vi "Main HMI.vi"() -> ()   [LabVIEW 2023]
uses:
  <instrlib>/HPS-17000/Client Facing Datatypes/Limits.ctl
  Types/Function.ctl
  Types/Mode.ctl
  Types/Range.ctl
  Types/Setpoints.ctl
  <instrlib>/HPS-17000/Client Facing Datatypes/DeviceProperties.ctl
  Types/EIS Mode.ctl
  <vilib>/HPS-17000/nibatterycycler_grpc_Setpoint.ctl
  Classes/Grapher_class/Grapher.lvclass
  Streamer_class/Streamer.lvclass
  Logger_class/Logger.lvclass
  Script_class/Script.lvclass
  <instrlib>/HPS-17000/HPS-17000.lvclass
  <instrlib>/HPS-17000/Client Facing Datatypes/Multi-Cycler Events.ctl
  <instrlib>/HPS-17000/Client Facing Datatypes/Heartbeat Event Data.ctl
  <instrlib>/HPS-17000/Client Facing Datatypes/Faults Event Data.ctl
  <instrlib>/HPS-17000/Client Facing Datatypes/Network Sync Event Data.ctl
  <instrlib>/HPS-17000/Client Facing Datatypes/Setpoint Stream Status Data.ctl
  <vilib>/HPS-17000/MStream_grpc_CyclerMeasurement.ctl
  Types/ERROR_GLOBAL.ctl
  <instrlib>/HPS-17000/Client Facing Datatypes/Range.ctl
  <vilib>/HPS-17000/Setpoint Stream Basic Config.ctl
  <vilib>/Utility/miscctls.llb/LVStringsAndValuesArrayTypeDef_I16.ctl
  <vilib>/addons/_JKI Toolkits/State Machine/_JKI_lib_State_Machine.llb/Select State(s)_err__jki_lib_state_machine.vi
  <vilib>/Utility/error.llb/Trim Whitespace One-Sided.vi
  <instrlib>/HPS-17000/Internal/Acknowledge Faults Multi.vi
  <instrlib>/HPS-17000/Internal/Identify Multi.vi
  <vilib>/Utility/TDMS File Viewer/TDMS - File Viewer (NXG Style).vi
  <instrlib>/HPS-17000/Internal/Get Status Multi.vi
  <instrlib>/HPS-17000/Internal/Get Faults Multi.vi
  <instrlib>/HPS-17000/Internal/Get Mode Multi.vi
  <instrlib>/HPS-17000/Internal/Get Limits Multi.vi
  <instrlib>/HPS-17000/Internal/Get Enabled Output Multi.vi
  <vilib>/Waveform/WDTOps.llb/WDT Append Waveforms DBL.vi
  <vilib>/Utility/file.llb/Write Delimited Spreadsheet (DBL).vi
  <instrlib>/HPS-17000/Internal/Find GM ID Single.vi
  <instrlib>/HPS-17000/Internal/Initialize Single.vi
  <instrlib>/HPS-17000/Internal/Initialize Multi.vi
  <instrlib>/HPS-17000/Internal/Close Multi.vi
  <instrlib>/HPS-17000/Internal/Reserve Multi.vi
  <instrlib>/HPS-17000/Internal/Unreserve Multi.vi
  <instrlib>/HPS-17000/Internal/Clear Reservation Multi.vi
  <instrlib>/HPS-17000/Internal/Clear Reservation Confirmation Multi.vi
  <instrlib>/HPS-17000/Internal/Write Setpoint Multi.vi
  <instrlib>/HPS-17000/Internal/Set Mode Multi.vi
  <instrlib>/HPS-17000/Internal/Set Limits Multi.vi
  <instrlib>/HPS-17000/Internal/Set Energized Multi.vi
  <instrlib>/HPS-17000/Internal/Set Enabled Output Multi.vi
  <instrlib>/HPS-17000/Internal/Start Measurement Stream Multi.vi
  <instrlib>/HPS-17000/Internal/Stop Measurement Stream Multi.vi
  <instrlib>/HPS-17000/Internal/Start Setpoint Stream Multi.vi
  <instrlib>/HPS-17000/Internal/Stream Setpoints Multi.vi
  <instrlib>/HPS-17000/Internal/Stop Setpoint Stream Multi.vi
  <vilib>/Utility/file.llb/Read Delimited Spreadsheet (DBL).vi
  <userlib>/_OpenG.lib/appcontrol/appcontrol.llb/openg_application_control.lvlib
  <vilib>/HPS-17000/NI_BC_client.lvlib
  <vilib>/HPS-17000/Cycler.lvclass
  <vilib>/measure/NI_MABase.lvlib
  <vilib>/Utility/TDMS File Viewer/NI_TDMS File Viewer.lvlib
panel:
  out "Charging 2":bool caption="CHARGE"
  out "Discharging":bool caption="DISCHARGE"
  in  "Cycler Selection":i16(ring) caption="CYCLER(S)" items=["ALL"=-1]
  out "EMO Indicator":u16(ring)
  in  "Start Logging":bool
  out "Function":T1=enum."STANDBY" caption="FUNCTION"
  out "MODE":u16(ring)=193 items=["UNKNOWN"=0, "CONSTANT VOLTAGE"=1, "CONSTANT CURRENT"=2, "INTERNAL RECIRCULATION"=193]
  in  "HPS Clear":bool
  out "Status Message":string
  in  "HPS Reserve":bool
  in  "HPS Connect":bool
  out "Fault Message":string
  in  "Acknowledge Faults":bool
  out "Current Range":string(combo) caption="RANGE"
  out "Voltage Range":string(combo) caption="RANGE"
  out "Power Maximum":sgl caption="MAX"
  out "Power Minimum":sgl caption="MIN"
  out "Current Maximum":sgl caption="MAX"
  out "Current Minimum":sgl caption="MIN"
  out "Voltage Maximum":sgl caption="MAX"
  out "Voltage Minimum":sgl caption="MIN"
  in  "Main Tab Control":T2(tab)=enum."CONTROL"
  out "XY Graph":T3(graph)
  in  "Use Local Time":bool caption="LOCAL TIME"
  in  "High Speed":bool caption="HIGH SPEED"
  in  "Pause Chart":bool
  in  "Save Chart":bool
  in  "Erase Chart":bool
  in  "TSN NIC IP Address":string caption="TSN NIC IP ADDRESS"
  in  "HPS Topology":enum16{"SINGLE", "MULTI"}(ring) caption="HPS17K TOPOLOGY"
  in  "Profile Step dT (ns)":i64=10000 caption="PROFILE STEP TIME (ns)"
  in  "Graph Samples":u32=10000 caption="CHART SAMPLES"
  in  "Graph Data Decimation":i32=100 caption="CHART DECIMATION"
  in  "Log File Directory":path caption="LOG FILE DIRECTORY"
  in  "Controller TSN IP":string caption="CONTROLLER TSN IP"
  in  "HPS17K Search":bool
  in  "Device Search":string(tree) caption="HPS17K SEARCH"
  in  "HPS17K IP Addresses":string[](tree) caption="HPS17K NETWORK"
  in  "Add HPS17K":bool
  in  "Remove HPS17K":bool
  in  "Apply Slew Rates":bool
  in  "Slew Rates":T4={"Voltage Inc. [V/sec]"=inf, "Voltage Dec. [V/sec]"=inf, "Current Inc. [A/sec]"=inf, "Current Dec. [A/sec]"=inf, "Resistance Inc. [Ohms/sec]"=inf, "Resistance Dec. [Ohms/sec]"=inf} caption="SLEW RATES"
  in  "Output":bool caption="OUTPUT"
  in  "Apply Setpoints":bool
  in  "Setpoints":T5 caption="SETPOINTS"
  in  "Apply Mode & Range":bool
  in  "Mode & Range":cluster{"Mode":T6, "Range":T7}={"Mode"=193, "Range"=1} caption="MODE | RANGE" {"Range" items=["Low Voltage"=1, "High Voltage"=2]; "Mode" items=["Constant Voltage"=1, "Constant Current"=2, "Internal Recirculation"=193]}
  in  "Apply Limits":bool
  in  "Limits":T8 caption="LIMITS"
  in  "Energize":bool caption="ENERGIZE"
  in  "TDMS Viewer":bool
  in  "Get Device Properties":bool
  in  "Get XC Report":bool
  out "Event Log":i32(listbox) caption="EVENT LOG"
  in  "Clear Event Log":bool
  in  "Volta Monitor":bool
  out "device properties":T9
  out "GM ID":string
  out "Measurement Stream":bool caption="MEASUREMENT STREAM"
  out "Setpoint Stream":bool caption="SETPOINT STREAM"
  out "OK":bool
  out "Heartbeat Valid":bool caption="HEARTBEAT VALID"
  in  "FC Sys Inspect":bool
  out "Fault Description":string caption="FAULT DESCRIPTION"
  in  "Start & Stop EIS Profile":bool
  in  "EIS AC Step Delay":dbl=1.0 caption="AC Step Delay (Seconds)"
  in  "EIS Samples":dbl=1000.0 caption="Samples at Frequency"
  in  "AC Signal (mV/mA RMS)":dbl=20.0
  in  "EIS DC Current":dbl caption="DC Current (A)"
  in  "EIS Delta Frequency":dbl=100.0 caption="AC Step Frequency (Hz)"
  in  "EIS Stop Frequency":dbl=500.0 caption="AC Stop Frequency (Hz)"
  in  "EIS Start Frequency":dbl=1000.0 caption="AC Start Frequency (Hz)"
  in  "EIS DC Potential":dbl=650.0 caption="DC Potential (V)"
  in  "EIS Mode":T10=2 items=["Voltage (PEIS)"=1, "Current (GEIS)"=2]
  in  "Generate EIS Profile":bool
  in  "EIS Save & Load Profile":bool
  in  "Generate EIS Report":bool
  in  "CSV Profile":path caption="CSV PROFILE"
  in  "Start Profile":bool
  out "CSV Profile":waveform(sgl)[](graph)
  out "Self Test Log":i32(listbox) caption="SELF TEST LOG"
  in  "Run Self Test":bool
  out "Test Server Log":i32(listbox) caption="TEST SERVER LOG"
  in  "Launch Test Server":bool
  in  "Voltage Reformation":bool caption="REFORMATION"
  in  "Update Temperatures":bool
  out "Temperatures":i32(listbox) caption="TEMPERATURES"
  out "Thermal Limits":i32(listbox) caption="THERMAL LIMITS"
  out "Hardware Limits":i32(listbox) caption="HARDWARE LIMITS"
  out "Fault":bool caption="FAULT"
  out "Output Enabled":bool caption="OUTPUT ENABLED"
  out "Output Disabled":bool caption="OUTPUT DISABLED"
  out "System Power":bool caption="SYSTEM POWER"
  out "POWER":dbl(knob) caption="Gauge" scale=150.0..-150.0
  out "CURRENT":dbl(knob) caption="Gauge" scale=480.0..-480.0
  out "VOLTAGE":dbl(knob) caption="Gauge"
  # "what if the graphs on the right were instead a subpanel of the new EIS active object class\n\nthat way it could show us the actual EIS profile, where it's at in the test, and other features.\n\nikt would need to communicate with teh main HMI to lock out the GUI but that is fine, the main HMI\n\nwould act as the object controller launching/destroying it for different EIS profiles.  This will run an automated test that will guarnatee full resolution for each EIS frequency sweep.  It will need to automate the logging functionality as well because this log file will be necessary to run the VI afterwards to generate the profile\n\nexpand the tabs to show more details, maybe show the FFT graph so we can pinpoint hte frequency peaks and see more intermediate FFT data that might help analysis (or at the very least help development)"
  # "generate eis profile will create a new object and embed it into the subpanel.  if one already exists, it willr emove it\n\nstart eis profile will start/stop the EIS profile active object active test sequence until it finishes or is stopped.  It will not\nenable this button until an EIS profile has been generated.\n\nthe user can also load a previous EIS data which will load the data into the EIS object for analysis\n\nthen, generate report wil take the newly generated (or loaded data previously generated) and then generate the nyquist, bode, and FFT plots for viewing.\n\nwe should also add a way to export this graph once it's generated\n\nneed to add teh subpanel"
  # "OFF               ON"
  # "OFF               ON"
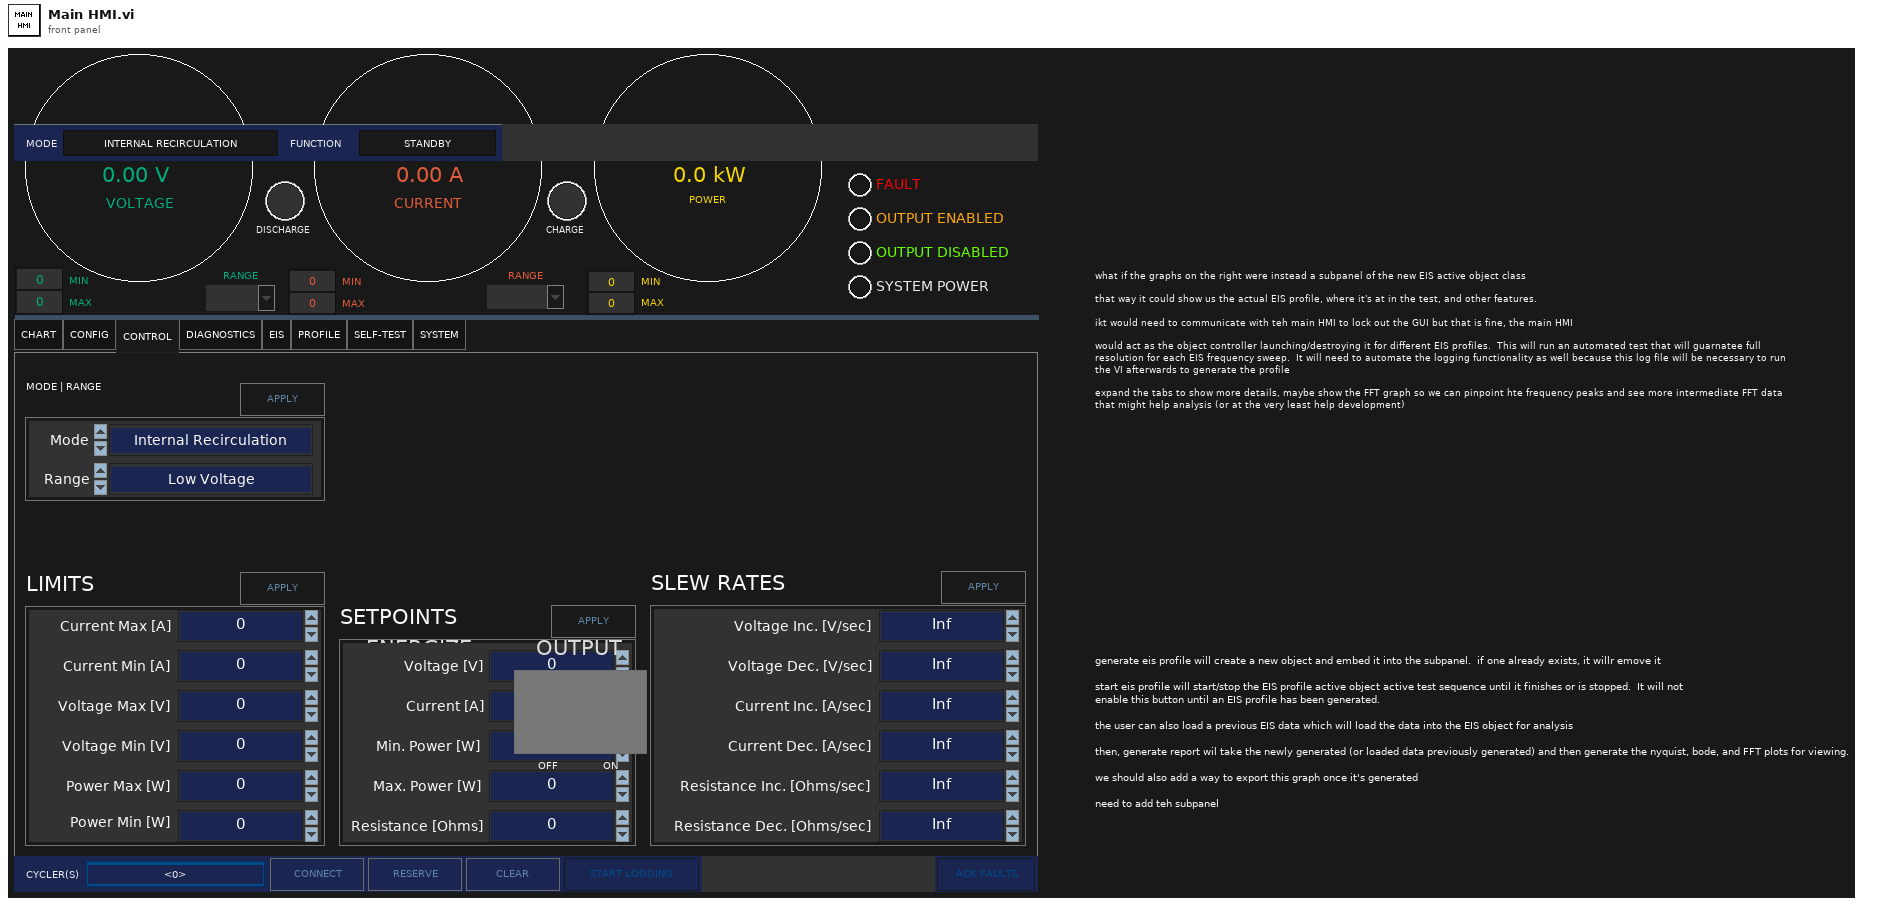
[diagram p1: front panel]
types:
  T1 = typedef "Function.ctl" = enum16{"REGEN", "STANDBY", "SUPPLY"}
  T2 = enum32{"CHART", "CONFIG", "CONTROL", "DIAGNOSTICS", "EIS", "PROFILE", "SELF-TEST", "SYSTEM"}
  T3 = cluster{"timestamp":dbl[], "setpoint current":dbl[]}[]
  T4 = cluster{"Voltage Inc. [V/sec]":sgl, "Voltage Dec. [V/sec]":sgl, "Current Inc. [A/sec]":sgl, "Current Dec. [A/sec]":sgl, "Resistance Inc. [Ohms/sec]":sgl, "Resistance Dec. [Ohms/sec]":sgl}
  T5 = typedef "Setpoints.ctl" = cluster{"Voltage":sgl, "Current":sgl, "Minimum Power":sgl, "Maximum Power":sgl, "Resistance":sgl}
  T6 = typedef "Mode.ctl" = u16
  T7 = typedef "Range.ctl" = u16
  T8 = typedef "HPS-17000.lvclass/Limits.ctl" = cluster{"Current Max Limit":sgl, "Current Min Limit":sgl, "Voltage Max Limit":sgl, "Voltage Min Limit":sgl, "Power Max Limit":sgl, "Power Min Limit":sgl}
  T9 = typedef "HPS-17000.lvclass/DeviceProperties.ctl" = cluster{"name":string, "model":string, "vendor":string, "serial_number":string}
  T10 = typedef "EIS Mode.ctl" = u16
  T11 = typedef "NI_BC_client.lvlib/nibatterycycler_grpc_Setpoint.ctl" = cluster{"voltage":sgl, "current":sgl, "min_power":sgl, "max_power":sgl, "resistance":sgl}
  T12 = typedef "HPS-17000.lvclass/Multi-Cycler Events.ctl" = cluster{"heartbeats events":refnum<user-event>[], "faults events":refnum<user-event>[], "network sync event":refnum<user-event>[], "setpoint status event":refnum<user-event>[]}
  T13 = cluster{"Core":cluster{"Current VI Reference":refnum<vi>, "Close Panel on Exit?":bool}, "Connected":bool, "Reserved":bool, "Measurement Stream":bool, "Setpoint Stream":bool, "Last Periodic Update":u32, "Profile Setpoints":T11[], "Grapher Ref":refnum<class "Grapher.lvclass">, "Streamer Ref":refnum<class "Streamer.lvclass">, "Logger Ref":refnum<class "Logger.lvclass">, "Test Server Ref":refnum<class "Script.lvclass">, "Self Test Ref":refnum<class "Script.lvclass">, "HPS17K Refs":refnum<class "HPS-17000.lvclass">[], "HPS17K Events":T12, "Self Test Completed":refnum<user-event>, "Graph Queue":refnum<queue>, "Logger Queue":refnum<queue>, "Drag Data":cluster{"data name":string, "drag data":variant}[]}
  T14 = enum8{"Enabled", "Disabled", "Disabled and Grayed Out"}
  T15 = cluster{"data name":string, "drag data":variant}[]
  T16 = enum32{"Invalid", "Standard", "Closed", "Hidden", "Minimized", "Maximized"}
  T17 = enum32{"invalid app kind", "Development System", "Run Time System", "Student Edition", "Embedded LabVIEW", "Evaluation", "Custom"}
  T18 = enum16{"open", "replace", "create", "open or create", "replace or create", "replace or create with confirmation"}
  T19 = typedef "Cycler.lvclass/Setpoint Stream Basic Config.ctl" = cluster{"local address":string, "receiver port":u16}
  T20 = cluster{"XY Graph":refnum<vi>, "Voltage":refnum<vi>, "Current":refnum<vi>, "Power":refnum<vi>, "Function":refnum<vi>}
  T21 = typedef "LVStringsAndValuesArrayTypeDef_I16.ctl" = cluster{"String":string, "Value":i16}[]
  T22 = typedef "ERROR_GLOBAL.ctl" = u32
  T23 = typedef "NI_BC_client.lvlib/MStream_grpc_CyclerMeasurement.ctl" = cluster{"measured_voltage":sgl, "measured_current":sgl, "setpoint_voltage":sgl, "setpoint_current":sgl, "timestamp":i64}
  T24 = cluster{"Current VI Reference":refnum<vi>, "Close Panel on Exit?":bool}
  T25 = typedef "HPS-17000.lvclass/Range.ctl" = u8
  T26 = typedef "HPS-17000.lvclass/Mode.ctl" = u8
  T27 = typedef "HPS-17000.lvclass/Events.ctl" = cluster{"heartbeat failure event":refnum<user-event>, "faults event":refnum<user-event>, "network sync event":refnum<user-event>, "setpoint status event":refnum<user-event>}
  T28 = cluster{"[0]":dbl, "[1]":dbl, "[2]":dbl, "[3]":dbl, "[4]":dbl, "[5]":dbl}
  T29 = cluster{"[0]":dbl, "[1]":dbl, "[2]":dbl, "[3]":dbl, "[4]":dbl}
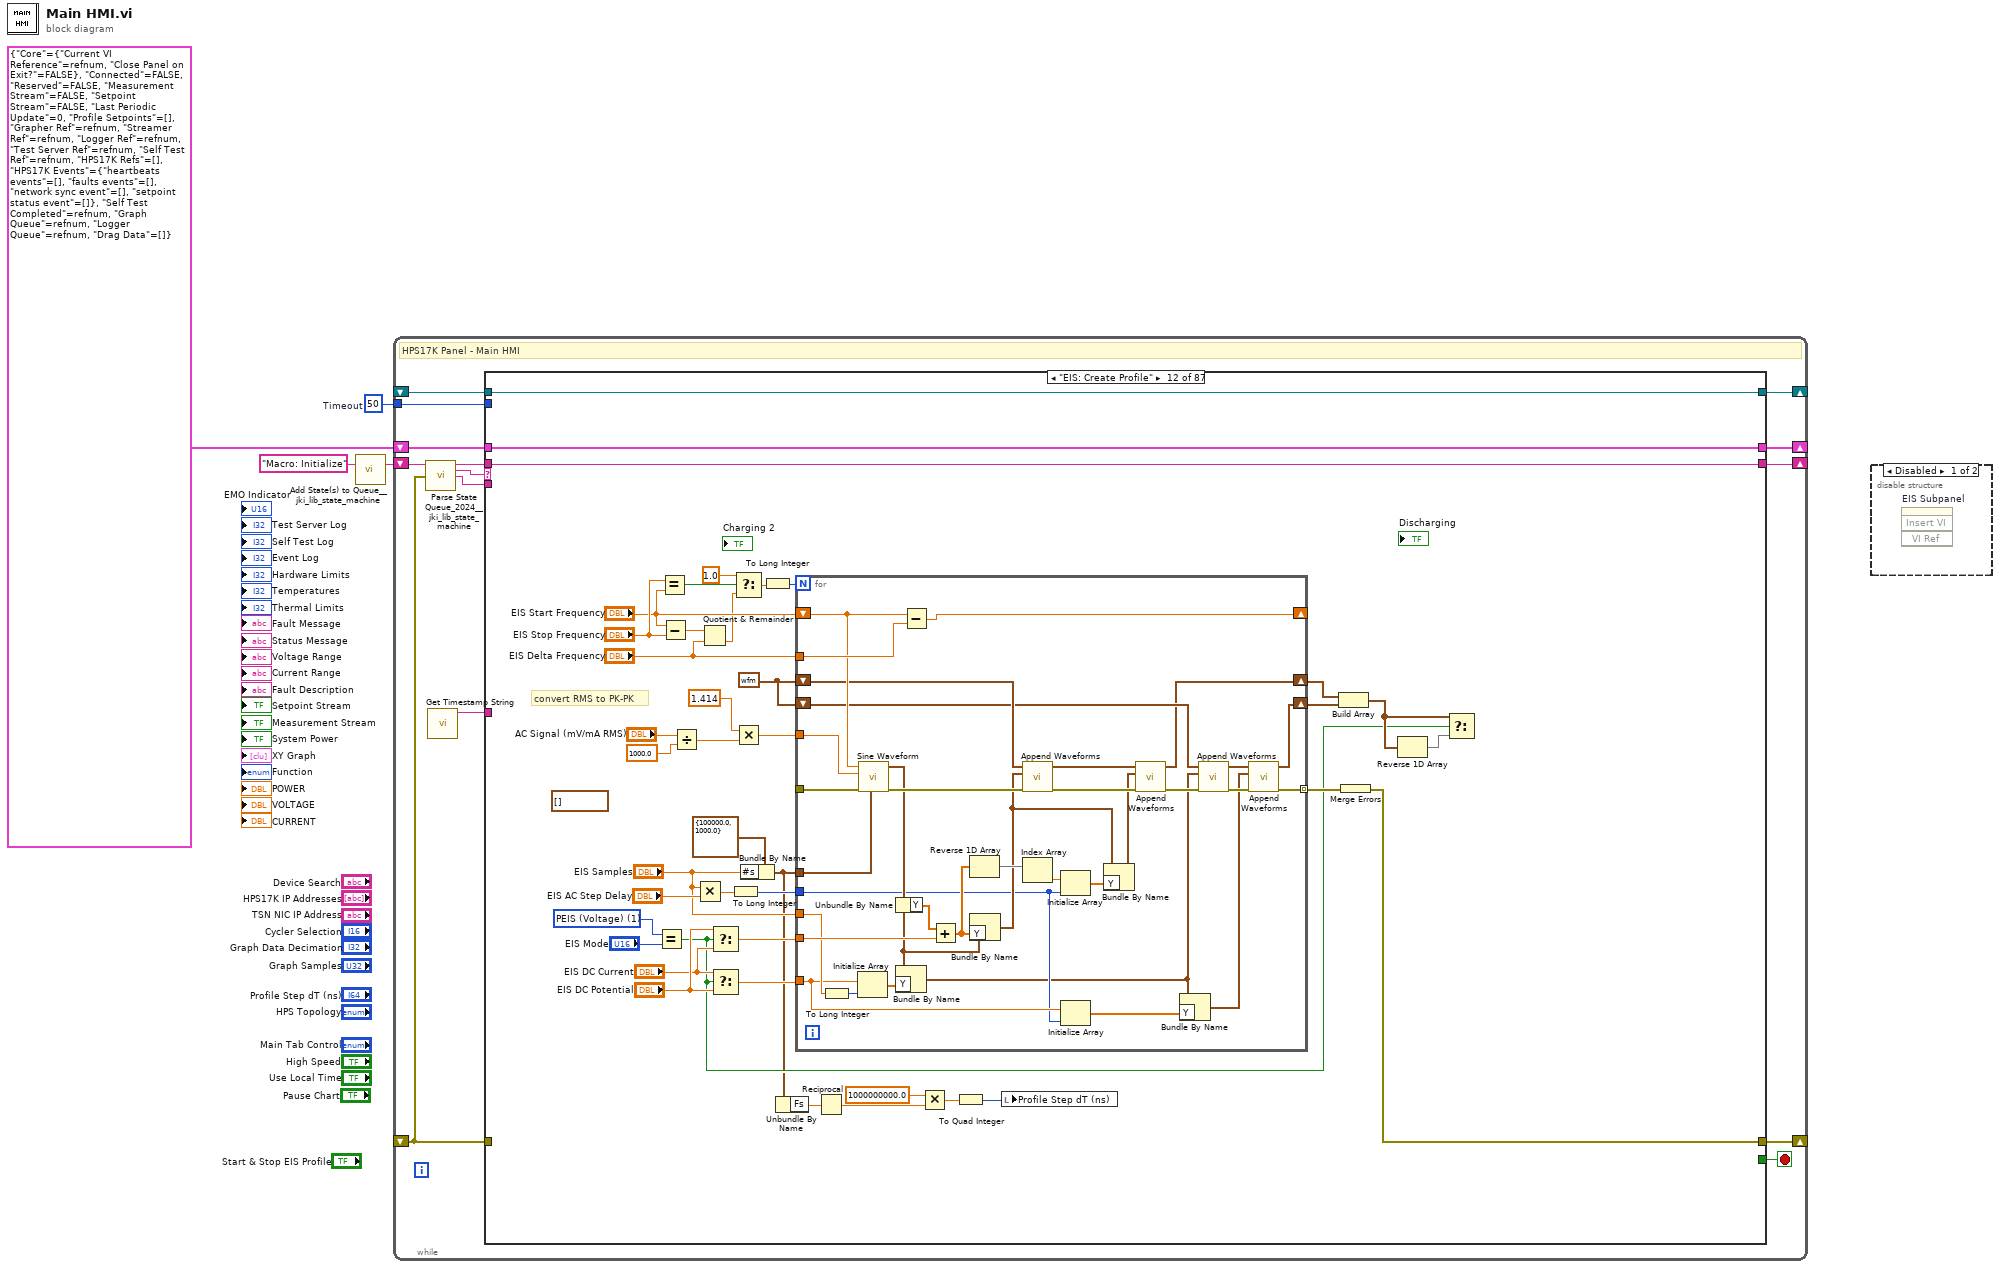
[diagram p0: block diagram]
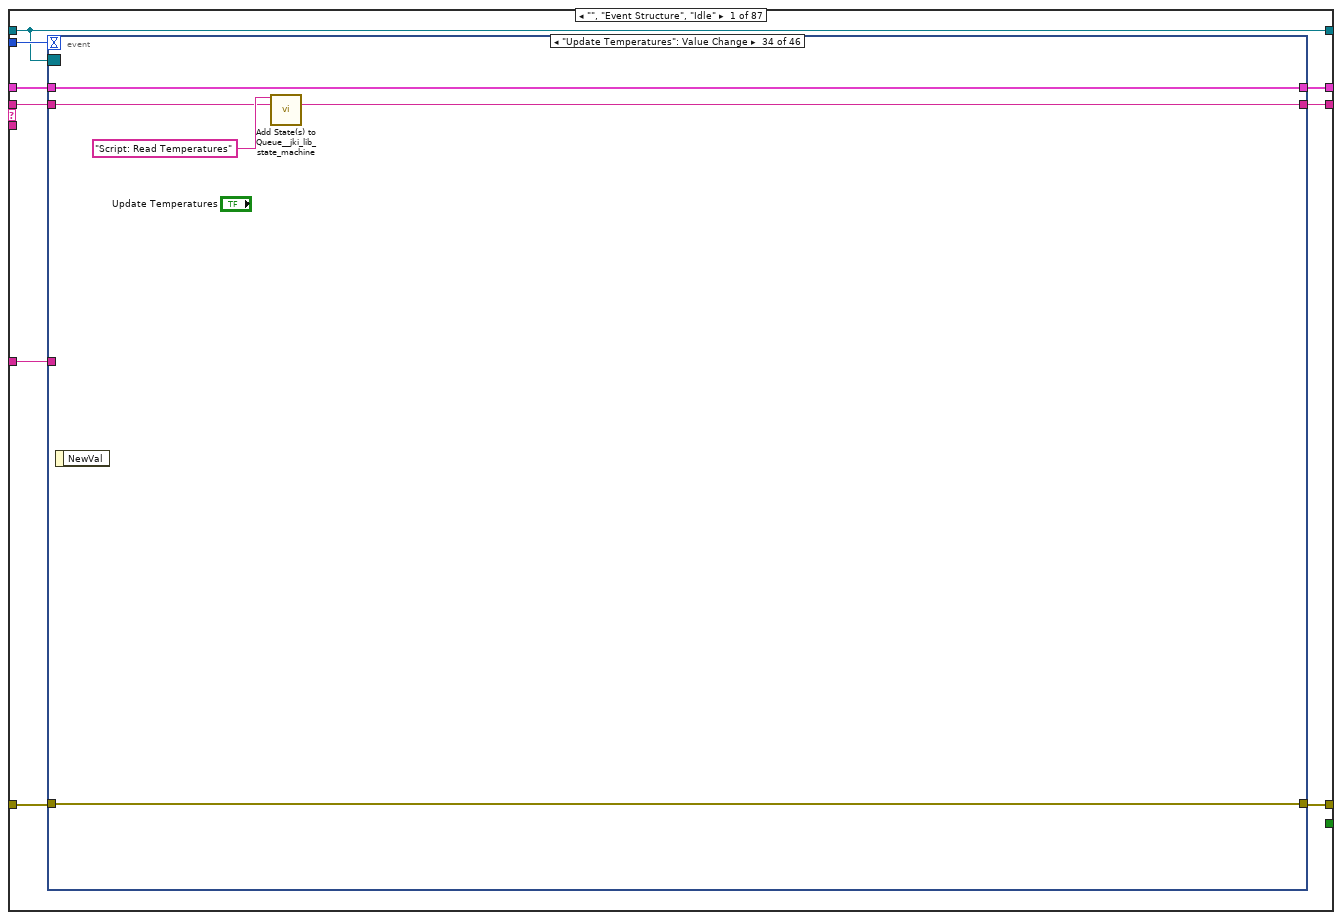
[diagram p3: hidden frame]
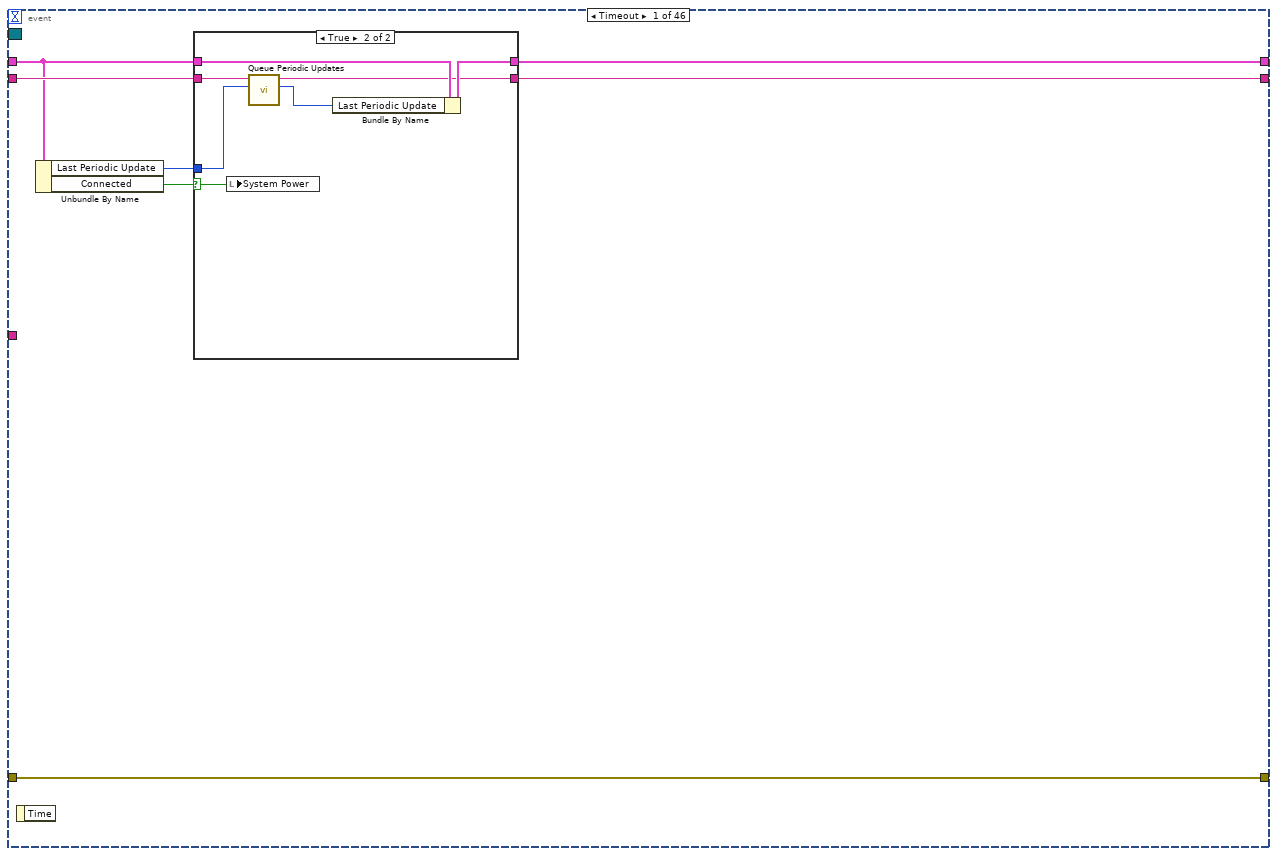
[diagram p4: hidden frame]
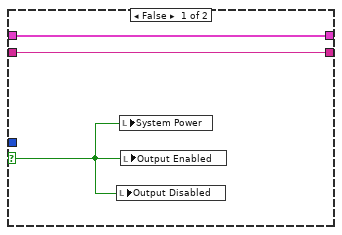
[diagram p5: hidden frame]
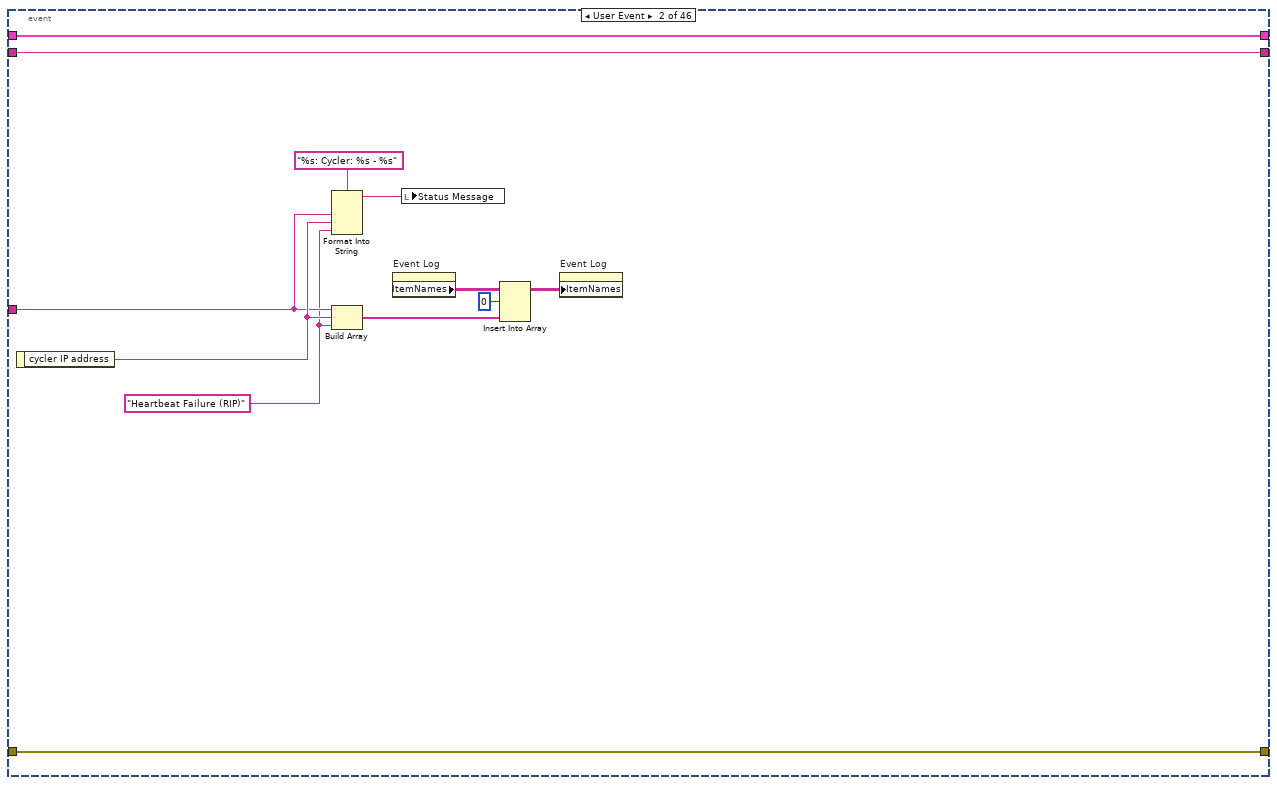
[diagram p6: hidden frame]
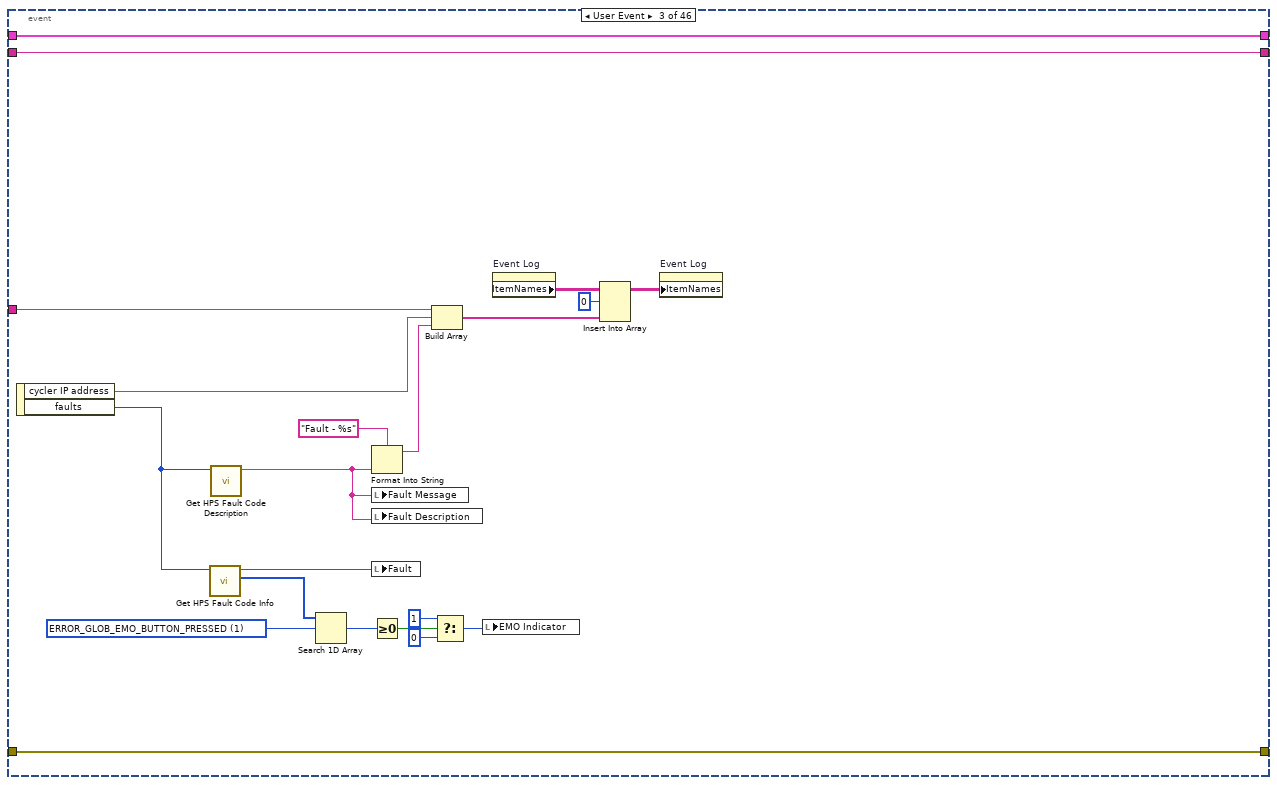
[diagram p7: hidden frame]
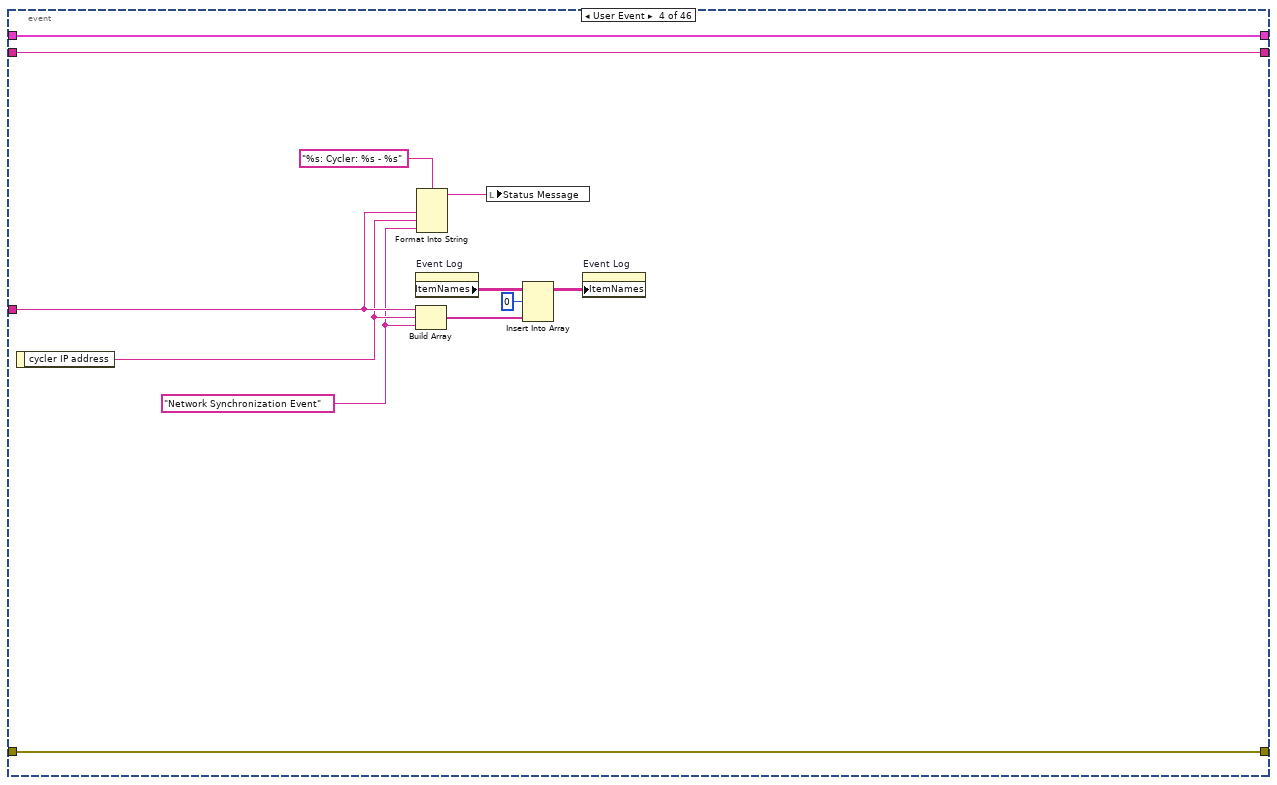
[diagram p8: hidden frame]
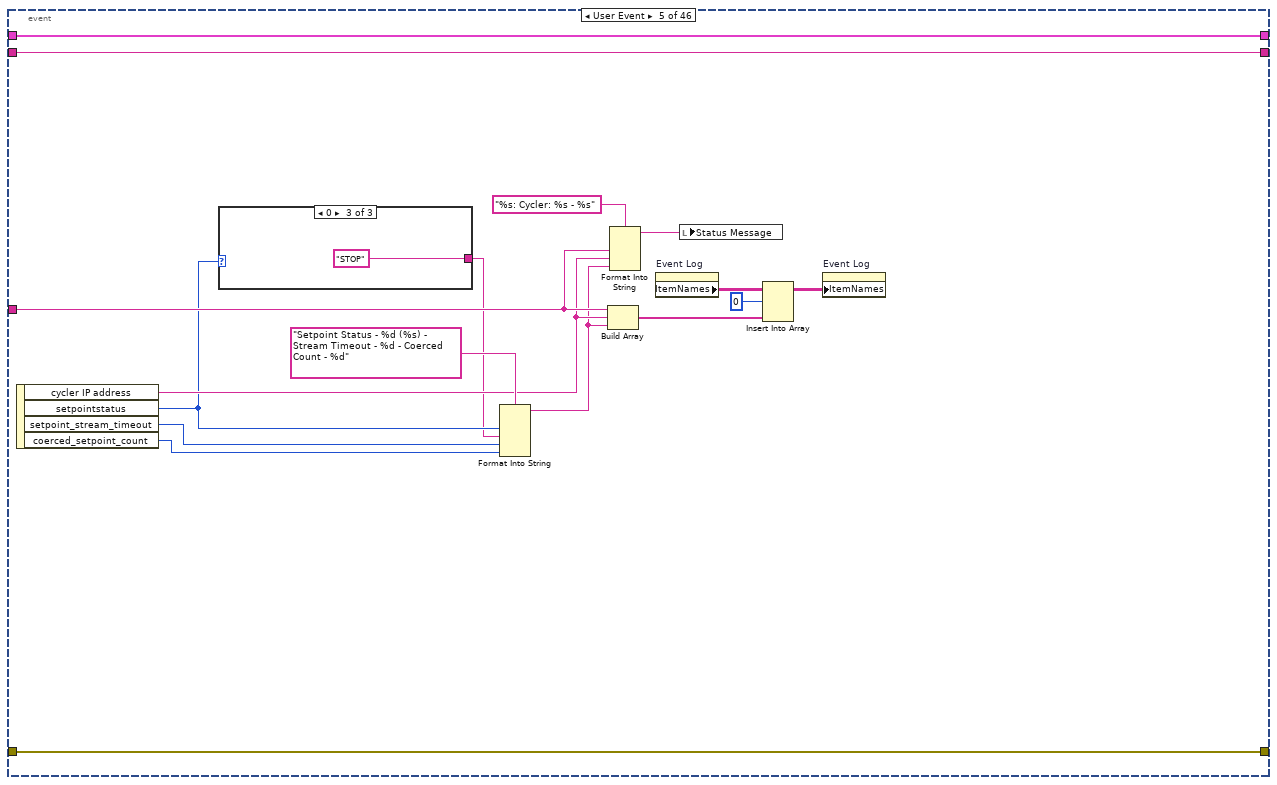
[diagram p9: hidden frame]
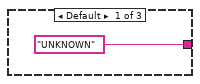
[diagram p10: hidden frame]
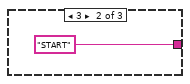
[diagram p11: hidden frame]
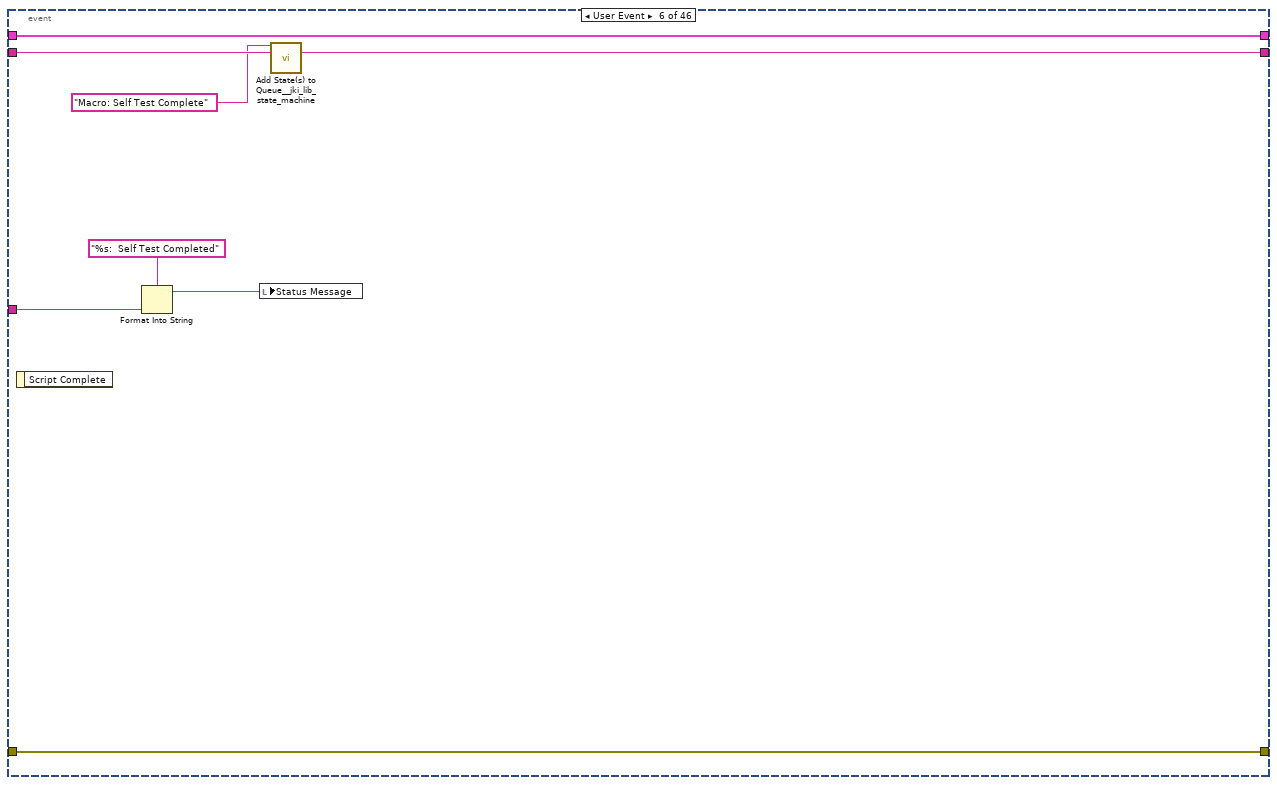
[diagram p12: hidden frame]
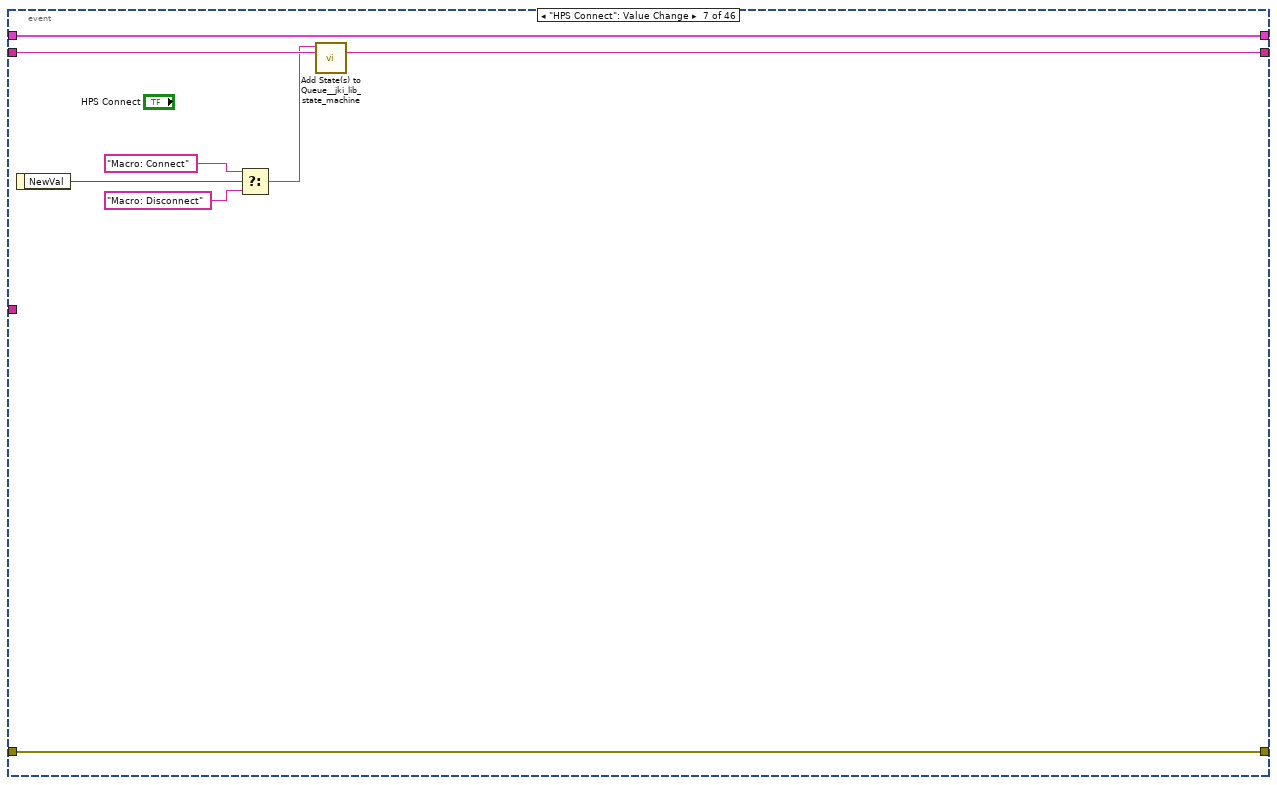
[diagram p13: hidden frame]
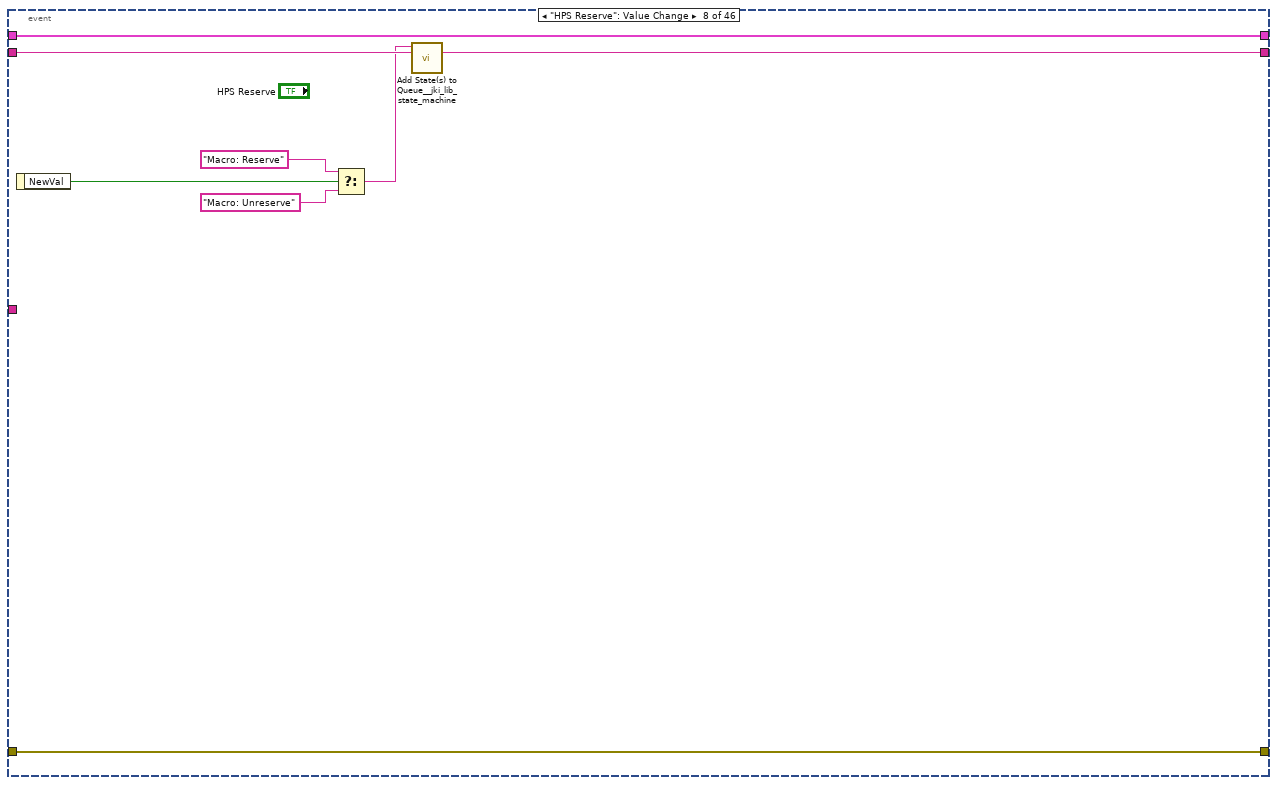
[diagram p14: hidden frame]
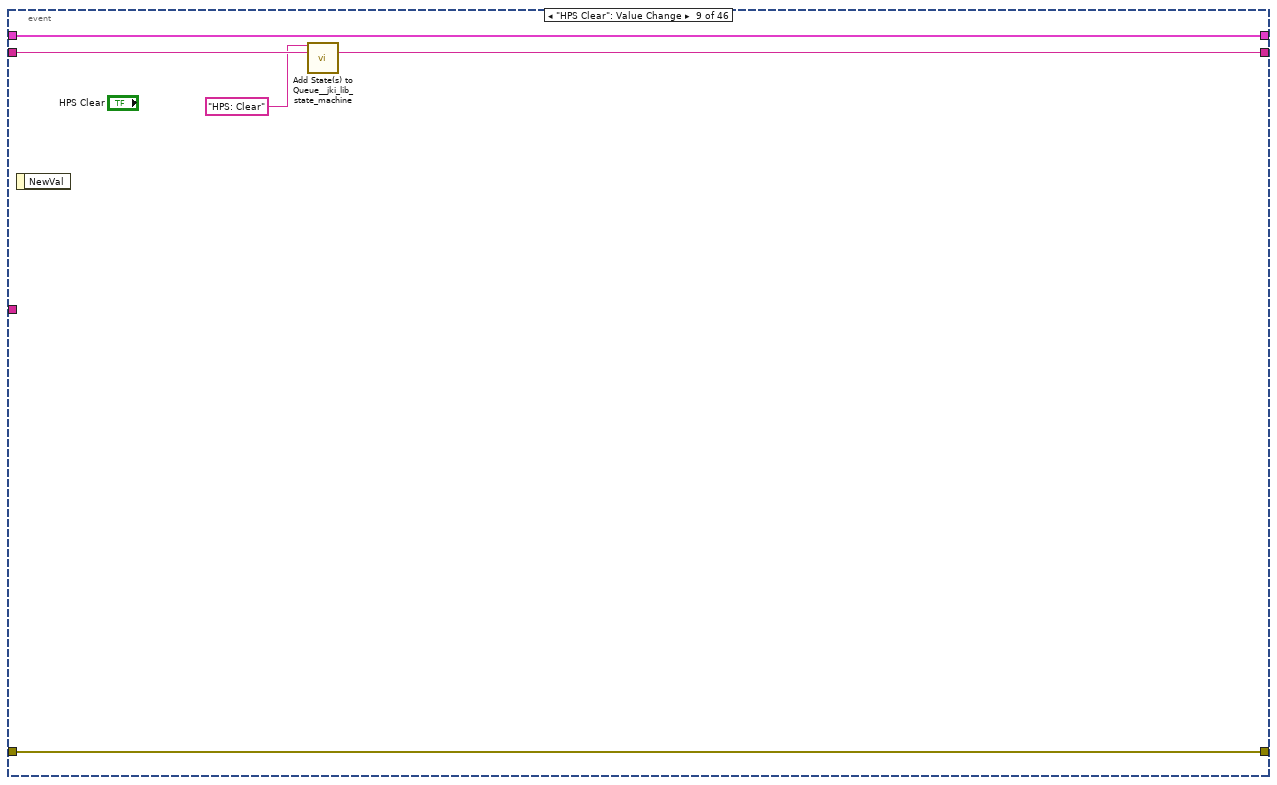
[diagram p15: hidden frame]
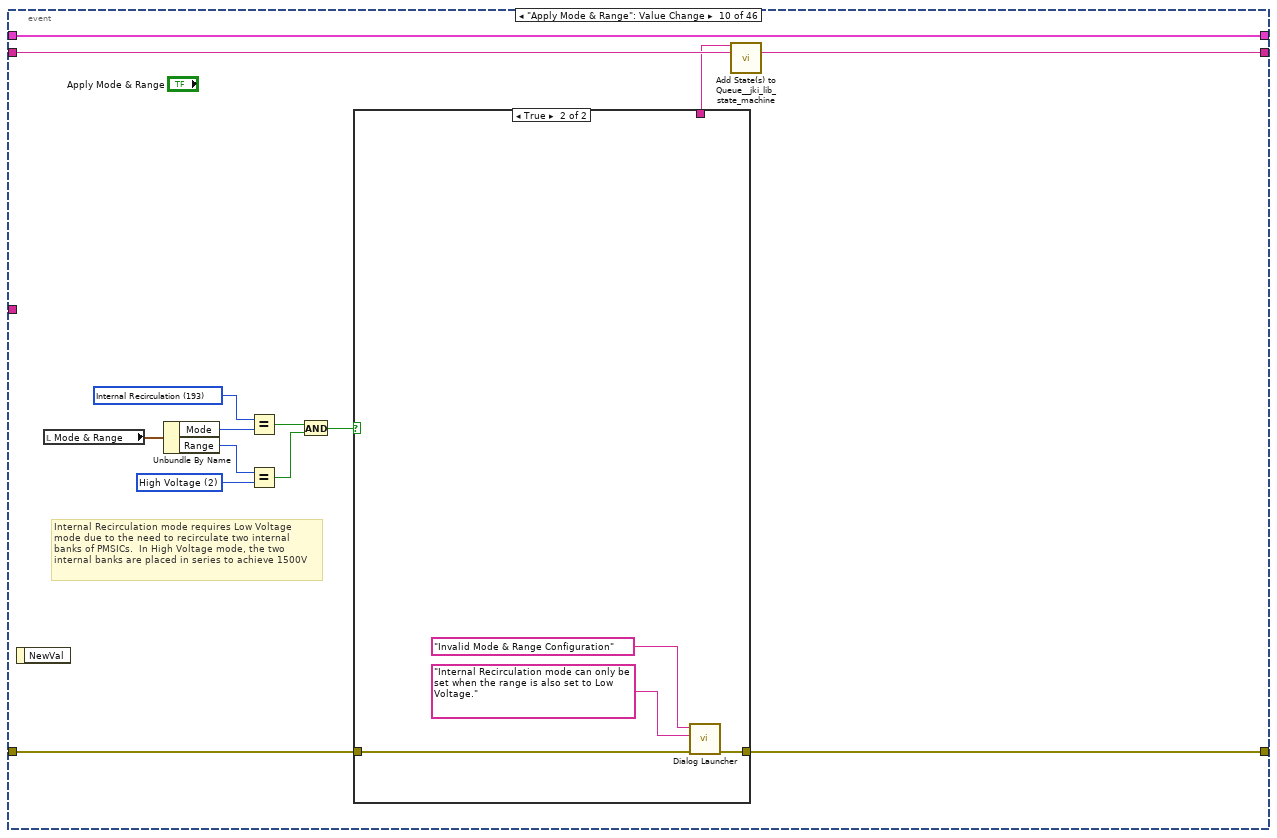
[diagram p16: hidden frame]
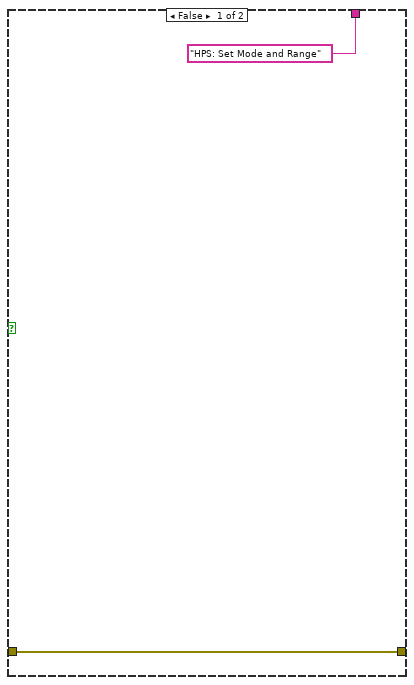
[diagram p17: hidden frame]
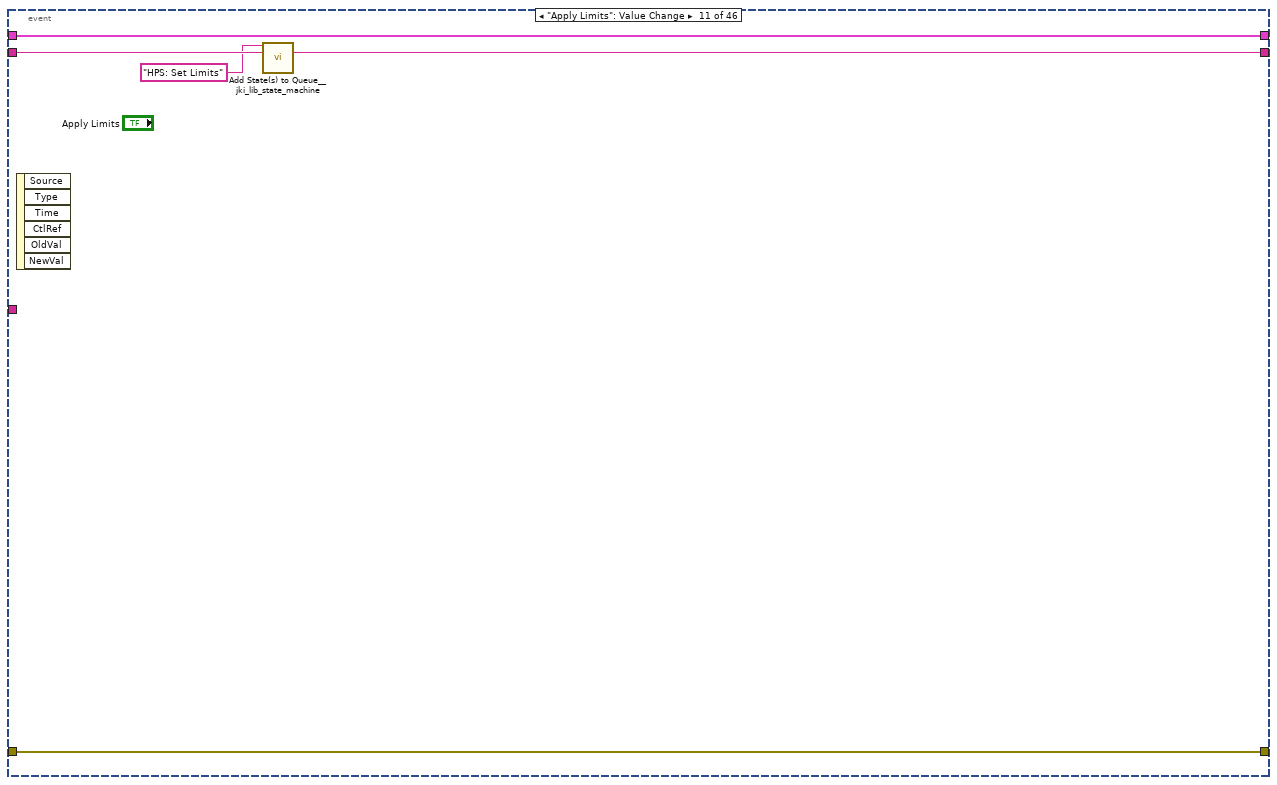
[diagram p18: hidden frame]
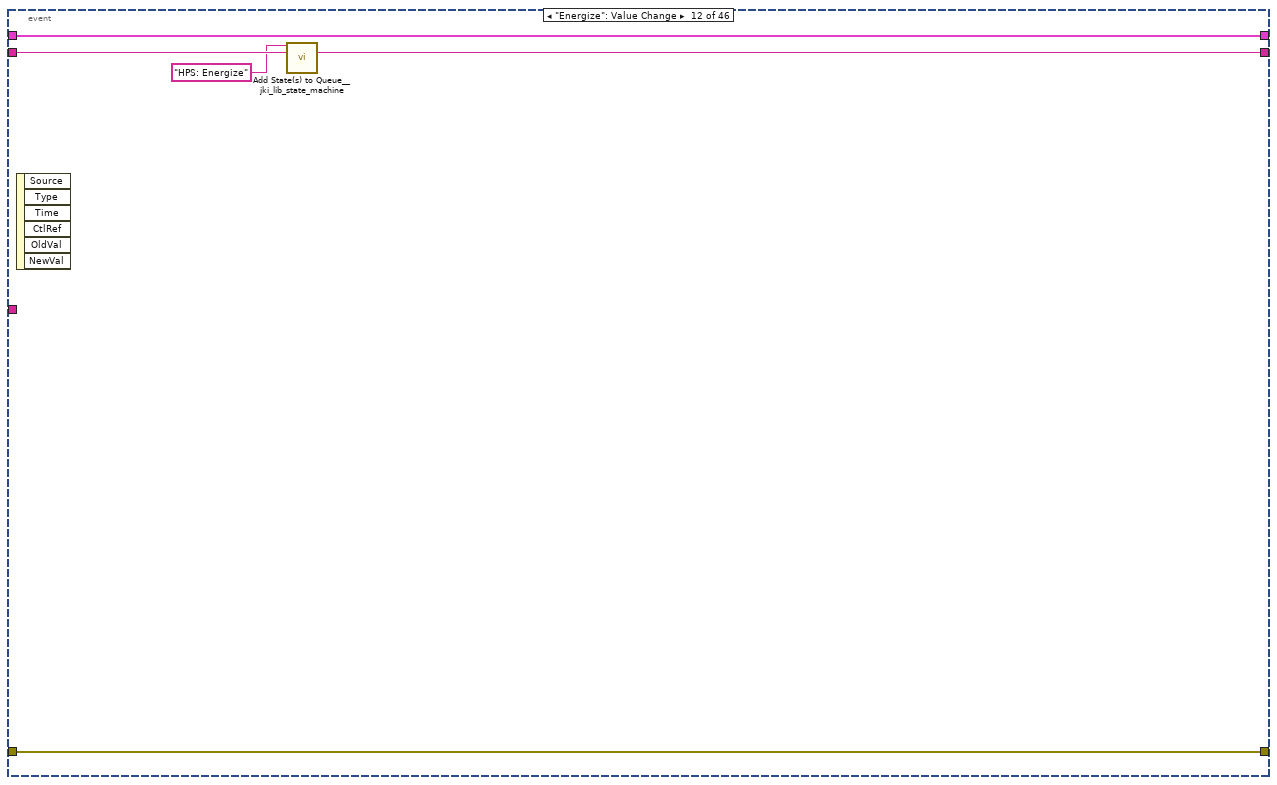
[diagram p19: hidden frame]
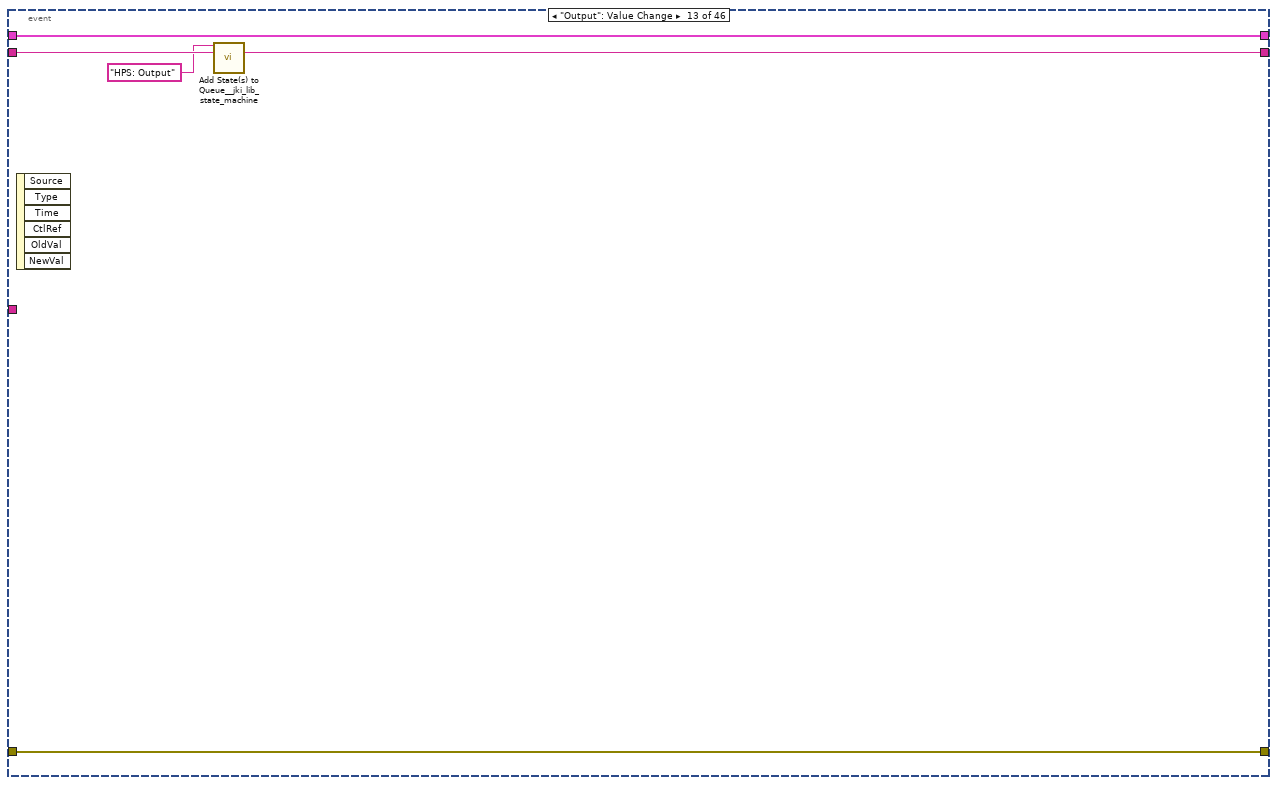
[diagram p20: hidden frame]
diagram:
  w2 = 50  # Timeout
  n1 = call <vilib>:"Add State(s) to Queue__jki_lib_state_machine.vi"("State(s) in (\"\")"="Macro: Initialize") -> ("States Out"=w4:string)  [unwired: 14 in]
  n2 = while "JKI State Machine 2024" {
    shift-right: [w12] -> _
    shift-left: T13 {"Core"={"Current VI Reference"=refnum, "Close Panel on Exit?"=FALSE}, "Connected"=FALSE, "Reserved"=FALSE, "Measurement Stream"=FALSE, "Setpoint Stream"=FALSE, "Last Periodic Update"=0, "Profile Setpoints"=[], "Grapher Ref"=refnum, "Streamer Ref"=refnum, "Logger Ref"=refnum, "Test Server Ref"=refnum, "Self Test Ref"=refnum, "HPS17K Refs"=[], "HPS17K Events"={"heartbeats events"=[], "faults events"=[], "network sync event"=[], "setpoint status event"=[]}, "Self Test Completed"=refnum, "Graph Queue"=refnum, "Logger Queue"=refnum, "Drag Data"=[]} -> [w11]
    shift-right: [w14] -> _
    shift-left: _ -> [w10]
    shift-right: [w6] -> _
    shift-left: w4 -> [w15]
    tunnel: w2 -> [w9]
    shift-right: [w8] -> _
    shift-left: _ -> [w7]
    stop <- w13 stop-if-true
    # "HPS17K Panel - Main HMI"
    n3 = call <vilib>:"Parse State Queue_2024__jki_lib_state_machine.vi"("State Queue"=w15, "Error In (no error)"=w10) -> ("Remaining States"=w17:string, "Current State"=w18:string, "Arguments"=w16:string)  [unwired: 11 in]
    n4 = call "Get Timestamp String.vi"() -> ("date/time string"=w5:string)  [unwired: 11 in]
    n5 = case shown="\"EIS: Create Profile\"" w18 {
      selector: w18 -> [_ _ w473 _ _ _ _ _ _ _ _ _ _ _ _ _ _ _ _ _ _ _ _ _ _ _ _ _ _ _ _ _ _ _ _ _ _ _ _ _ _ _ _ _ _ _ _ _ _ _ _ _ _ _ _ _ _ _ _ _ _ _ _ _ _ _ _ _ _ _ _ _ _ _ _ _ _ _ _ _ _ _ _ _ _ _ _]
      tunnel: w17 -> [w27 w471 w477 w500 w511 w521 w526 w543 w558 w573 w630 w631 w712 w765 w775 w781 w841 w856 w889 w900 w910 w942 w961 w977 w993 w1014 w1043 w1057 w1090 w1118 w1134 w1168 w1179 w1235 w1239 w1251 w1273 w1295 w1321 w1356 w1375 w1393 w1420 w1453 w1486 w1518 w1550 w1582 w1607 w1621 w1656 w1678 w1695 w1723 w1734 w1741 w1746 w1750 w1777 w1781 w1787 w1788 w1803 w1827 w1839 w1846 w1853 w1860 w1867 w1878 w1947 w1953 w1960 w1966 w1972 w1984 w1990 w1996 w2002 w2008 w2014 w2020 w2026 w2032 w2038 w2059 w2069]
      tunnel: w16 -> [_ _ _ _ w506 _ _ _ _ _ _ _ _ _ _ _ _ _ _ _ _ _ _ _ _ _ _ _ _ _ _ _ _ _ _ _ _ _ _ _ _ _ _ _ _ _ _ _ _ _ _ _ _ _ _ _ _ _ _ _ _ _ _ _ _ _ _ _ w1863 w1873 _ _ _ _ _ _ _ _ _ _ _ _ _ _ _ _ _]
      tunnel: w11 -> [w25 w468 w475 w494 w508 w516 w523 w540 w556 w570 w627 w632 w722 w764 w772 w800 w838 w862 w887 w898 w908 w939 w958 w975 w991 w1003 w1041 w1060 w1088 w1108 w1131 w1166 w1169 w1233 w1237 w1247 w1269 w1291 w1316 w1357 w1374 w1392 w1419 w1452 w1485 w1517 w1549 w1581 w1603 w1623 w1659 w1674 w1691 w1719 w1732 w1738 w1745 w1748 w1776 w1780 w1786 w1793 w1802 w1826 w1838 w1845 w1852 w1859 w1866 w1875 w1945 w1950 w1957 w1963 w1968 w1980 w1986 w1992 w1998 w2004 w2010 w2016 w2022 w2028 w2035 w2055 w2067]
      tunnel: [w24 w469 w479 w484 errorcluster {"status"=FALSE, "code"=0, "source"=""} ("error out") w517 w524 w534 w544 w567 w628 w670 w713 w761 w773 w791 w835 w859 w882 w891 w906 w936 w955 w972 w988 w1010 w1038 w1066 w1085 w1114 w1136 w1167 w1173 w1231 w1238 w1248 w1270 w1292 w1319 w1354 w1368 w1390 w1417 w1450 w1483 w1515 w1547 w1579 w1605 w1626 w1661 w1676 w1693 w1721 w1733 w1739 w1742 w1749 w1773 w1779 w1785 w1792 w1801 w1825 w1840 w1847 w1854 w1861 w1864 w1876 w1946 w1951 w1958 w1964 w1970 w1982 w1988 w1994 w2000 w2006 w2012 w2018 w2024 w2030 w2036 w2057 w2060] -> w14
      tunnel: w10 -> [w21 w469 w478 w485 w507 w517 w524 w538 w549 w568 w628 w664 w720 w762 w773 w785 w840 w864 w885 w896 w902 w937 w956 w973 w989 w1011 w1039 w1067 w1086 w1115 w1137 w1167 w1177 w1231 w1238 w1249 w1271 w1293 w1320 w1355 w1369 w1391 w1418 w1451 w1484 w1516 w1548 w1580 w1606 w1627 w1662 w1677 w1694 w1722 w1733 w1736 w1743 w1749 w1774 w1779 w1785 w1792 w1801 w1825 w1840 w1847 w1854 w1861 w1865 w1877 w1946 w1951 w1958 w1964 w1970 w1982 w1988 w1994 w2000 w2006 w2012 w2018 w2024 w2030 w2036 w2057 w2060]
      tunnel: [w26 w470 w476 w499 w510 w520 w525 w542 w557 w573 w629 w631 w711 w765 w774 w780 w841 w854 w889 w900 w910 w941 w960 w977 w993 w1014 w1043 w1057 w1090 w1118 w1134 w1168 w1179 w1235 w1239 w1251 w1273 w1295 w1321 w1356 w1375 w1393 w1420 w1453 w1486 w1518 w1550 w1582 w1607 w1621 w1656 w1678 w1695 w1723 w1734 w1741 w1746 w1750 w1777 w1781 w1787 w1788 w1803 w1827 w1839 w1846 w1853 w1860 w1867 w1878 w1947 w1952 w1959 w1965 w1971 w1983 w1989 w1995 w2001 w2007 w2013 w2019 w2025 w2031 w2037 w2058 w2068] -> w6
      tunnel: [_ _ _ _ _ TRUE _ _ _ _ _ _ _ _ _ _ _ _ _ _ _ _ _ _ _ _ _ _ _ _ _ _ _ _ _ _ _ _ _ _ _ _ _ _ _ _ _ _ _ _ _ _ _ _ _ _ _ _ _ _ _ _ _ _ _ _ _ _ _ _ _ _ _ _ _ _ _ _ _ _ _ _ _ _ _ _ _] -> w13
      tunnel: [w23 w468 w475 w498 w508 w516 w523 w540 w554 w570 w627 w632 w722 w764 w772 w799 w839 w861 w886 w897 w907 w938 w957 w974 w990 w1012 w1040 w1068 w1087 w1116 w1131 w1166 w1170 w1232 w1237 w1246 w1268 w1290 w1318 w1357 w1374 w1392 w1419 w1452 w1485 w1517 w1549 w1581 w1604 w1625 w1660 w1675 w1692 w1720 w1732 w1738 w1745 w1748 w1776 w1780 w1786 w1793 w1802 w1826 w1838 w1845 w1852 w1859 w1866 w1875 w1945 w1950 w1957 w1963 w1968 w1980 w1986 w1992 w1998 w2004 w2010 w2016 w2022 w2028 w2035 w2055 w2067] -> w12
      tunnel: w9 -> [w22 _ _ _ _ _ _ _ _ _ _ _ _ _ _ _ _ _ _ _ _ _ _ _ _ _ _ _ _ _ _ _ _ _ _ _ _ _ _ _ _ _ _ _ _ _ _ _ _ _ _ _ _ _ _ _ _ _ _ _ _ _ _ _ _ _ _ _ _ _ _ _ _ _ _ _ _ _ _ _ _ _ _ _ _ _ _]
      tunnel: [w20 w467 w472 w488 w501 w518 w522 w539 w553 w572 w626 w676 w721 w763 w771 w797 w836 w865 w888 w899 w909 w940 w959 w976 w992 w1013 w1042 w1069 w1089 w1117 w1132 w1165 w1178 w1234 w1236 w1250 w1272 w1294 w1322 w1358 w1376 w1394 w1421 w1454 w1487 w1519 w1551 w1583 w1608 w1628 w1663 w1679 w1696 w1724 w1731 w1740 w1744 w1747 w1775 w1778 w1784 w1791 w1800 w1824 w1837 w1844 w1851 w1858 w1862 w1872 w1944 w1948 w1955 w1961 w1969 w1981 w1987 w1993 w1999 w2005 w2011 w2017 w2023 w2029 w2033 w2056 w2061] -> w8
      tunnel: w7 -> [w20 w467 w472 w488 w501 w518 w522 w539 w553 w572 w626 w676 w721 w763 w771 w797 w836 w865 w888 w899 w909 w940 w959 w976 w992 w1013 w1042 w1069 w1089 w1117 w1132 w1165 w1178 w1234 w1236 w1250 w1272 w1294 w1322 w1358 w1376 w1394 w1421 w1454 w1487 w1519 w1551 w1583 w1608 w1628 w1663 w1679 w1696 w1724 w1731 _ w1744 w1747 w1775 w1778 w1784 w1791 w1800 w1824 w1837 w1844 w1851 w1858 w1862 w1872 w1944 w1948 w1955 w1961 w1969 w1981 w1987 w1993 w1999 w2005 w2011 w2017 w2023 w2029 w2033 w2056 w2061]
      tunnel: w5 -> [w19 _ _ _ _ _ _ _ _ _ _ _ _ _ _ _ _ _ _ _ _ _ _ _ _ _ _ w1054 _ _ _ _ _ _ _ _ _ _ _ w1341 w1359 w1377 w1404 w1437 w1470 w1503 w1535 w1567 _ _ _ _ w1686 _ _ _ _ _ _ _ _ _ _ _ w1834 w1841 w1848 w1855 _ _ _ _ _ _ _ _ _ _ _ _ _ _ _ _ _ _ _]
      frame "", "Event Structure", "Idle" {
        n6 = event shown="[33] \"Update Temperatures\": Value Change" {
          selector: w20 -> [_ _ _ _ _ _ _ _ _ _ _ _ _ _ _ _ _ _ _ _ _ _ _ _ _ _ _ _ _ _ _ _ _ _ _ _ _ _ _ _ _ _ _ _ _ _]
          dyn-events: _ -> [_ _ _ _ _ _ _ _ _ _ _ _ _ _ _ _ _ _ _ _ _ _ _ _ _ _ _ _ _ _ _ _ _ _ _ _ _ _ _ _ _ _ _ _ _ _]
          timeout: w22 -> [_ _ _ _ _ _ _ _ _ _ _ _ _ _ _ _ _ _ _ _ _ _ _ _ _ _ _ _ _ _ _ _ _ _ _ _ _ _ _ _ _ _ _ _ _ _]
          tunnel: w27 -> [w34 w56 w77 w89 w90 w115 w123 w131 w136 w151 w161 w166 w171 w176 w184 w199 w205 w209 w214 w219 w233 w246 w254 w260 w266 w272 w278 w299 w306 w310 w315 w320 w325 w329 w338 w346 w354 w357 w362 w369 w375 w382 w402 w420 w441 w461]
          tunnel: [w33 w56 w77 w89 w90 w114 w122 w130 w135 w150 w160 w165 w170 w174 w184 w199 w204 w208 w213 w218 w232 w245 w254 w260 w266 w272 w278 w299 w304 w309 w314 w319 w324 w331 w339 w346 w354 w355 w360 w369 w375 w382 w401 w420 w441 w460] -> w26
          tunnel: w25 -> [w32 w54 w75 w87 w105 w116 w125 w133 w138 w152 w162 w167 w172 w177 w181 w197 w206 w211 w216 w221 w234 w247 w253 w259 w265 w271 w275 w298 w307 w312 w317 w322 w327 w332 w340 w343 w352 w358 w363 w366 w371 w381 w400 w417 w437 w455]
          tunnel: [w29 w55 w76 w88 w106 w117 w124 w132 w137 w147 w163 w168 w173 w178 w182 w198 w207 w212 w217 w222 w235 w248 w249 w257 w261 w269 w276 w290 w308 w313 w318 w323 w328 w333 w341 w344 w353 w359 w364 w367 w372 w378 w404 w419 w421 w459] -> w24
          tunnel: w21 -> [w29 w55 w76 w88 w106 w117 w124 w132 w137 w148 w163 w168 w173 w178 w183 w198 w207 w212 w217 w222 w235 w248 w251 w258 w264 w270 w277 w296 w308 w313 w318 w323 w328 w333 w341 w345 w353 w359 w364 w368 w374 w380 w404 w419 w430 w459]
          tunnel: [w31 w54 w75 w87 w105 w116 w125 w133 w138 w152 w162 w167 w172 w177 w181 w197 w206 w211 w216 w221 w234 w247 w253 w259 w265 w271 w275 w298 w307 w312 w317 w322 w327 w332 w340 w343 w352 w358 w363 w366 w371 w381 w399 w416 w439 w455] -> w23
          tunnel: w19 -> [_ w46 w57 w80 w97 w110 _ _ _ _ _ _ _ _ _ _ _ _ _ _ w227 w237 _ _ _ _ _ _ _ _ _ _ _ _ _ _ _ _ _ _ _ _ _ _ _ _]
          event Timeout {
            n7 = event-data() -> ()  [unwired: 1 in, 1 out]
            n8 = Unbundle By Name(w32) -> ("Last Periodic Update"=w28:u32, "Connected"=w30:bool)
            n9 = case shown="True" w30 {
              selector: w30 -> [w35 w42]
              tunnel: w34 -> [w37 w41]
              tunnel: [w37 w40] -> w33
              tunnel: w32 -> [w36 w44]
              tunnel: [w36 w43] -> w31
              tunnel: w28 -> [_ w39]
              frame False {
                n10 = local write "Output Disabled"(w35) -> ()
                n11 = local write "System Power"(w35) -> ()
                n12 = local write "Output Enabled"(w35) -> ()
              }
              frame True {
                n13 = local write "System Power"(w42) -> ()
                n14 = call "Queue Periodic Updates.vi"("Last Periodic Update in"=w39, "Remaining States"=w41) -> ("Last Periodic Update out"=w38:u32, "States Out"=w40:string)  [unwired: 8 in]
                n15 = Bundle By Name(cluster=w44, "Last Periodic Update"=w38) -> (w43:T13)
              }
            }
          }
          event User Event {
            w45 = "Heartbeat Failure (RIP)" ("format string")
            n16 = event-data() -> ("cycler IP address"=w48:string)  [unwired: 1 in]
            n17 = Format Into String(format string="%s: Cycler: %s - %s", w46, w48, w45) -> (resulting string=w47:string)  [unwired: 2 in, 1 out]
            n18 = Build Array(w46, w48, w45) -> (w51:string[])
            n19 = property on="Event Log" class="MCListbox (strict)"() -> ("ItemNames"=w53:string[][])  [unwired: 2 in, 2 out]
            n20 = local write "Status Message"(w47) -> ()
            n21 = Insert Into Array(array=w53, index (row)=0, new element=w51) -> (w52:string[][])  [unwired: 1 in]
            n22 = property on="Event Log" class="MCListbox (strict)"("ItemNames"=w52) -> ()  [unwired: 2 in, 2 out]
          }
          event User Event {
            w60 = T22 1 items=["ERROR_GLOB_EMO_GLOBAL"=0, "ERROR_GLOB_EMO_BUTTON_PRESSED"=1, "ERROR_GLOB_USER"=2, "ERROR_GLOB_PM"=3, "ERROR_GLOB_GRID"=4, "ERROR_GLOB_VOLTAGE_DCBUS_OUT_OF_BOUNDS"=6, "ERROR_GLOB_VOLTAGE_OUTPUT_HIGH"=7, "ERROR_GLOB_VOLTAGE_OUTPUT_LOW"=8, "ERROR_GLOB_VOLTAGE_OUTPUT_UNBALANCE"=9, "ERROR_GLOB_CURRENT_OUTPUT_HIGH"=10, "ERROR_GLOB_SYS_OVERTEMPERATURE"=13, "ERROR_GLOB_SYS_HW"=14, "ERROR_GLOB_SYS_COMM"=15, "ERROR_GLOB_SYNC_AND_CONNECT"=16, "ERROR_GLOB_SP"=20, "ERROR_GLOB_SP_TRACKING"=21, "ERROR_GLOB_CONFIG"=23, "ERROR_GLOB_REG_SYS"=27, "ERROR_GLOB_REG_GRID"=28, "ERROR_GLOB_REG_AFE1"=29, "ERROR_GLOB_REG_AFE2"=30, "ERROR_GLOB_REG_DC"=31] ("element")
            n23 = event-data() -> ("cycler IP address"=w71:string, "faults"=w62:u64)  [unwired: 1 in]
            n24 = call "Get HPS Fault Code Info.vi"("fault code"=w62) -> ("fault enums"=w61:T22[], "is fault?"=w58:bool)  [unwired: 8 in, 1 out]
            n25 = call "Get HPS Fault Code Description.vi"("fault code"=w62) -> ("fault description"=w59:string)  [unwired: 10 in]
            n26 = Search 1D Array(1D array=w61, element=w60) -> (index of element=w67:i32)  [unwired: 1 in]
            n27 = Format Into String(format string="Fault - %s", w59) -> (resulting string=w70:string)  [unwired: 2 in, 1 out]
            n28 = local write "Fault Message"(w59) -> ()
            n29 = local write "Fault Description"(w59) -> ()
            n30 = local write "Fault"(w58) -> ()
            n31 = Greater Or Equal To 0?(x=w67) -> (x >= 0?=w66:bool)
            n32 = Build Array(w57, w71, w70) -> (w68:string[])
            n33 = Select(t=u16 1, s=w66, f=u16 0 ("EMO Indicator")) -> (s? t:f=w63:u16)
            n34 = local write "EMO Indicator"(w63) -> ()
            n35 = property on="Event Log" class="MCListbox (strict)"() -> ("ItemNames"=w74:string[][])  [unwired: 2 in, 2 out]
            n36 = Insert Into Array(array=w74, index (row)=0, new element=w68) -> (w73:string[][])  [unwired: 1 in]
            n37 = property on="Event Log" class="MCListbox (strict)"("ItemNames"=w73) -> ()  [unwired: 2 in, 2 out]
          }
          event User Event {
            w78 = "Network Synchronization Event" ("format string")
            n38 = event-data() -> ("cycler IP address"=w79:string)  [unwired: 1 in]
            n39 = property on="Event Log" class="MCListbox (strict)"() -> ("ItemNames"=w86:string[][])  [unwired: 2 in, 2 out]
            n40 = Build Array(w80, w79, w78) -> (w84:string[])
            n41 = Format Into String(format string="%s: Cycler: %s - %s", w80, w79, w78) -> (resulting string=w82:string)  [unwired: 2 in, 1 out]
            n42 = local write "Status Message"(w82) -> ()
            n43 = Insert Into Array(array=w86, index (row)=0, new element=w84) -> (w85:string[][])  [unwired: 1 in]
            n44 = property on="Event Log" class="MCListbox (strict)"("ItemNames"=w85) -> ()  [unwired: 2 in, 2 out]
          }
          event User Event {
            n45 = event-data() -> ("cycler IP address"=w96:string, "setpointstatus"=w94:i32, "setpoint_stream_timeout"=w92:u32, "coerced_setpoint_count"=w93:u32)  [unwired: 1 in]
            n46 = case shown="0" w94 {
              tunnel: ["UNKNOWN" ("input 2") "START" ("input 2") "STOP" ("input 2")] -> w91
              frame Default {
              }
              frame 3 {
              }
              frame 0 {
              }
            }
            n47 = Format Into String(format string="Setpoint Status - %d (%s) - Stream Timeout - %d - Coerced Count - %d", w94, w91, w92, w93) -> (resulting string=w95:string)  [unwired: 2 in, 1 out]
            n48 = Build Array(w97, w96, w95) -> (w102:string[])
            n49 = Format Into String(format string="%s: Cycler: %s - %s", w97, w96, w95) -> (resulting string=w99:string)  [unwired: 2 in, 1 out]
            n50 = property on="Event Log" class="MCListbox (strict)"() -> ("ItemNames"=w104:string[][])  [unwired: 2 in, 2 out]
            n51 = local write "Status Message"(w99) -> ()
            n52 = Insert Into Array(array=w104, index (row)=0, new element=w102) -> (w103:string[][])  [unwired: 1 in]
            n53 = property on="Event Log" class="MCListbox (strict)"("ItemNames"=w103) -> ()  [unwired: 2 in, 2 out]
          }
          event User Event {
            n54 = event-data() -> ()  [unwired: 1 in, 1 out]
            n55 = Format Into String(format string="%s:  Self Test Completed", w110) -> (resulting string=w111:string)  [unwired: 2 in, 1 out]
            n56 = local write "Status Message"(w111) -> ()
            n57 = call <vilib>:"Add State(s) to Queue__jki_lib_state_machine.vi"("State(s) in Front (\"\")"="Macro: Self Test Complete", "State(s) in (\"\")"=w115) -> ("States Out"=w114:string)  [unwired: 13 in]
          }
          event "HPS Connect": Value Change {
            n58 = event-data() -> ("NewVal"=w121:bool)  [unwired: 1 in]
            n59 = Select(t="Macro: Connect", s=w121, f="Macro: Disconnect") -> (s? t:f=w118:string)
            n60 = call <vilib>:"Add State(s) to Queue__jki_lib_state_machine.vi"("State(s) in Front (\"\")"=w118, "State(s) in (\"\")"=w123) -> ("States Out"=w122:string)  [unwired: 13 in]
          }
          event "HPS Reserve": Value Change {
            n61 = event-data() -> ("NewVal"=w129:bool)  [unwired: 1 in]
            n62 = Select(t="Macro: Reserve", s=w129, f="Macro: Unreserve") -> (s? t:f=w126:string)
            n63 = call <vilib>:"Add State(s) to Queue__jki_lib_state_machine.vi"("State(s) in Front (\"\")"=w126, "State(s) in (\"\")"=w131) -> ("States Out"=w130:string)  [unwired: 13 in]
          }
          event "HPS Clear": Value Change {
            n64 = event-data() -> ()  [unwired: 1 in, 1 out]
            n65 = call <vilib>:"Add State(s) to Queue__jki_lib_state_machine.vi"("State(s) in Front (\"\")"="HPS: Clear", "State(s) in (\"\")"=w136) -> ("States Out"=w135:string)  [unwired: 13 in]
          }
          event "Apply Mode & Range": Value Change {
            w142 = T6 193 items=["Constant Voltage"=1, "Constant Current"=2, "Internal Recirculation"=193] ("x")
            w144 = T7 2 items=["Low Voltage"=1, "High Voltage"=2] ("y")
            # "Internal Recirculation mode requires Low Voltage\nmode due to the need to recirculate two internal\nbanks of PMSICs.  In High Voltage mode, the two \ninternal banks are placed in series to achieve 1500V"
            n66 = event-data() -> ()  [unwired: 1 in, 1 out]
            n67 = local read "Mode & Range"() -> (w146:cluster{"Mode":T6, "Range":T7})
            n68 = Unbundle By Name(w146) -> ("Mode"=w143:T6, "Range"=w145:T7)
            n69 = Equal?(x=w142, y=w143) -> (x = y?=w141:bool)
            n70 = Equal?(x=w145, y=w144) -> (x = y?=w140:bool)
            n71 = And(x=w141, y=w140) -> (x .and. y?=w139:bool)
            n72 = case shown="True" w139 {
              tunnel: ["HPS: Set Mode and Range" _] -> w149
              tunnel: w148 -> [w153 w158]
              tunnel: [w153 w157] -> w147
              frame False {
              }
              frame True {
                n73 = call "Dialog Launcher.vi"("error in (no error)"=w158, "Message"="Internal Recirculation mode can only be set when the range is also set to Low Voltage.", "Title"="Invalid Mode & Range Configuration") -> ("error out"=w157:errorcluster)  [unwired: 8 in]
              }
            }
            n74 = call <vilib>:"Add State(s) to Queue__jki_lib_state_machine.vi"("State(s) in Front (\"\")"=w149, "State(s) in (\"\")"=w151) -> ("States Out"=w150:string)  [unwired: 13 in]
          }
          event "Apply Limits": Value Change {
            n75 = event-data() -> ()  [unwired: 1 in, 6 out]
            n76 = call <vilib>:"Add State(s) to Queue__jki_lib_state_machine.vi"("State(s) in Front (\"\")"="HPS: Set Limits" ("State(s) in Front (\"\")"), "State(s) in (\"\")"=w161) -> ("States Out"=w160:string)  [unwired: 13 in]
          }
          event "Energize": Value Change {
            n77 = event-data() -> ()  [unwired: 1 in, 6 out]
            n78 = call <vilib>:"Add State(s) to Queue__jki_lib_state_machine.vi"("State(s) in Front (\"\")"="HPS: Energize" ("State(s) in Front (\"\")"), "State(s) in (\"\")"=w166) -> ("States Out"=w165:string)  [unwired: 13 in]
          }
          event "Output": Value Change {
            n79 = event-data() -> ()  [unwired: 1 in, 6 out]
            n80 = call <vilib>:"Add State(s) to Queue__jki_lib_state_machine.vi"("State(s) in Front (\"\")"="HPS: Output" ("State(s) in Front (\"\")"), "State(s) in (\"\")"=w171) -> ("States Out"=w170:string)  [unwired: 13 in]
          }
          event "Apply Setpoints": Value Change {
            n81 = event-data() -> ()  [unwired: 1 in, 6 out]
            n82 = call <vilib>:"Add State(s) to Queue__jki_lib_state_machine.vi"("State(s) in Front (\"\")"="HPS: Apply Setpoints" ("State(s) in Front (\"\")"), "State(s) in (\"\")"=w176) -> ("States Out"=w174:string)  [unwired: 13 in]
          }
          event "Acknowledge Faults": Value Change {
            n83 = event-data() -> ()  [unwired: 1 in, 1 out]
            n84 = Unbundle By Name(w181) -> ("HPS17K Refs"=w180:refnum<class "HPS-17000.lvclass">[], "Reserved"=w179:bool)
            n85 = case shown="False" w179 {
              tunnel: w183 -> [w186 w192]
              tunnel: [w185 w189] -> w182
              tunnel: w180 -> [_ w191]
              frame False {
                n86 = call "Dialog Launcher.vi"("error in (no error)"=w186, "Message"="You must first connect to and then reserve the \nHPS17K before you can acknowledge faults.", "Title"="HPS17K Not Reserved") -> ("error out"=w185:errorcluster)  [unwired: 8 in]
              }
              frame True {
                n87 = call-poly <instrlib>:"Acknowledge Faults.vi"("error in"=w192, "cycler refs in"=w191) -> ("error out"=w190:errorcluster)  [unwired: 8 in, 1 out]
                n88 = case shown="Error .." w190 {
                  selector: w190 -> [w194 w195]
                  tunnel: [w194 w195] -> w189
                  frame No Error {
                    n89 = local write "Fault Message"("" ("Fault Message")) -> ()
                  }
                  frame Error {
                  }
                }
              }
            }
          }
          event "Clear Event Log": Value Change {
            n90 = event-data() -> ()  [unwired: 1 in, 1 out]
            n91 = property on="Event Log" class="MCListbox (strict)"("ItemNames"=string[][] [] ("Item Names")) -> ()  [unwired: 2 in, 2 out]
          }
          event "Start Profile": Value Change {
            n92 = event-data() -> ()  [unwired: 1 in, 1 out]
            n93 = Select(t="Macro: Start Setpoint Stream" ("State(s) in Front (\"\")"), s="Start Profile", f="Macro: Stop Setpoint Stream" ("State(s) in Front (\"\")")) -> (s? t:f=w200:string)
            n94 = call <vilib>:"Add State(s) to Queue__jki_lib_state_machine.vi"("State(s) in Front (\"\")"=w200, "State(s) in (\"\")"=w205) -> ("States Out"=w204:string)  [unwired: 13 in]
          }
          event "Volta Monitor": Value Change {
            n95 = event-data() -> ()  [unwired: 1 in, 6 out]
            n96 = call <vilib>:"Add State(s) to Queue__jki_lib_state_machine.vi"("State(s) in Front (\"\")"="Script: Volta Monitor" ("State(s) in Front (\"\")"), "State(s) in (\"\")"=w209) -> ("States Out"=w208:string)  [unwired: 13 in]
          }
          event "FC Sys Inspect": Value Change {
            n97 = event-data() -> ()  [unwired: 1 in, 6 out]
            n98 = call <vilib>:"Add State(s) to Queue__jki_lib_state_machine.vi"("State(s) in Front (\"\")"="Script: FC Sys Inspect" ("State(s) in Front (\"\")"), "State(s) in (\"\")"=w214) -> ("States Out"=w213:string)  [unwired: 13 in]
          }
          event "Get XC Report": Value Change {
            n99 = event-data() -> ()  [unwired: 1 in, 6 out]
            n100 = call <vilib>:"Add State(s) to Queue__jki_lib_state_machine.vi"("State(s) in Front (\"\")"="HPS: Get Diagnostic Data", "State(s) in (\"\")"=w219) -> ("States Out"=w218:string)  [unwired: 13 in]
          }
          event "Launch Test Server": Value Change {
            n101 = event-data() -> ("NewVal"=w226:bool)  [unwired: 1 in]
            n102 = Select(t="Macro: Start Test Server" ("State(s) in Front (\"\")"), s=w226, f="Macro: Stop Test Server" ("State(s) in Front (\"\")")) -> (s? t:f=w229:string)
            n103 = Select(t="%s: Start Test Server" ("format string"), s=w226, f="%s: Stop Test Server" ("format string")) -> (s? t:f=w224:string)
            n104 = Format Into String(format string=w224, w227) -> (resulting string=w228:string)  [unwired: 2 in, 1 out]
            n105 = call <vilib>:"Add State(s) to Queue__jki_lib_state_machine.vi"("State(s) in Front (\"\")"=w229, "State(s) in (\"\")"=w233) -> ("States Out"=w232:string)  [unwired: 13 in]
            n106 = local write "Status Message"(w228) -> ()
          }
          event "Run Self Test": Value Change {
            n107 = event-data() -> ("NewVal"=w236:bool)  [unwired: 1 in]
            n108 = Select(t="%s: Self Test Started" ("format string"), s=w236, f="%s: Self Test Stopped" ("format string")) -> (s? t:f=w238:string)
            n109 = Select(t="Macro: Start Self Test" ("State(s) in Front (\"\")"), s=w236, f="Macro: Stop Self Test" ("State(s) in Front (\"\")")) -> (s? t:f=w242:string)
            n110 = Format Into String(format string=w238, w237) -> (resulting string=w241:string)  [unwired: 2 in, 1 out]
            n111 = local write "Status Message"(w241) -> ()
            n112 = call <vilib>:"Add State(s) to Queue__jki_lib_state_machine.vi"("State(s) in Front (\"\")"=w242, "State(s) in (\"\")"=w246) -> ("States Out"=w245:string)  [unwired: 13 in]
          }
          event "Use Local Time": Value Change {
            n113 = event-data() -> ("NewVal"=w250:bool)  [unwired: 1 in]
            n114 = Unbundle By Name(w253) -> ("Grapher Ref"=w252:refnum<class "Grapher.lvclass">)
            n115 = call "Set Time Selector.vi"("reference in"=w252, "Use Local Time?"=w250, "Error In"=w251) -> ("Error Out"=w249:errorcluster)  [unwired: 15 in, 1 out]
          }
          event "High Speed": Value Change {
            n116 = event-data() -> ("NewVal"=w255:bool)  [unwired: 1 in]
            n117 = Unbundle By Name(w259) -> ("Grapher Ref"=w256:refnum<class "Grapher.lvclass">)
            n118 = call "Set High Speed.vi"("reference in"=w256, "High Speed?"=w255, "Error In"=w258) -> ("Error Out"=w257:errorcluster)  [unwired: 15 in, 1 out]
          }
          event "Graph Samples": Value Change {
            n119 = event-data() -> ("NewVal"=w262:u32)  [unwired: 1 in]
            n120 = Unbundle By Name(w265) -> ("Grapher Ref"=w263:refnum<class "Grapher.lvclass">)
            n121 = call "Set Graph Samples.vi"("reference in"=w263, "Graph Samples"=w262, "Error In"=w264) -> ("Error Out"=w261:errorcluster)  [unwired: 15 in, 1 out]
          }
          event "Graph Data Decimation": Value Change {
            n122 = event-data() -> ("NewVal"=w267:i32)  [unwired: 1 in]
            n123 = Unbundle By Name(w271) -> ("Grapher Ref"=w268:refnum<class "Grapher.lvclass">)
            n124 = call "Set Graph Decimation.vi"("reference in"=w268, "Graph Decimation"=w267, "Error In"=w270) -> ("Error Out"=w269:errorcluster)  [unwired: 15 in, 1 out]
          }
          event "Get Device Properties": Value Change {
            n125 = event-data() -> ()  [unwired: 1 in, 6 out]
            n126 = Unbundle By Name(w275) -> ("HPS17K Refs"=w274:refnum<class "HPS-17000.lvclass">[], "Connected"=w273:bool)
            n127 = case shown="True" w273 {
              tunnel: w277 -> [w279 w289]
              tunnel: [w279 w288] -> w276
              tunnel: w274 -> [_ w287]
              frame False {
              }
              frame True {
                n128 = local read "Cycler Selection"() -> (w282:i16)
                n129 = call-poly <instrlib>:"Identify.vi"("error in"=w289, "blink"=TRUE, "cycler refs in"=w287) -> ("error out"=w288:errorcluster, "device properties"=w285:T9[])  [unwired: 6 in, 1 out]
                n130 = In Range and Coerce(upper limit=i16 50 ("lower limit"), x=w282, lower limit=i16 0) -> (coerced(x)=w281:i16)  [unwired: 1 out]
                n131 = Index Array(array=w285, index=w281) -> (element=→"device properties":T9)
              }
            }
          }
          event "HPS17K Search": Value Change {
            n132 = event-data() -> ()  [unwired: 1 in, 6 out]
            n133 = call <instrlib>:"Find All HPS-17000s.vi"("error in"=w296, "controller TSN IP"="Controller TSN IP") -> ("error out"=w293:errorcluster, "HPS-17000 IPs"=w294:string[], "HPS-17000 names"=w292:string[])  [unwired: 7 in]
            n134 = invoke on="Device Search" class="Tree (strict)" method="Edit Tree Items.Delete"(error in=w293) -> (error out=w295:errorcluster)  [unwired: 4 in, 4 out]
            n135 = Build Array(w292) -> (w291:string[][])
            n136 = for {
              shift-right: [w302] -> w290
              shift-left: w295 -> [w303]
              tunnel: w294 -> [w301] mode=indexing
              tunnel: w291 -> [w300] mode=indexing
              n137 = invoke on="Device Search" class="Tree (strict)" method="Edit Tree Items.Add Item"(error in=w303, "Left Cell"=w301, "Child Text"=w300, "Child Tag"=w301) -> (error out=w302:errorcluster)  [unwired: 5 in, 8 out]
            }
          }
          event "CSV Profile": Value Change {
            n138 = event-data() -> ()  [unwired: 1 in, 1 out]
            n139 = call <vilib>:"Add State(s) to Queue__jki_lib_state_machine.vi"("State(s) in Front (\"\")"="Profile: Load" ("State(s) in Front (\"\")"), "State(s) in (\"\")"=w306) -> ("States Out"=w304:string)  [unwired: 13 in]
          }
          event "Apply Slew Rates": Value Change {
            n140 = event-data() -> ()  [unwired: 1 in, 1 out]
            n141 = call <vilib>:"Add State(s) to Queue__jki_lib_state_machine.vi"("State(s) in Front (\"\")"="Macro: Update Slew Rate", "State(s) in (\"\")"=w310) -> ("States Out"=w309:string)  [unwired: 13 in]
          }
          event "Generate EIS Profile": Value Change {
            n142 = event-data() -> ()  [unwired: 1 in, 6 out]
            n143 = call <vilib>:"Add State(s) to Queue__jki_lib_state_machine.vi"("State(s) in Front (\"\")"="EIS: Create Profile", "State(s) in (\"\")"=w315) -> ("States Out"=w314:string)  [unwired: 13 in]
          }
          event "Generate EIS Report": Value Change {
            n144 = event-data() -> ()  [unwired: 1 in, 6 out]
            n145 = call <vilib>:"Add State(s) to Queue__jki_lib_state_machine.vi"("State(s) in Front (\"\")"="EIS: Generate Report", "State(s) in (\"\")"=w320) -> ("States Out"=w319:string)  [unwired: 13 in]
          }
          event "EIS Save & Load Profile": Value Change {
            n146 = event-data() -> ()  [unwired: 1 in, 6 out]
            n147 = call <vilib>:"Add State(s) to Queue__jki_lib_state_machine.vi"("State(s) in Front (\"\")"="EIS: Save Profile", "State(s) in (\"\")"=w325) -> ("States Out"=w324:string)  [unwired: 13 in]
          }
          event "Update Temperatures": Value Change {
            n148 = event-data() -> ()  [unwired: 1 in, 1 out]
            n149 = call <vilib>:"Add State(s) to Queue__jki_lib_state_machine.vi"("State(s) in Front (\"\")"="Script: Read Temperatures", "State(s) in (\"\")"=w329) -> ("States Out"=w331:string)  [unwired: 13 in]
          }
          event "Start Logging": Value Change {
            n150 = event-data() -> ("NewVal"=w337:bool)  [unwired: 1 in]
            n151 = Select(t="Script: Launch Logger", s=w337, f="Script: Stop Logger") -> (s? t:f=w334:string)
            n152 = call <vilib>:"Add State(s) to Queue__jki_lib_state_machine.vi"("State(s) in Front (\"\")"=w334, "State(s) in (\"\")"=w338) -> ("States Out"=w339:string)  [unwired: 13 in]
          }
          event "Save Chart": Value Change {
            n153 = event-data() -> ()  [unwired: 1 in, 1 out]
            n154 = Unbundle By Name(w343) -> ("Grapher Ref"=w342:refnum<class "Grapher.lvclass">)
            n155 = call "Save Chart.vi"("reference in"=w342, "Error In"=w345) -> ("Error Out"=w344:errorcluster)  [unwired: 16 in, 1 out]
          }
          event "Log File Directory": Value Change {
            n156 = event-data() -> ("NewVal"=w351:path)  [unwired: 1 in]
            n157 = Empty String/Path?(string/path=w351) -> (empty?=w350:bool)
            n158 = Select(t=T14."Disabled and Grayed Out" ("Disabled"), s=w350, f=T14."Enabled" ("Disabled")) -> (s? t:f=w347:T14)
            n159 = property on="Start Logging" class="Bool (strict)"("DisabledEnum"=w347) -> ()  [unwired: 2 in, 2 out]
          }
          event "Add HPS17K": Value Change {
            n160 = event-data() -> ()  [unwired: 1 in, 6 out]
            n161 = call <vilib>:"Add State(s) to Queue__jki_lib_state_machine.vi"("State(s) in Front (\"\")"="UI: Add HPS17K", "State(s) in (\"\")"=w357) -> ("States Out"=w355:string)  [unwired: 13 in]
          }
          event "Remove HPS17K": Value Change {
            n162 = event-data() -> ()  [unwired: 1 in, 6 out]
            n163 = call <vilib>:"Add State(s) to Queue__jki_lib_state_machine.vi"("State(s) in Front (\"\")"="UI: Remove HPS17K", "State(s) in (\"\")"=w362) -> ("States Out"=w360:string)  [unwired: 13 in]
          }
          event "Erase Chart": Value Change {
            n164 = event-data() -> ()  [unwired: 1 in, 1 out]
            n165 = Unbundle By Name(w366) -> ("Grapher Ref"=w365:refnum<class "Grapher.lvclass">)
            n166 = call "Erase Chart.vi"("reference in"=w365, "Error In"=w368) -> ("Error Out"=w367:errorcluster)  [unwired: 16 in, 1 out]
          }
          event "Pause Chart": Value Change {
            n167 = event-data() -> ("NewVal"=w373:bool)  [unwired: 1 in]
            n168 = Unbundle By Name(w371) -> ("Grapher Ref"=w370:refnum<class "Grapher.lvclass">)
            n169 = call "Set Pause.vi"("reference in"=w370, "Set Pause"=w373, "Error In"=w374) -> ("Error Out"=w372:errorcluster)  [unwired: 15 in, 1 out]
          }
          event "TDMS Viewer": Value Change {
            n170 = event-data() -> ()  [unwired: 1 in, 1 out]
            n171 = call "File Dialog3"("error in"=w380) -> ("selected path"=w379:path, "cancelled"=w377:bool, "error out"=w376:errorcluster)  [unwired: 11 in, 1 out]
            n172 = case shown="No Error" w376 {
              selector: w376 -> [w383 _]
              tunnel: w379 -> [w386 _]
              tunnel: [w385 errorcluster {"status"=FALSE, "code"=0, "source"=""} ("error IO")] -> w378
              tunnel: w377 -> [w384 _]
              frame No Error {
                n173 = case shown="False" w384 {
                  tunnel: w383 -> [w396 w397]
                  tunnel: w386 -> [w389 _]
                  tunnel: [w387 w397] -> w385
                  frame False {
                    w391 = 128  # call & forget
                    n174 = vi-ref "NI_TDMS File Viewer.lvlib:TDMS - File Viewer (NXG Style).vi"() -> (w395:refnum<vi>)
                    n175 = property class="VI Interface Type 0"(reference=w395, error in=w396) -> (reference out=w393:refnum<vi>, error out=w394:errorcluster, "Path"=w392:path)
                    n176 = Open VI Reference(type specifier VI Refnum (for type only)=w393, vi path=w392, options=w391, error in (no error)=w394) -> (vi reference=w390:refnum<vi>, error out=w388:errorcluster)  [unwired: 2 in]
                    n177 = call-by-ref "Start Asynchronous Call"(reference=w390, error in=w388, "error in"=w388, "file in"=w389) -> (error out=w387:errorcluster)  [unwired: 8 in, 3 out]
                  }
                  frame True {
                  }
                }
              }
              frame Error {
              }
            }
          }
          event "HPS17K IP Addresses": Shortcut Menu Selection (User) {
            n178 = event-data() -> ("ItemTag"=w403:string)  [unwired: 1 in]
            n179 = case shown="Default" w403 {
              tunnel: w402 -> [w406 w408 w412]
              tunnel: [w406 w407 w411] -> w401
              tunnel: w400 -> [w405 w410 w414]
              tunnel: [w405 w410 w414] -> w399
              frame Default {
              }
              frame "Add HPS17K" {
                n180 = call <vilib>:"Add State(s) to Queue__jki_lib_state_machine.vi"("State(s) in Front (\"\")"="UI: Add HPS17K", "State(s) in (\"\")"=w408) -> ("States Out"=w407:string)  [unwired: 13 in]
              }
              frame "Remove HPS17K" {
                n181 = call <vilib>:"Add State(s) to Queue__jki_lib_state_machine.vi"("State(s) in Front (\"\")"="UI: Remove HPS17K", "State(s) in (\"\")"=w412) -> ("States Out"=w411:string)  [unwired: 13 in]
              }
            }
          }
          event "Device Search": Drag Starting? {
            n182 = event-data() -> ("Data"=w415:T15)  [unwired: 1 in]
            n183 = Bundle By Name(cluster=w417, "Drag Data"=w415) -> (w416:T13)
            n184 = event-data("Discard?"=FALSE) -> ()  [unwired: 3 in, 1 out]
          }
          event "HPS17K IP Addresses": Drop {
            n185 = event-data() -> ("Available Data Names"=w436:string[], "CtlRef"=w440:refnum<vi>)  [unwired: 1 in]
            n186 = Unbundle By Name(w437) -> ("Drag Data"=w434:T15)
            n187 = Search 1D Array(1D array=w436, element="LV_TREE_TAG") -> (index of element=w433:i32)  [unwired: 1 in]
            n188 = property class="Tree (strict)"(reference=w440, error in=w430) -> (error out=w429:errorcluster, "All Tags"=w427:string[])  [unwired: 1 out]
            n189 = Index Array(array=w434, index=w433) -> (element=w432:cluster{"data name":string, "drag data":variant})
            n190 = Unbundle By Name(w432) -> ("drag data"=w431:variant)
            n191 = Variant To Data(error in=w429, type="" ("element"), Variant=w431) -> (data=w422:string, error out=w423:errorcluster)
            n192 = Search 1D Array(1D array=w427, element=w422) -> (index of element=w426:i32)  [unwired: 1 in]
            n193 = Less Than 0?(x=w426) -> (x < 0?=w424:bool)
            n194 = case shown="True" w424 {
              tunnel: w423 -> [w442 w452]
              tunnel: w422 -> [_ w444]
              tunnel: [w442 w451] -> w421
              frame False {
              }
              frame True {
                n195 = property on="Cycler Selection" class="Ring (strict)"() -> ("StringsAndValues[]"=w448:T21)  [unwired: 2 in, 2 out]
                n196 = Array Size(array=w448) -> (size(s)=w449:i32)
                n197 = Decrement(x=w449) -> (x-1=w450:i32)
                n198 = invoke on="HPS17K IP Addresses" class="Tree (strict)" method="Edit Tree Items.Add Item"(error in=w452, "Left Cell"=w444, "Child Tag"=w444) -> (error out=w451:errorcluster)  [unwired: 6 in, 8 out]
                n199 = Bundle By Name(cluster=cluster{"String":string, "Value":i16} {"String"="", "Value"=0} ("new element/subarray"), "String"=w444, "Value"=w450) -> (w447:cluster{"String":string, "Value":i16})
                n200 = property on="HPS Connect" class="Bool (strict)"("DisabledEnum"=T14."Enabled" ("Disabled")) -> ()  [unwired: 2 in, 2 out]
                n201 = Insert Into Array(array=w448, new element=w447) -> (w446:T21)  [unwired: 1 in]
                n202 = property on="Cycler Selection" class="Ring (strict)"("StringsAndValues[]"=w446) -> ()  [unwired: 2 in, 2 out]
              }
            }
            n203 = Bundle By Name(cluster=w437, "Drag Data"=T15 []) -> (w439:T13)
            n204 = event-data("Accepted?"=FALSE) -> ()  [unwired: 1 in, 1 out]
          }
          event Panel Close? {
            # "Close Panel button (pressed) Event\n(this executes Macro: Exit to terminate the VI)"
            n205 = event-data() -> ()  [unwired: 1 in, 1 out]
            n206 = Unbundle By Name(w455) -> ("Connected"=w454:bool)
            n207 = case shown="True" w454 {
              tunnel: [TRUE ("T button?") w463] -> w457
              frame False {
              }
              frame True {
                n208 = Two Button Dialog(message="Are you sure you want to close HPS17K Panel?  Your control to the unit will be relinquished which could impact connected devices.", 1:"No" ("F button name (\"Cancel\")"), 2:"Yes" ("T button name (\"OK\")")) -> (T button?=w463:bool)
              }
            }
            n209 = call <vilib>:"Conditional State String__jki_lib_state_machine.vi"("Do State(s)?"=w457, "State"="Macro: Exit") -> ("State Out"=w456:string)  [unwired: 7 in]
            n210 = call <vilib>:"Add State(s) to Queue__jki_lib_state_machine.vi"("State(s) in Front (\"\")"=w456, "State(s) in (\"\")"=w461) -> ("States Out"=w460:string)  [unwired: 13 in]
            n211 = event-data("Discard?"=TRUE) -> ()  [unwired: 1 in, 1 out]
          }
        }
      }
      frame "---------- Core ----------" {
        # "Do not put any code in this frame.\n(it is a separator no-op)"
        n212 = call <vilib>:"Add State(s) to Queue__jki_lib_state_machine.vi"("State(s) in (\"\")"=w471) -> ("States Out"=w470:string)  [unwired: 14 in]
      }
      frame Default {
        w482 = 42 items=["No error", "Argument error", "Memory is full", "Out of zone", "End of file", "File already open", "Generic file I/O error", "File not found", "File permission error", "Disk is full", "Duplicate path", "Too many files open", "System feature not enabled", "Resource file not found", "Cannot add resource", "Resource not found", "Image not found", "Image memory error", "Pen does not exist", "Config type invalid", "Config token not found", "Config parse error", "Config memory error", "Bad external code format", "Bad external code offset", "External code not present", "Null window", "Destroy window error", "Null menu", "Print aborted", "Bad print record", "Print driver error", "Windows error during printing", "Memory error during printing", "Print dialog error", "Generic print error", "Invalid device refnum", "Device not found", "Device parameter error", "Device unit error", "Cannot open device", "Device call aborted", "Generic error", "Cancelled by user", "Object ID too low", "Object ID too high", "Object not in heap", "Unknown heap", "Unknown object (invalid DefProc)", "Unknown object (DefProc not in table)", "Message out of range", "Invalid (null) method", "Unknown message", "Manager call not supported", "Bad address", "Network operation in progress", "Network operation timed out", "Connection is busy", "Network attribute not supported", "Network error", "Address in use", "System out of memory", "Connection aborted", "Connection refused", "Not connected", "Already connected", "Connection closed", "Initialization error (interapplication manager)", "Bad occurrence", "Wait on unbound occurrence handler", "Occurrence queue overflow", "Datalog type conflict", "Unused", "Unrecognized type (interapplication manager)", "Memory corrupt", "Failed to make temporary DLL", "Old CIN version", "Drag socket not found", "Failed to load drop-object", "Failed to register OLE object", "Failed to release OLE object", "Format specifier type mismatch", "Unknown format specifier", "Too few format specifiers", "Too many format specifiers", "Scan failed", "Newer CIN version", "Error converting to variant", "Runtime menu error", "Password tampered", "Variant attribute not found", "Incompatible variant data type", "Event data is not available", "Event Store is not present", "Occurrence is not found", "Event Queue is not created", "Event info is not available", "Refnum passed is NULL", "Error retrieving Class GUID", "Error retrieving CoClass GUID", "Error retrieving TypeLib GUID.", "Bad built application magic bytes.", "Specific driver is different from the specific driver associated with the Logical Name.", "There is no session opened to the class driver.", "Max Error", "MAX - Error with config objects", "MAX - Error loading configuration", "MAX - Group not supported"]
        # "Current State"
        # "Do not delete, rename, or modify this frame.\n(this is used to capture unhandled states and typos)"
        # "Handle mistyped state name (developer tool)"
        n213 = Format Into String(format string="Software Exception: Unhandled State \"%s\"." ("message"), error in=w478, w473) -> (resulting string=w481:string, error out=w480:errorcluster)  [unwired: 1 in]
        n214 = call <vilib>:"Error Cluster From Error Code.vi"("show call chain? (False)"=TRUE, "error in (no error)"=w480, "error message (\"\")"=w481, "error code (0)"=w482) -> ("error out"=w479:errorcluster)  [unwired: 5 in]
        n215 = call <vilib>:"Add State(s) to Queue__jki_lib_state_machine.vi"("State(s) in (\"\")"=w477) -> ("States Out"=w476:string)  [unwired: 14 in]
      }
      frame "Initialize Core Data" {
        # "Do not delete, rename, or modify this frame.\n(this is used to determine panel behavior on exit)"
        # "originally closed?"
        # "exe?"
        # "If panel starts closed or is an EXE, then close it when we exit"
        n216 = property class="VI"() -> ("FP.State"=w491:T16)  [unwired: 2 in, 2 out]
        n217 = property class="App"() -> ("App.Kind"=w497:T17)  [unwired: 2 in, 2 out]
        n218 = control-ref of="Current VI Reference"() -> (w492:refnum<vi>)
        n219 = Equal?(x=w491, y=T16."Closed" ("Front Panel Window:State")) -> (x = y?=w489:bool)
        n220 = Equal?(x=w497, y=T17."Run Time System" ("Application:Kind")) -> (x = y?=w495:bool)
        n221 = call <resource>:"LV Config Write Boolean.vi"("error in (no error)"=w485, "value"=TRUE, "key"="allowmultipleinstances") -> ("error out"=w484:errorcluster)  [unwired: 4 in]
        n222 = Or(x=w489, y=w495) -> (x .or. y?=w493:bool)
        n223 = call <vilib>:"Add State(s) to Queue__jki_lib_state_machine.vi"("State(s) in (\"\")"=w500) -> ("States Out"=w499:string)  [unwired: 14 in]
        n224 = Bundle By Name(cluster=w494, "Core.Current VI Reference"=w492, "Core.Close Panel on Exit?"=w493) -> (w498:T13)
      }
      frame "Error Handler" {
        # "When running as sourcecode, this function will add previous state data to the error message to aid the developer in troubleshoot errors.\nIf run as an executable, no additional information is added to the error message."
        # "This state receives both Errors and Warnings which is how the Status of this wire can be FALSE"
        # "Unhandled Error -- Display it"
        # "Handle any errors or warnings here.\nYou can also output any states to clean-up after errors or warnings occur"
        # "Clear error or warning"
        n225 = disable-structure shown="Default" {
          disable-tunnel: w507 -> [w514 w515]
          disable-tunnel: w506 -> [w513 _]
          disable-tunnel: [w512 w515] -> w505
          frame condition #0 (active) {
            n226 = call <vilib>:"Append Error Details__jki_lib_state_machine.vi"("error in (no error)"=w514, "Previous State and Argument(s)"=w513) -> ("error out"=w512:errorcluster)  [unwired: 9 in]
          }
          frame condition #1 {
          }
        }
        n227 = call <vilib>:"General Error Handler.vi"("error in (no error)"=w505) -> ()  [unwired: 10 in, 5 out]
        n228 = call-poly <vilib>:"Select State(s)__jki_lib_state_machine.vi"("State(s) if True (\"\")"="/* Post Error States", "Select"=w505, "State(s) if False (\"\")"="/* Post Warning States") -> ("States Out"=w503:string)  [unwired: 12 in]
        n229 = call <vilib>:"Add State(s) to Queue__jki_lib_state_machine.vi"("State(s) in Front (\"\")"=w503, "State(s) in (\"\")"=w511) -> ("States Out"=w510:string)  [unwired: 13 in]
      }
      frame "Exit" {
        # "Do not put any code in this frame.\n(No errors that occur here will be handled.)"
        n230 = call <vilib>:"Add State(s) to Queue__jki_lib_state_machine.vi"("State(s) in (\"\")"=w521) -> ("States Out"=w520:string)  [unwired: 14 in]
      }
      frame "---------- Data ----------" {
        # "Do not put any code in this frame.\n(It is a separator no-op. You can make a copy of this frame to create a new Data frame)"
        n231 = call <vilib>:"Add State(s) to Queue__jki_lib_state_machine.vi"("State(s) in (\"\")"=w526) -> ("States Out"=w525:string)  [unwired: 14 in]
      }
      frame "Data: Cleanup" {
        # "Cleanup any data and references, here.\n(this is called automatically, by the Macro: Exit)"
        n232 = Unbundle By Name(w540) -> ("Self Test Completed"=w529:refnum<user-event>, "Logger Queue"=w536:refnum<queue>, "Graph Queue"=w537:refnum<queue>, "Core.Current VI Reference"=w541:refnum<vi>)
        n233 = Release Queue(queue=w536) -> (error out=w533:errorcluster)  [unwired: 2 in, 2 out]
        n234 = Release Queue(queue=w537) -> (error out=w532:errorcluster)  [unwired: 2 in, 2 out]
        n235 = Close Reference(reference=w541, error in (no error)=w538) -> (error out=w535:errorcluster)
        n236 = Destroy User Event(user event=w529) -> (error out=w528:errorcluster)  [unwired: 1 in]
        n237 = call <vilib>:"Clear Errors.vi"("error in (no error)"=w528) -> ("error out"=w527:errorcluster)  [unwired: 5 in, 1 out]
        n238 = call <vilib>:"Clear Errors.vi"("error in (no error)"=w533) -> ("error out"=w530:errorcluster)  [unwired: 5 in, 1 out]
        n239 = call <vilib>:"Clear Errors.vi"("error in (no error)"=w532) -> ("error out"=w531:errorcluster)  [unwired: 5 in, 1 out]
        n240 = Merge Errors(w527, w530, w531, w535) -> (w534:errorcluster)
        n241 = call <vilib>:"Add State(s) to Queue__jki_lib_state_machine.vi"("State(s) in (\"\")"=w543) -> ("States Out"=w542:string)  [unwired: 14 in]
      }
      frame "Data: Initialize" {
        w552 = T23[][] []
        w555 = T24 {"Current VI Reference"=refnum, "Close Panel on Exit?"=FALSE}  # Core
        n242 = Obtain Queue(max queue size (-1, unlimited)=1000, element data type=w552, error in (no error)=w549) -> (queue out=w546:refnum<queue>, error out=w547:errorcluster)  [unwired: 2 in, 1 out]
        n243 = Obtain Queue(max queue size (-1, unlimited)=1000, element data type=w552, error in (no error)=w549) -> (queue out=w545:refnum<queue>, error out=w548:errorcluster)  [unwired: 2 in, 1 out]
        n244 = Merge Errors(w547, w548) -> (w544:errorcluster)
        n245 = Bundle By Name(cluster=w556, "Core"=w555, "Graph Queue"=w546, "Logger Queue"=w545) -> (w554:T13)
        n246 = call <vilib>:"Add State(s) to Queue__jki_lib_state_machine.vi"("State(s) in (\"\")"=w558) -> ("States Out"=w557:string)  [unwired: 14 in]
      }
      frame "Data: Update Periodic" {
        n247 = local read "Cycler Selection"() -> (w563:i16)
        n248 = Unbundle By Name(w570) -> ("HPS17K Refs"=w566:refnum<class "HPS-17000.lvclass">[], "Connected"=w571:bool)
        n249 = Empty Array?(array=w566) -> (empty?=w565:bool)
        n250 = To Long Integer(number=w563) -> (32bit integer=w562:i32)
        n251 = Not(x=w565) -> (.not. x?=w564:bool)
        n252 = And(x=w571, y=w564) -> (x .and. y?=w569:bool)
        n253 = In Range and Coerce(upper limit=50, x=w562, lower limit=0) -> (coerced(x)=w560:i32)  [unwired: 1 out]
        n254 = case shown="True" w569 {
          tunnel: w568 -> [w574 w598]
          tunnel: w566 -> [_ w604]
          tunnel: [w574 w602] -> w567
          tunnel: w560 -> [_ w580]
          frame False {
          }
          frame True {
            w577 = T22 1 items=["ERROR_GLOB_EMO_GLOBAL"=0, "ERROR_GLOB_EMO_BUTTON_PRESSED"=1, "ERROR_GLOB_USER"=2, "ERROR_GLOB_PM"=3, "ERROR_GLOB_GRID"=4, "ERROR_GLOB_VOLTAGE_DCBUS_OUT_OF_BOUNDS"=6, "ERROR_GLOB_VOLTAGE_OUTPUT_HIGH"=7, "ERROR_GLOB_VOLTAGE_OUTPUT_LOW"=8, "ERROR_GLOB_VOLTAGE_OUTPUT_UNBALANCE"=9, "ERROR_GLOB_CURRENT_OUTPUT_HIGH"=10, "ERROR_GLOB_SYS_OVERTEMPERATURE"=13, "ERROR_GLOB_SYS_HW"=14, "ERROR_GLOB_SYS_COMM"=15, "ERROR_GLOB_SYNC_AND_CONNECT"=16, "ERROR_GLOB_SP"=20, "ERROR_GLOB_SP_TRACKING"=21, "ERROR_GLOB_CONFIG"=23, "ERROR_GLOB_REG_SYS"=27, "ERROR_GLOB_REG_GRID"=28, "ERROR_GLOB_REG_AFE1"=29, "ERROR_GLOB_REG_AFE2"=30, "ERROR_GLOB_REG_DC"=31] ("element")
            n255 = call-poly <instrlib>:"Get Status.vi"("error in"=w598, "cycler refs in"=w604) -> ("error out"=w596:errorcluster, "heartbeat valid"=w594:bool[], "ok"=→"OK":bool)  [unwired: 6 in, 1 out]
            n256 = call-poly <instrlib>:"Get Faults.vi"("error in"=w598, "cycler refs in"=w604) -> ("error out"=w599:errorcluster, "faults"=w581:u64[])  [unwired: 7 in, 1 out]
            n257 = call-poly <instrlib>:"Get Mode.vi"("error in"=w598, "cycler refs in"=w604) -> ("error out"=w600:errorcluster, "range"=w592:T25[], "mode"=w590:T26[])  [unwired: 6 in, 1 out]
            n258 = call-poly <instrlib>:"Get Limits.vi"("error in"=w598, "cycler refs in"=w604) -> ("error out"=w601:errorcluster, "limits out"=w615:T8)  [unwired: 7 in, 1 out]
            n259 = call-poly <instrlib>:"Get Enabled Output.vi"("error in"=w598, "cycler refs in"=w604) -> ("error out"=w603:errorcluster, "enabled output"=w588:bool[])  [unwired: 7 in, 1 out]
            n260 = Index Array(array=w594, index=w580) -> (element=→"Heartbeat Valid":bool)
            n261 = Index Array(array=w590, index=w580) -> (element=→"MODE":T26)
            n262 = Index Array(array=w592, index=w580) -> (element=w591:T25)
            n263 = Index Array(array=w588, index=w580) -> (element=w587:bool)
            "Output Enabled" <- w587
            n264 = Unbundle By Name(w615) -> ("Current Max Limit"=→"Current Maximum":sgl, "Current Min Limit"=→"Current Minimum":sgl, "Voltage Max Limit"=→"Voltage Maximum":sgl, "Voltage Min Limit"=→"Voltage Minimum":sgl, "Power Max Limit"=w610:sgl, "Power Min Limit"=w608:sgl)
            n265 = case shown="1, Default" w591 {
              frame 1, Default {
                w617 = 480.0 ("Scale.Range:Maximum")
                (unwired) T25 1 items=["low voltage"=1, "high voltage"=2] ("range")
                n266 = local write "Voltage Range"("750V" ("Voltage Range")) -> ()
                n267 = local write "Current Range"("+/- 480A" ("Current Range")) -> ()
                n268 = Negate(x=w617) -> (-x=w616:dbl)
                n269 = property on="VOLTAGE" class="Knob (strict)"("Scale.Maximum"=750.0 ("Scale.Range:Maximum")) -> ()  [unwired: 2 in, 2 out]
                n270 = property on="CURRENT" class="Knob (strict)"("Scale.Maximum"=w617, "Scale.Minimum"=w616) -> ()  [unwired: 2 in, 2 out]
              }
              frame 2 {
                w622 = 240.0 ("Scale.Range:Maximum")
                (unwired) T25 2 items=["low voltage"=1, "high voltage"=2] ("range")
                n271 = local write "Voltage Range"("1500V" ("Voltage Range")) -> ()
                n272 = local write "Current Range"("+/- 240A" ("Current Range")) -> ()
                n273 = Negate(x=w622) -> (-x=w623:dbl)
                n274 = property on="VOLTAGE" class="Knob (strict)"("Scale.Maximum"=1500.0 ("Scale.Range:Maximum")) -> ()  [unwired: 2 in, 2 out]
                n275 = property on="CURRENT" class="Knob (strict)"("Scale.Maximum"=w622, "Scale.Minimum"=w623) -> ()  [unwired: 2 in, 2 out]
              }
            }
            n276 = Index Array(array=w581, index=w580) -> (element=w579:u64)
            n277 = Not(x=w587) -> (.not. x?=→"Output Disabled":bool)
            n278 = call "Get HPS Fault Code Info.vi"("fault code"=w579) -> ("fault enums"=w578:T22[], "is fault?"=→"Fault":bool)  [unwired: 8 in, 1 out]
            n279 = call "Get HPS Fault Code Description.vi"("fault code"=w579) -> ("fault description"=w575:string)  [unwired: 10 in]
            n280 = Divide(x=w610, y=sgl 1000.0) -> (x/y=→"Power Maximum":sgl)
            n281 = Search 1D Array(1D array=w578, element=w577) -> (index of element=w586:i32)  [unwired: 1 in]
            n282 = local write "Fault Description"(w575) -> ()
            n283 = local write "Fault Message"(w575) -> ()
            n284 = Greater Or Equal To 0?(x=w586) -> (x >= 0?=w585:bool)
            n285 = Divide(x=w608, y=sgl 1000.0) -> (x/y=→"Power Minimum":sgl)
            n286 = Select(t=u16 1, s=w585, f=u16 0 ("EMO Indicator")) -> (s? t:f=w584:u16)
            n287 = local write "EMO Indicator"(w584) -> ()
            n288 = Merge Errors(w596, w599, w600, w601, w603) -> (w602:errorcluster)
          }
        }
      }
      frame "---------- EIS ----------" {
        # "Do not put any code in this frame.\n(It is a separator no-op. You can make a copy of this frame to create a new UI frame)"
        n289 = call <vilib>:"Add State(s) to Queue__jki_lib_state_machine.vi"("State(s) in (\"\")"=w630) -> ("States Out"=w629:string)  [unwired: 14 in]
      }
      frame "EIS: Create Profile" {
        w661 = waveform(dbl) {"t0"=timestamp(0 s since 1904-01-01), "dt"=1.0, "Y"=[]} ("waveform out")
        w663 = waveform(dbl)[] [] ("EIS Profile")
        w675 = T10 1 items=["PEIS (Voltage)"=1, "GEIS (Current)"=2] ("x")
        # "convert RMS to PK-PK"
        n290 = Equal?(x=w675, y="EIS Mode") -> (x = y?=w645:bool)
        n291 = Equal?(x="EIS Stop Frequency", y="EIS Start Frequency") -> (x = y?=w636:bool)
        n292 = Subtract(x="EIS Start Frequency", y="EIS Stop Frequency") -> (x-y=w674:dbl)
        n293 = Divide(x="AC Signal (mV/mA RMS)", y=1000.0) -> (x/y=w654:dbl)
        n294 = Multiply(x="EIS Samples", y="EIS AC Step Delay") -> (x*y=w650:dbl)
        n295 = Quotient & Remainder(x=w674, y="EIS Delta Frequency") -> (floor(x/y)=w635:dbl)  [unwired: 1 out]
        n296 = Select(t="EIS DC Potential", s=w645, f="EIS DC Current") -> (s? t:f=w655:dbl)
        n297 = Select(t="EIS DC Current", s=w645, f="EIS DC Potential") -> (s? t:f=w656:dbl)
        n298 = To Long Integer(number=w650) -> (32bit integer=w649:i32)
        n299 = Select(t=1.0, s=w636, f=w635) -> (s? t:f=w634:dbl)
        n300 = Multiply(x=1.414, y=w654) -> (x*y=w653:dbl)
        n301 = Bundle By Name(cluster=cluster{"Fs":dbl, "#s":dbl} {"Fs"=100000.0, "#s"=1000.0} ("EIS Sampling Info"), "#s"="EIS Samples") -> (w644:cluster{"Fs":dbl, "#s":dbl})
        n302 = To Long Integer(number=w634) -> (32bit integer=w672:i32)
        n303 = Unbundle By Name(w644) -> ("Fs"=w643:dbl)
        n304 = for {
          N: w672 -> [_]
          tunnel: w655 -> [w705]
          tunnel: "EIS Delta Frequency" -> [w709]
          shift-right: [w710] -> _
          shift-left: "EIS Start Frequency" -> [w708]
          tunnel: w644 -> [w704]
          tunnel: [w691] -> w671 mode=indexing
          tunnel: [w707] -> w662
          tunnel: w653 -> [w706]
          tunnel: w656 -> [w683]
          shift-right: [w694] -> w646
          shift-left: w661 -> [w700]
          shift-right: [w690] -> w647
          shift-left: w661 -> [w699]
          tunnel: w649 -> [w680]
          tunnel: "EIS Samples" -> [w684]
          n305 = To Long Integer(number=w684) -> (32bit integer=w682:i32)
          n306 = Initialize Array(w683, w682) -> (w703:dbl[])
          n307 = call <vilib>:"Sine Waveform.vi"("sampling info"=w704, "error in (no error)"=w707, "amplitude"=w706, "frequency"=w708) -> ("error out"=w701:errorcluster, "signal out"=w698:waveform(dbl))  [unwired: 6 in]
          n308 = Unbundle By Name(w698) -> ("Y"=w702:dbl[])
          n309 = Bundle By Name(cluster=w698, "Y"=w703) -> (w679:waveform(dbl))
          n310 = Subtract(x=w708, y=w709) -> (x-y=w710:dbl)
          n311 = Add(x=w702, y=w705) -> (x+y=w689:dbl[])
          n312 = Reverse 1D Array(array=w689) -> (reversed array=w688:dbl[])
          n313 = Bundle By Name(cluster=w698, "Y"=w689) -> (w686:waveform(dbl))
          n314 = call-poly <vilib>:"Append Waveforms.vi"("error in (no error)"=w701, "waveform B"=w686, "waveform A"=w700) -> ("error out"=w697:errorcluster, "waveform out"=w696:waveform(dbl))  [unwired: 7 in]
          n315 = Index Array(array=w688) -> (element=w687:dbl)  [unwired: 1 in]
          n316 = Initialize Array(w687, w680) -> (w685:dbl[])
          n317 = Initialize Array(w683, w680) -> (w678:dbl[])
          n318 = Bundle By Name(cluster=w686, "Y"=w685) -> (w681:waveform(dbl))
          n319 = call-poly <vilib>:"Append Waveforms.vi"("error in (no error)"=w697, "waveform B"=w681, "waveform A"=w696) -> ("error out"=w695:errorcluster, "waveform out"=w694:waveform(dbl))  [unwired: 7 in]
          n320 = Bundle By Name(cluster=w679, "Y"=w678) -> (w677:waveform(dbl))
          n321 = call-poly <vilib>:"Append Waveforms.vi"("error in (no error)"=w695, "waveform B"=w679, "waveform A"=w699) -> ("error out"=w692:errorcluster, "waveform out"=w693:waveform(dbl))  [unwired: 7 in]
          n322 = call-poly <vilib>:"Append Waveforms.vi"("error in (no error)"=w692, "waveform B"=w677, "waveform A"=w693) -> ("error out"=w691:errorcluster, "waveform out"=w690:waveform(dbl))  [unwired: 7 in]
        }
        n323 = Reciprocal(x=w643) -> (1/x=w642:dbl)
        n324 = Multiply(x=1000000000.0, y=w642) -> (x*y=w640:dbl)
        n325 = To Quad Integer(1:w640) -> (0:w639:i64)
        n326 = local write "Profile Step dT (ns)"(w639) -> ()
        n327 = Build Array(w646, w647) -> (w660:waveform(dbl)[])
        n328 = Merge Errors(w671) -> (w670:errorcluster)
        n329 = Reverse 1D Array(array=w660) -> (reversed array=w659:waveform(dbl)[])
        n330 = Select(t=w660, s=w645, f=w659) -> (s? t:f=w658:waveform(dbl)[])
      }
      frame "EIS: Save Profile" {
        n331 = call "File Dialog2"("prompt"="Save EIS Profile", "error in"=w720, "pattern (all files)"="*.csv") -> ("selected path"=w719:path, "cancelled"=w718:bool, "error out"=w716:errorcluster)  [unwired: 9 in, 1 out]
        n332 = Or(x=w718, y=w716) -> (x .or. y?=w717:bool)
        n333 = case shown="False" w717 {
          tunnel: w719 -> [w730 _]
          tunnel: w716 -> [w740 w760]
          tunnel: [w725 w760] -> w713
          tunnel: w712 -> [w729 w759]
          tunnel: [w728 w759] -> w711
          frame False {
            # "min power\nmax power\nresistance\n\nare all constant"
            n334 = local read item#-1() -> (w755)
            n335 = local write "CSV Profile"(w730) -> ()
            n336 = for {
              tunnel: w755 -> [w758]
              tunnel: [w757] -> w753 mode=indexing
              tunnel: [w756] -> w750
              n337 = Unbundle By Name(w758) -> ("Y"=w757)
              n338 = Array Size(array=w757) -> (size(s)=w756:i32)
            }
            n339 = Open/Create/Replace File(file path (use dialog)=w730, error in=w740, operation (0:open)=T18."replace or create") -> (refnum out=w738:refnum<file>, error out=w739:errorcluster)  [unwired: 3 in, 1 out]
            n340 = Concatenate Strings("voltage,current,min_power,max_power,resistance" ("text"), "\r\n") -> (w732:string)
            n341 = Initialize Array(-150000.0 ("element"), w750) -> (w748:dbl[])
            n342 = Initialize Array(150000.0 ("element"), w750) -> (w747:dbl[])
            n343 = Initialize Array(0.0 ("element"), w750) -> (w746:dbl[])
            n344 = Write to Binary File(file (use dialog)=w738, data=w732, error in=w739, 5:FALSE ("prepend array or string size? (T)")) -> (refnum out=w735:refnum<file>, error out=w736:errorcluster)  [unwired: 2 in, 1 out]
            n345 = Close File(refnum=w735, error in=w736) -> (path=w741:path, error out=w742:errorcluster)
            n346 = Build Array (concatenate)(w753, w748, w747, w746) -> (w745:dbl[][])
            n347 = call-poly <vilib>:"Write Delimited Spreadsheet.vi"("file path (dialog if empty)"=w741, "2D data"=w745, "append to file? (new file:F)"=TRUE, "error in (no error)"=w742, "transpose? (no:F)"=TRUE, "delimiter (\\t)"="," ("delimiter (\\t)")) -> ("error out"=w725:errorcluster)  [unwired: 8 in, 1 out]
            n348 = Unbundle By Name(w725) -> ("status"=w724:bool)
            n349 = Not(x=w724) -> (.not. x?=w723:bool)
            n350 = call <vilib>:"Conditional State String__jki_lib_state_machine.vi"("Do State(s)?"=w723, "State"="Profile: Load" ("State(s) in Front (\"\")")) -> ("State Out"=w726:string)  [unwired: 7 in]
            n351 = call <vilib>:"Add State(s) to Queue__jki_lib_state_machine.vi"("State(s) in Front (\"\")"=w726, "State(s) in (\"\")"=w729) -> ("States Out"=w728:string)  [unwired: 13 in]
          }
          frame True {
          }
        }
      }
      frame "EIS: Generate Report" {
        # "#todo"
        n352 = disable-structure shown="Disabled" {
          disable-tunnel: w762 -> [w769 w770]
          disable-tunnel: [w768 w770] -> w761
          frame Disabled {
            # "prompt user file"
            n353 = call "File Dialog4"("prompt"="Save EIS Profile", "pattern (all files)"="*.csv") -> ()  [unwired: 10 in, 4 out]
            n354 = call "Generate EIS Plots.vi"("error in (no error)"=w769) -> ("error out"=w768:errorcluster)  [unwired: 8 in, 2 out]
          }
          frame Enabled {
          }
        }
      }
      frame "---------- HPS ----------" {
        # "Do not put any code in this frame.\n(It is a separator no-op. You can make a copy of this frame to create a new UI frame)"
        n355 = call <vilib>:"Add State(s) to Queue__jki_lib_state_machine.vi"("State(s) in (\"\")"=w775) -> ("States Out"=w774:string)  [unwired: 14 in]
      }
      frame "HPS: Connect" {
        # "If we fail to connect the unit,\nthen cancel the remaining steps"
        n356 = local read "TSN NIC IP Address"() -> (w787:string)
        n357 = local read "HPS Topology"() -> (w788:enum16{"SINGLE", "MULTI"})
        n358 = property on="HPS17K IP Addresses" class="Tree (strict)"() -> ("All Tags"=w784:string[])  [unwired: 2 in, 2 out]
        n359 = Index Array(array=w784) -> (element=w786:string)  [unwired: 1 in]
        n360 = call-poly <instrlib>:"Find GM ID.vi"("error in"=w785, "cycler IP address in"=w786) -> ("error out"=w794:errorcluster, "GM ID"=w790:string, "cycler IP address out"=w795:string)  [unwired: 7 in]
        "GM ID" <- w790
        n361 = case shown="\"SINGLE\", Default" w788 {
          tunnel: [w813 w825] -> w798
          tunnel: [w802 w821] -> w782
          tunnel: w795 -> [w818 _]
          tunnel: w794 -> [w817 w824]
          tunnel: [w816 w823] -> w791
          tunnel: w790 -> [w815 w822]
          tunnel: w787 -> [w801 w820]
          tunnel: w784 -> [_ w819]
          frame "SINGLE", Default {
            n362 = call-poly <instrlib>:"Initialize.vi"("intended GM ID"=w815, "error in"=w817, "TSN NIC IP address"=w801, "cycler IP address"=w818) -> ("error out"=w816:errorcluster, "events"=w812:T27, "HPS-17000 out"=w814:refnum<class "HPS-17000.lvclass">)  [unwired: 5 in]
            n363 = Unbundle By Name(w812) -> ("heartbeat failure event"=w810:refnum<user-event>, "faults event"=w808:refnum<user-event>, "network sync event"=w806:refnum<user-event>, "setpoint status event"=w804:refnum<user-event>)
            n364 = Build Array(w814) -> (w813:refnum<class "HPS-17000.lvclass">[])
            n365 = Build Array(w810) -> (w809:refnum<user-event>[])
            n366 = Build Array(w808) -> (w807:refnum<user-event>[])
            n367 = Build Array(w806) -> (w805:refnum<user-event>[])
            n368 = Build Array(w804) -> (w803:refnum<user-event>[])
            n369 = Bundle By Name(cluster=T12 {"heartbeats events"=[], "faults events"=[], "network sync event"=[], "setpoint status event"=[]} ("events"), "heartbeats events"=w809, "faults events"=w807, "network sync event"=w805, "setpoint status event"=w803) -> (w802:T12)
          }
          frame "MULTI" {
            n370 = call-poly <instrlib>:"Initialize.vi"("intended GM ID"=w822, "error in"=w824, "TSN NIC IP address"=w820, "cycler IP addresses"=w819) -> ("error out"=w823:errorcluster, "events"=w821:T12, "cycler refs out"=w825:refnum<class "HPS-17000.lvclass">[])  [unwired: 5 in]
          }
        }
        n371 = Unbundle By Name(w791) -> ("status"=w796:bool)
        n372 = Not(x=w796) -> (.not. x?=w777:bool)
        n373 = Select(t=w781, s=w777, f="UI: Connection Failed") -> (s? t:f=w780:string)
        n374 = Select(t="HPS17K Panel - Connected" ("Front Panel Window:Title"), s=w777, f="HPS17K Panel" ("Front Panel Window:Title")) -> (s? t:f=w776:string)
        n375 = local write "HPS Connect"(w777) -> ()
        n376 = Select(t=T14."Enabled" ("Disabled"), s=w777, f=T14."Disabled and Grayed Out" ("Disabled")) -> (s? t:f=w789:T14)
        n377 = property class="VI"("Front Panel.Title"=w776) -> ()  [unwired: 2 in, 2 out]
        n378 = property on="Get Device Properties" class="Bool"("DisabledEnum"=w789) -> ()  [unwired: 2 in, 2 out]
        n379 = property on="HPS Clear" class="Bool"("DisabledEnum"=w789) -> ()  [unwired: 2 in, 2 out]
        n380 = property on="HPS Reserve" class="Bool (strict)"("DisabledEnum"=w789) -> ()  [unwired: 2 in, 2 out]
        n381 = property on="Launch Test Server" class="Bool (strict)"("DisabledEnum"=w789) -> ()  [unwired: 2 in, 2 out]
        n382 = property on="Get XC Report" class="Bool"("DisabledEnum"=w789) -> ()  [unwired: 2 in, 2 out]
        n383 = property on="FC Sys Inspect" class="Bool"("DisabledEnum"=w789) -> ()  [unwired: 2 in, 2 out]
        n384 = property on="Volta Monitor" class="Bool"("DisabledEnum"=w789) -> ()  [unwired: 2 in, 2 out]
        n385 = Bundle By Name(cluster=w800, "HPS17K Events"=w782, "HPS17K Refs"=w798, "Connected"=w777) -> (w799:T13)
      }
      frame "HPS: Disconnect" {
        n386 = Unbundle By Name(w838) -> ("HPS17K Refs"=w837:refnum<class "HPS-17000.lvclass">[])
        n387 = call-poly <instrlib>:"Close.vi"("error in"=w840, "cycler refs in"=w837) -> ("error out"=w835:errorcluster)  [unwired: 9 in]
        n388 = Unbundle By Name(w835) -> ("status"=w826:bool)
        n389 = Bundle By Name(cluster=w838, "HPS17K Refs"=refnum<class "HPS-17000.lvclass">[] [], "HPS17K Events"=T12 {"heartbeats events"=[], "faults events"=[], "network sync event"=[], "setpoint status event"=[]}, "Connected"=w826) -> (w839:T13)
        n390 = local write "HPS Connect"(w826) -> ()
        n391 = Select(t="HPS17K Panel - Connected" ("Front Panel Window:Title"), s=w826, f="HPS17K Panel" ("Front Panel Window:Title")) -> (s? t:f=w829:string)
        n392 = Select(t=T14."Enabled" ("Disabled"), s=w826, f=T14."Disabled and Grayed Out" ("Disabled")) -> (s? t:f=w832:T14)
        n393 = property class="VI"("Front Panel.Title"=w829) -> ()  [unwired: 2 in, 2 out]
        n394 = property on="HPS Reserve" class="Bool (strict)"("DisabledEnum"=w832) -> ()  [unwired: 2 in, 2 out]
        n395 = property on="Get Device Properties" class="Bool"("DisabledEnum"=w832) -> ()  [unwired: 2 in, 2 out]
        n396 = property on="Launch Test Server" class="Bool (strict)"("DisabledEnum"=w832) -> ()  [unwired: 2 in, 2 out]
        n397 = property on="Get XC Report" class="Bool"("DisabledEnum"=w832) -> ()  [unwired: 2 in, 2 out]
        n398 = property on="FC Sys Inspect" class="Bool"("DisabledEnum"=w832) -> ()  [unwired: 2 in, 2 out]
        n399 = property on="Volta Monitor" class="Bool"("DisabledEnum"=w832) -> ()  [unwired: 2 in, 2 out]
        n400 = property on="HPS Clear" class="Bool"("DisabledEnum"=w832) -> ()  [unwired: 2 in, 2 out]
      }
      frame "HPS: Reserve" {
        w845 = T14."Disabled and Grayed Out" ("Disabled")
        w848 = T14."Enabled" ("Disabled")
        # "If we fail to reserve the unit,\nthen cancel the remaining steps"
        n401 = Unbundle By Name(w862) -> ("Profile Setpoints"=w844:T11[], "HPS17K Refs"=w863:refnum<class "HPS-17000.lvclass">[], "Reserved"=w858:bool)
        n402 = case shown="False" w858 {
          selector: w858 -> [_ w871]
          tunnel: w864 -> [w870 w872]
          tunnel: w863 -> [w869 w873]
          tunnel: [w868 w873] -> w860
          tunnel: [w867 w872] -> w859
          tunnel: [w866 w871] -> w849
          frame False {
            n403 = call-poly <instrlib>:"Reserve.vi"("error in"=w870, "cycler refs in"=w869) -> ("error out"=w867:errorcluster, "successful"=w866:bool, "cycler refs out"=w868:refnum<class "HPS-17000.lvclass">[])  [unwired: 7 in]
          }
          frame True {
          }
        }
        n404 = Empty Array?(array=w844) -> (empty?=w843:bool)
        n405 = Not(x=w843) -> (.not. x?=w842:bool)
        n406 = Select(t=w856, s=w849, f="UI: Reservation Failed") -> (s? t:f=w854:string)
        n407 = Bundle By Name(cluster=w862, "HPS17K Refs"=w860, "Reserved"=w849) -> (w861:T13)
        n408 = And(x=w842, y=w849) -> (x .and. y?=w846:bool)
        n409 = local write "HPS Reserve"(w849) -> ()
        n410 = Select(t="HPS17K Panel - Reserved" ("Front Panel Window:Title"), s=w849, f="HPS17K Panel" ("Front Panel Window:Title")) -> (s? t:f=w853:string)
        n411 = Select(t=w848, s=w849, f=w845) -> (s? t:f=w850:T14)
        n412 = Select(t=w848, s=w846, f=w845) -> (s? t:f=w847:T14)
        n413 = Select(t=w845, s=w849, f=w848) -> (s? t:f=w857:T14)
        n414 = property class="VI"("Front Panel.Title"=w853) -> ()  [unwired: 2 in, 2 out]
        n415 = property on="Apply Mode & Range" class="Bool"("DisabledEnum"=w850) -> ()  [unwired: 2 in, 2 out]
        n416 = property on="Apply Limits" class="Bool"("DisabledEnum"=w850) -> ()  [unwired: 2 in, 2 out]
        n417 = property on="Apply Slew Rates" class="Bool"("DisabledEnum"=w850) -> ()  [unwired: 2 in, 2 out]
        n418 = property on="High Speed" class="Bool (strict)"("DisabledEnum"=w850) -> ()  [unwired: 2 in, 2 out]
        n419 = property on="Start Profile" class="Bool (strict)"("DisabledEnum"=w847) -> ()  [unwired: 2 in, 2 out]
        n420 = property on="HPS Clear" class="Bool"("DisabledEnum"=w857) -> ()  [unwired: 2 in, 2 out]
        n421 = property on="Apply Setpoints" class="Bool"("DisabledEnum"=w850) -> ()  [unwired: 2 in, 2 out]
        n422 = property on="Energize" class="Bool (strict)"("DisabledEnum"=w850) -> ()  [unwired: 2 in, 2 out]
        n423 = property on="Output" class="Bool (strict)"("DisabledEnum"=w850) -> ()  [unwired: 2 in, 2 out]
      }
      frame "HPS: Unreserve" {
        w880 = T14."Disabled and Grayed Out" ("Disabled")
        w879 = T14."Enabled" ("Disabled")
        n424 = Unbundle By Name(w887) -> ("HPS17K Refs"=w884:refnum<class "HPS-17000.lvclass">[])
        n425 = call-poly <instrlib>:"Unreserve.vi"("error in"=w885, "cycler refs in"=w884) -> ("error out"=w882:errorcluster, "cycler refs out"=w883:refnum<class "HPS-17000.lvclass">[])  [unwired: 8 in]
        n426 = Unbundle By Name(w882) -> ("status"=w875:bool)
        n427 = local write "HPS Reserve"(w875) -> ()
        n428 = Bundle By Name(cluster=w887, "HPS17K Refs"=w883, "Reserved"=w875) -> (w886:T13)
        n429 = Select(t="HPS17K Panel - Reserved" ("Front Panel Window:Title"), s=w875, f="HPS17K Panel - Connected" ("Front Panel Window:Title")) -> (s? t:f=w878:string)
        n430 = Select(t=w880, s=w875, f=w879) -> (s? t:f=w881:T14)
        n431 = Select(t=w879, s=w875, f=w880) -> (s? t:f=w874:T14)
        n432 = property class="VI"("Front Panel.Title"=w878) -> ()  [unwired: 2 in, 2 out]
        n433 = property on="HPS Clear" class="Bool"("DisabledEnum"=w881) -> ()  [unwired: 2 in, 2 out]
        n434 = property on="Apply Mode & Range" class="Bool"("DisabledEnum"=w874) -> ()  [unwired: 2 in, 2 out]
        n435 = property on="Apply Limits" class="Bool"("DisabledEnum"=w874) -> ()  [unwired: 2 in, 2 out]
        n436 = property on="Apply Setpoints" class="Bool"("DisabledEnum"=w874) -> ()  [unwired: 2 in, 2 out]
        n437 = property on="Energize" class="Bool (strict)"("DisabledEnum"=w874) -> ()  [unwired: 2 in, 2 out]
        n438 = property on="Output" class="Bool (strict)"("DisabledEnum"=w874) -> ()  [unwired: 2 in, 2 out]
        n439 = property on="Apply Slew Rates" class="Bool"("DisabledEnum"=w874) -> ()  [unwired: 2 in, 2 out]
        n440 = property on="High Speed" class="Bool (strict)"("DisabledEnum"=w874) -> ()  [unwired: 2 in, 2 out]
        n441 = property on="Start Profile" class="Bool (strict)"("DisabledEnum"=w874) -> ()  [unwired: 2 in, 2 out]
      }
      frame "HPS: Clear" {
        n442 = Unbundle By Name(w898) -> ("HPS17K Refs"=w895:refnum<class "HPS-17000.lvclass">[])
        n443 = call-poly <instrlib>:"Clear Reservation.vi"("error in"=w896, "cycler refs in"=w895) -> ("error out"=w894:errorcluster, "clear reserve tokens"=w892:string[], "cycler refs out"=w893:refnum<class "HPS-17000.lvclass">[])  [unwired: 7 in]
        n444 = call-poly <instrlib>:"Clear Reservation Confirmation.vi"("error in"=w894, "clear reserve tokens"=w892, "cycler refs in"=w893) -> ("error out"=w891:errorcluster, "cycler refs out"=w890:refnum<class "HPS-17000.lvclass">[])  [unwired: 7 in]
        n445 = Bundle By Name(cluster=w898, "HPS17K Refs"=w890) -> (w897:T13)
      }
      frame "HPS: Apply Setpoints" {
        n446 = Unbundle By Name(w908) -> ("HPS17K Refs"=w905:refnum<class "HPS-17000.lvclass">[], "Connected"=w903:bool, "Grapher Ref"=w901:refnum<class "Grapher.lvclass">)
        n447 = case shown="True" w903 {
          tunnel: w902 -> [w911 w916]
          tunnel: [w911 w932] -> w906
          tunnel: w905 -> [w912 w931]
          tunnel: [w912 w930] -> w904
          tunnel: w901 -> [_ w915]
          frame False {
          }
          frame True {
            n448 = call "Get Timestamp.vi"("reference in"=w915, "Error In"=w916) -> ("timestamp (seconds)"=w914:dbl, "Error Out"=w913:errorcluster)  [unwired: 15 in, 1 out]
            n449 = Multiply(x=1000000000.0, y=w914) -> (x*y=w921:dbl)
            n450 = To Quad Integer(1:w921) -> (0:w920:i64)
            n451 = Add(x=w920, y=i64 100000000) -> (x+y=w917:i64)
            n452 = Unbundle By Name("Setpoints") -> ("Voltage"=w926:sgl, "Current"=w925:sgl, "Minimum Power"=w924:sgl, "Maximum Power"=w923:sgl, "Resistance"=w922:sgl)
            n453 = Bundle By Name(cluster=T11 {"voltage"=3.0, "current"=5.0, "min_power"=6.0, "max_power"=0.0, "resistance"=7.0} ("setpoint"), "voltage"=w926, "current"=w925, "min_power"=w924, "max_power"=w923, "resistance"=w922) -> (w928:T11)
            n454 = call-poly <instrlib>:"Write Setpoint.vi"("timestamp"=w917, "error in"=w913, "setpoint"=w928, "cycler refs in"=w931) -> ("error out"=w932:errorcluster, "cycler refs out"=w930:refnum<class "HPS-17000.lvclass">[])  [unwired: 6 in]
          }
        }
        n455 = Bundle By Name(cluster=w908, "HPS17K Refs"=w904) -> (w907:T13)
      }
      frame "HPS: Set Mode and Range" {
        n456 = Unbundle By Name(w939) -> ("HPS17K Refs"=w935:refnum<class "HPS-17000.lvclass">[], "Connected"=w933:bool)
        n457 = case shown="True" w933 {
          tunnel: w937 -> [w943 w951]
          tunnel: [w943 w950] -> w936
          tunnel: w935 -> [w944 w948]
          tunnel: [w944 w949] -> w934
          frame False {
          }
          frame True {
            n458 = Unbundle By Name("Mode & Range") -> ("Mode"=w947:T6, "Range"=w946:T7)
            n459 = call-poly <instrlib>:"Set Mode.vi"("error in"=w951, "range"=w946, "mode"=w947, "cycler refs in"=w948) -> ("error out"=w950:errorcluster, "cycler refs out"=w949:refnum<class "HPS-17000.lvclass">[])  [unwired: 6 in]
          }
        }
        n460 = Bundle By Name(cluster=w939, "HPS17K Refs"=w934) -> (w938:T13)
        n461 = call <vilib>:"Add State(s) to Queue__jki_lib_state_machine.vi"("State(s) in (\"\")"=w942) -> ("States Out"=w941:string)  [unwired: 14 in]
      }
      frame "HPS: Set Limits" {
        n462 = Unbundle By Name(w958) -> ("HPS17K Refs"=w954:refnum<class "HPS-17000.lvclass">[], "Connected"=w952:bool)
        n463 = case shown="True" w952 {
          tunnel: w956 -> [w962 w968]
          tunnel: [w962 w967] -> w955
          tunnel: w954 -> [w963 w965]
          tunnel: [w963 w966] -> w953
          frame False {
          }
          frame True {
            n464 = call-poly <instrlib>:"Set Limits.vi"("error in"=w968, "limits"="Limits", "cycler refs in"=w965) -> ("error out"=w967:errorcluster, "cycler refs out"=w966:refnum<class "HPS-17000.lvclass">[])  [unwired: 7 in]
          }
        }
        n465 = Bundle By Name(cluster=w958, "HPS17K Refs"=w953) -> (w957:T13)
        n466 = call <vilib>:"Add State(s) to Queue__jki_lib_state_machine.vi"("State(s) in (\"\")"=w961) -> ("States Out"=w960:string)  [unwired: 14 in]
      }
      frame "HPS: Energize" {
        n467 = Unbundle By Name(w975) -> ("HPS17K Refs"=w971:refnum<class "HPS-17000.lvclass">[], "Connected"=w969:bool)
        n468 = case shown="True" w969 {
          tunnel: w973 -> [w978 w984]
          tunnel: [w978 w983] -> w972
          tunnel: w971 -> [w979 w982]
          tunnel: [w979 w981] -> w970
          frame False {
          }
          frame True {
            n469 = call-poly <instrlib>:"Set Energized.vi"("error in"=w984, "energize (T)"="Energize", "cycler refs in"=w982) -> ("error out"=w983:errorcluster, "cycler refs out"=w981:refnum<class "HPS-17000.lvclass">[])  [unwired: 7 in]
          }
        }
        n470 = Bundle By Name(cluster=w975, "HPS17K Refs"=w970) -> (w974:T13)
      }
      frame "HPS: Output" {
        n471 = Unbundle By Name(w991) -> ("HPS17K Refs"=w987:refnum<class "HPS-17000.lvclass">[], "Connected"=w985:bool)
        n472 = case shown="True" w985 {
          tunnel: w989 -> [w994 w999]
          tunnel: [w994 w998] -> w988
          tunnel: w987 -> [w995 w1000]
          tunnel: [w995 w997] -> w986
          frame False {
          }
          frame True {
            n473 = call-poly <instrlib>:"Set Enabled Output.vi"("error in"=w999, "enabled output"="Output", "cycler refs in"=w1000) -> ("error out"=w998:errorcluster, "cycler refs out"=w997:refnum<class "HPS-17000.lvclass">[])  [unwired: 7 in]
          }
        }
        n474 = Bundle By Name(cluster=w991, "HPS17K Refs"=w986) -> (w990:T13)
      }
      frame "HPS: Start Measurement Stream" {
        n475 = Unbundle By Name(w1003) -> ("HPS17K Refs"=w1009:refnum<class "HPS-17000.lvclass">[], "Connected"=w1007:bool, "Measurement Stream"=w1004:bool, "Grapher Ref"=w1001:refnum<class "Grapher.lvclass">)
        n476 = Not(x=w1004) -> (.not. x?=w1006:bool)
        n477 = And(x=w1007, y=w1006) -> (x .and. y?=w1005:bool)
        n478 = case shown="True" w1005 {
          tunnel: w1011 -> [w1016 w1021]
          tunnel: [w1016 w1027] -> w1010
          tunnel: w1009 -> [w1017 w1029]
          tunnel: [w1017 w1028] -> w1008
          tunnel: [w1015 w1030] -> w1002
          tunnel: w1004 -> [w1015 _]
          tunnel: w1001 -> [_ w1020]
          frame False {
          }
          frame True {
            n479 = call "Get Timestamp.vi"("reference in"=w1020, "Error In"=w1021) -> ("timestamp (seconds)"=w1018:dbl, "Error Out"=w1019:errorcluster)  [unwired: 15 in, 1 out]
            n480 = Multiply(x=1000000000.0, y=w1018) -> (x*y=w1022:dbl)
            n481 = To Unsigned Quad Integer(1:w1022) -> (0:w1026:u64)
            n482 = Add(x=w1026, y=u64 1000000000) -> (x+y=w1024:u64)
            n483 = call-poly <instrlib>:"Start Measurement Stream.vi"("error in"=w1019, "start timestamp"=w1024, "cycler refs in"=w1029) -> ("error out"=w1027:errorcluster, "cycler refs out"=w1028:refnum<class "HPS-17000.lvclass">[])  [unwired: 7 in]
            n484 = Unbundle By Name(w1027) -> ("status"=w1031:bool)
            n485 = Not(x=w1031) -> (.not. x?=w1030:bool)
          }
        }
        n486 = local write "Measurement Stream"(w1002) -> ()
        n487 = Bundle By Name(cluster=w1003, "HPS17K Refs"=w1008, "Measurement Stream"=w1002) -> (w1012:T13)
      }
      frame "HPS: Stop Measurement Stream" {
        n488 = Unbundle By Name(w1041) -> ("HPS17K Refs"=w1037:refnum<class "HPS-17000.lvclass">[], "Connected"=w1035:bool, "Measurement Stream"=w1033:bool)
        n489 = And(x=w1035, y=w1033) -> (x .and. y?=w1034:bool)
        n490 = case shown="True" w1034 {
          tunnel: w1039 -> [w1045 w1052]
          tunnel: [w1045 w1050] -> w1038
          tunnel: w1037 -> [w1046 w1053]
          tunnel: [w1046 w1051] -> w1036
          tunnel: [w1044 w1048] -> w1032
          tunnel: w1033 -> [w1044 _]
          frame False {
          }
          frame True {
            n491 = call-poly <instrlib>:"Stop Measurement Stream.vi"("error in"=w1052, "cycler refs in"=w1053) -> ("error out"=w1050:errorcluster, "cycler refs out"=w1051:refnum<class "HPS-17000.lvclass">[])  [unwired: 8 in]
            n492 = local read "High Speed"() -> (w1047:bool)
            n493 = Unbundle By Name(w1050) -> ("status"=w1048:bool)
            n494 = Select(t=w1047, s=w1048, f=w1048) -> (s? t:f=w1049:bool)
            n495 = local write "High Speed"(w1049) -> ()
          }
        }
        n496 = local write "Measurement Stream"(w1032) -> ()
        n497 = Bundle By Name(cluster=w1041, "HPS17K Refs"=w1036, "Measurement Stream"=w1032) -> (w1040:T13)
      }
      frame "HPS: Start Setpoint Stream" {
        n498 = Format Into String(format string="%s: Starting Setpoint Stream", w1054) -> (resulting string=w1056:string)  [unwired: 2 in, 1 out]
        n499 = local write "Status Message"(w1056) -> ()
        n500 = Unbundle By Name(w1060) -> ("HPS17K Refs"=w1065:refnum<class "HPS-17000.lvclass">[], "Connected"=w1063:bool, "Setpoint Stream"=w1058:bool)
        n501 = Not(x=w1058) -> (.not. x?=w1062:bool)
        n502 = And(x=w1063, y=w1062) -> (x .and. y?=w1061:bool)
        n503 = case shown="True" w1061 {
          tunnel: w1067 -> [w1071 w1077]
          tunnel: [w1071 w1076] -> w1066
          tunnel: w1065 -> [w1072 w1079]
          tunnel: [w1072 w1078] -> w1064
          tunnel: [w1070 w1074] -> w1059
          tunnel: w1058 -> [w1070 _]
          frame False {
          }
          frame True {
            n504 = call-poly <instrlib>:"Start Setpoint Stream.vi"("error in"=w1077, "setpoint stream config"=T19 {"local address"="224.1.0.0", "receiver port"=61557}, "cycler refs in"=w1079) -> ("error out"=w1076:errorcluster, "cycler refs out"=w1078:refnum<class "HPS-17000.lvclass">[])  [unwired: 7 in]
            n505 = Unbundle By Name(w1076) -> ("status"=w1075:bool)
            n506 = Not(x=w1075) -> (.not. x?=w1074:bool)
          }
        }
        n507 = Bundle By Name(cluster=w1060, "HPS17K Refs"=w1064, "Setpoint Stream"=w1059) -> (w1068:T13)
        n508 = local write "Setpoint Stream"(w1059) -> ()
      }
      frame "HPS: Update Setpoint Stream" {
        n509 = Unbundle By Name(w1088) -> ("HPS17K Refs"=w1084:refnum<class "HPS-17000.lvclass">[], "Profile Setpoints"=w1081:T11[], "Connected"=w1082:bool, "Grapher Ref"=w1080:refnum<class "Grapher.lvclass">)
        n510 = case shown="True" w1082 {
          tunnel: w1086 -> [w1091 w1096]
          tunnel: [w1091 w1106] -> w1085
          tunnel: w1084 -> [w1092 w1105]
          tunnel: [w1092 w1104] -> w1083
          tunnel: w1081 -> [_ w1103]
          tunnel: w1080 -> [_ w1093]
          frame False {
          }
          frame True {
            n511 = call "Get Timestamp.vi"("reference in"=w1093, "Error In"=w1096) -> ("timestamp (seconds)"=w1094:dbl, "Error Out"=w1095:errorcluster)  [unwired: 15 in, 1 out]
            n512 = Multiply(x=1000000000.0, y=w1094) -> (x*y=w1101:dbl)
            n513 = local read "Profile Step dT (ns)"() -> (w1097:i64)
            n514 = To Quad Integer(1:w1101) -> (0:w1102:i64)
            n515 = Add(x=w1102, y=i64 5000000000) -> (x+y=w1098:i64)
            n516 = call-poly <instrlib>:"Stream Setpoints.vi"("dt"=w1097, "t0"=w1098, "error in"=w1095, "setpoints"=w1103, "cycler refs in"=w1105) -> ("error out"=w1106:errorcluster, "cycler refs out"=w1104:refnum<class "HPS-17000.lvclass">[])  [unwired: 5 in]
          }
        }
        n517 = Bundle By Name(cluster=w1088, "HPS17K Refs"=w1083) -> (w1087:T13)
      }
      frame "HPS: Stop Setpoint Stream" {
        n518 = Unbundle By Name(w1108) -> ("HPS17K Refs"=w1113:refnum<class "HPS-17000.lvclass">[], "Connected"=w1111:bool, "Setpoint Stream"=w1109:bool)
        n519 = And(x=w1111, y=w1109) -> (x .and. y?=w1110:bool)
        n520 = case shown="True" w1110 {
          tunnel: w1115 -> [w1120 w1124]
          tunnel: [w1120 w1123] -> w1114
          tunnel: w1113 -> [w1121 w1126]
          tunnel: [w1121 w1125] -> w1112
          tunnel: [w1119 w1122] -> w1107
          tunnel: w1109 -> [w1119 _]
          frame False {
          }
          frame True {
            n521 = call-poly <instrlib>:"Stop Setpoint Stream.vi"("error in"=w1124, "cycler refs in"=w1126) -> ("error out"=w1123:errorcluster, "cycler refs out"=w1125:refnum<class "HPS-17000.lvclass">[])  [unwired: 8 in]
            n522 = Unbundle By Name(w1123) -> ("status"=w1122:bool)
          }
        }
        n523 = Bundle By Name(cluster=w1108, "HPS17K Refs"=w1112, "Setpoint Stream"=w1107) -> (w1116:T13)
        n524 = local write "Setpoint Stream"(w1107) -> ()
        n525 = local write "Start Profile"(w1107) -> ()
      }
      frame "HPS: Get Diagnostic Data" {
        n526 = Unbundle By Name(w1131) -> ("HPS17K Refs"=w1135:refnum<class "HPS-17000.lvclass">[], "Connected"=w1133:bool)
        n527 = local read "Cycler Selection"() -> (w1130:i16)
        n528 = In Range and Coerce(upper limit=i16 50, x=w1130, lower limit=i16 0) -> (coerced(x)=w1128:i16)  [unwired: 1 out]
        n529 = case shown="True" w1133 {
          tunnel: w1137 -> [w1138 w1150]
          tunnel: [w1138 w1151] -> w1136
          tunnel: w1135 -> [_ w1141]
          tunnel: w1128 -> [_ w1139]
          frame False {
          }
          frame True {
            n530 = Index Array(array=w1141, index=w1139) -> (element=w1140:refnum<class "HPS-17000.lvclass">)
            n531 = call "File Dialog"("prompt"="Select a file path for the diagnostic report", "default name"="xc_report.zip", "error in"=w1150, "pattern (all files)"="*.zip", "pattern label"="Compressed XC Report") -> ("selected path"=w1142:path, "cancelled"=w1149:bool, "error out"=w1148:errorcluster)  [unwired: 7 in, 1 out]
            n532 = Or(x=w1149, y=w1148) -> (x .or. y?=w1147:bool)
            n533 = case shown="False" w1147 {
              tunnel: w1140 -> [w1154 _]
              tunnel: [w1153 w1164] -> w1151
              tunnel: w1148 -> [w1162 w1164]
              tunnel: w1142 -> [w1155 _]
              frame False {
                w1152 = 60000  # timeout in ms (60000)
                w1158 = 128  # call & forget
                n534 = vi-ref "Get XC Report.vi"() -> (w1163:refnum<vi>)
                n535 = property class="VI Interface Type 2"(reference=w1163, error in=w1162) -> (reference out=w1160:refnum<vi>, error out=w1161:errorcluster, "Path"=w1159:path)
                n536 = Open VI Reference(type specifier VI Refnum (for type only)=w1160, vi path=w1159, options=w1158, error in (no error)=w1161) -> (vi reference=w1157:refnum<vi>, error out=w1156:errorcluster)  [unwired: 2 in]
                n537 = call-by-ref "Start Asynchronous Call"(reference=w1157, error in=w1156, "timeout in ms (60000)"=w1152, "selected path"=w1155, "HPS-17000 in"=w1154) -> (error out=w1153:errorcluster)  [unwired: 7 in, 3 out]
              }
              frame True {
              }
            }
          }
        }
      }
      frame "---------- Profile ----------" {
        # "Do not put any code in this frame.\n(It is a separator no-op. You can make a copy of this frame to create a new UI frame)"
      }
      frame "Profile: Load" {
        n538 = call-poly <vilib>:"Read Delimited Spreadsheet.vi"("file path (dialog if empty)"="CSV Profile", "error in (no error)"=w1177, "delimiter (\\t)"="," ("delimiter (\\t)")) -> ("all rows"=w1172:dbl[][], "error out"=w1174:errorcluster)  [unwired: 7 in, 4 out]
        n539 = To Single Precision Float(number=w1172) -> (single precision float=w1171:sgl[][])
        n540 = case shown="No Error" w1174 {
          selector: w1174 -> [w1213 w1229]
          tunnel: [w1213 w1229] -> w1173
          tunnel: w1171 -> [w1198 _]
          tunnel: w1169 -> [w1211 w1228]
          tunnel: [w1210 w1228] -> w1170
          tunnel: w1169 -> [w1184 _]
          frame No Error {
            w1181 = 1500  # max profile steps
            # "#note\n\nwarning about decimated profile resolution for profiles larger than 1500 steps"
            # "remove header\nrow"
            n541 = Unbundle By Name(w1184) -> ("Reserved"=w1183:bool)
            n542 = Delete From Array(array=w1198, index (row)=0) -> (array with subset deleted=w1192:sgl[][])  [unwired: 2 in, 1 out]
            n543 = Index Array(array=w1192, index (col) #1=0 ("disabled index (col)"), index (col) #2=1 ("index (col)")) -> (element #1=w1201:sgl[], element #2=w1203:sgl[])  [unwired: 2 in]
            n544 = local read "Profile Step dT (ns)"() -> (w1207:i64)
            n545 = Array Size(array=w1192) -> (size(s)=w1200:i32[])
            n546 = local write "Main Tab Control"(T2."PROFILE" ("Main Tab Control")) -> ()
            n547 = Index Array(array=w1200, index=0) -> (element=w1193:i32)
            n548 = Divide(x=w1193, y=w1181) -> (x/y=w1196:dbl)
            n549 = Divide(x=w1207, y=i64 1000000000) -> (x/y=w1204:dbl)
            n550 = Less Or Equal?(x=w1193, y=w1181) -> (x <= y?=w1197:bool)
            n551 = Round Toward +Infinity(x=w1196) -> (ceil(x): smallest int >= x=w1195:dbl)
            n552 = Select(t=T14."Enabled" ("Disabled"), s=w1183, f=T14."Disabled and Grayed Out" ("Disabled")) -> (s? t:f=w1185:T14)
            n553 = Bundle By Name(cluster=waveform(sgl) {"t0"=timestamp(0 s since 1904-01-01), "dt"=1.0, "Y"=[]} ("waveform"), "dt"=w1204) -> (w1189:waveform(sgl))
            n554 = To Long Integer(number=w1195) -> (32bit integer=w1194:i32)
            n555 = Bundle By Name(cluster=w1189, "Y"=w1201) -> (w1202:waveform(sgl))
            n556 = Bundle By Name(cluster=w1189, "Y"=w1203) -> (w1190:waveform(sgl))
            n557 = for {
              tunnel: w1198 -> [w1226] mode=indexing
              workers-P: _ -> [_]
              tunnel: [w1220] -> w1182 mode=indexing if=w1214
              tunnel: w1194 -> [w1218]
              tunnel: w1197 -> [w1215]
              i -> [w1219]
              n558 = Index Array(array=w1226) -> (element #1=w1225:sgl, element #2=w1224:sgl, element #3=w1223:sgl, element #4=w1222:sgl, element #5=w1221:sgl)  [unwired: 5 in]
              n559 = Quotient & Remainder(x=w1219, y=w1218) -> (x-y*floor(x/y)=w1217:i32)  [unwired: 1 out]
              n560 = Equal To 0?(x=w1217) -> (x = 0?=w1216:bool)
              n561 = Bundle By Name(cluster=T11 {"voltage"=0.0, "current"=0.0, "min_power"=0.0, "max_power"=0.0, "resistance"=0.0} ("nibatterycycler_grpc_Setpoint"), "voltage"=w1225, "current"=w1224, "min_power"=w1223, "max_power"=w1222, "resistance"=w1221) -> (w1220:T11)
              n562 = Or(x=w1216, y=w1215) -> (x .or. y?=w1214:bool)
            }
            n563 = property on="Start Profile" class="Bool (strict)"("DisabledEnum"=w1185) -> ()  [unwired: 2 in, 2 out]
            n564 = Build Array(w1202, w1190) -> (→"CSV Profile":waveform(sgl)[])
            n565 = Array Subset(array=w1182, length=w1181) -> (w1180:T11[])  [unwired: 1 in]
            n566 = Bundle By Name(cluster=w1211, "Profile Setpoints"=w1180) -> (w1210:T13)
          }
          frame Error {
          }
        }
      }
      frame "Profile: Unload" {
        n567 = Bundle By Name(cluster=w1233, "Profile Setpoints"=T11[] []) -> (w1232:T13)
      }
      frame "---------- Scripts ----------" {
        # "Do not put any code in this frame.\n(It is a separator no-op. You can make a copy of this frame to create a new UI frame)"
      }
      frame "Script: Launch Streamer" {
        n568 = Unbundle By Name(w1247) -> ("Graph Queue"=w1243:refnum<queue>, "Logger Queue"=w1242:refnum<queue>, "HPS17K Refs"=w1240:refnum<class "HPS-17000.lvclass">[], "Streamer Ref"=w1241:refnum<class "Streamer.lvclass">)
        n569 = Equal?(x=w1241, y=refnum<class "Streamer.lvclass"> refnum) -> (x = y?=w1245:bool)
        n570 = case shown="True" w1245 {
          tunnel: [w1252 w1259] -> w1248
          tunnel: w1249 -> [w1252 w1258]
          tunnel: w1247 -> [w1253 w1262]
          tunnel: [w1253 w1261] -> w1246
          tunnel: w1243 -> [_ w1257]
          tunnel: w1242 -> [_ w1256]
          tunnel: w1240 -> [_ w1254]
          frame False {
          }
          frame True {
            n571 = Build Array(w1257, w1256) -> (w1255:refnum<queue>[])
            n572 = call "Streamer_Create.vi"("Stream Queues"=w1255, "HPS17K Refs"=w1254, "Error In"=w1258) -> ("reference out"=w1260:refnum<class "Streamer.lvclass">, "Error Out"=w1259:errorcluster)  [unwired: 15 in]
            n573 = Bundle By Name(cluster=w1262, "Streamer Ref"=w1260) -> (w1261:T13)
          }
        }
      }
      frame "Script: Launch Logger" {
        n574 = Unbundle By Name(w1269) -> ("Logger Queue"=w1265:refnum<queue>, "HPS17K Refs"=w1263:refnum<class "HPS-17000.lvclass">[], "Logger Ref"=w1264:refnum<class "Logger.lvclass">)
        n575 = Equal?(x=w1264, y=refnum<class "Logger.lvclass"> refnum) -> (x = y?=w1267:bool)
        n576 = case shown="True" w1267 {
          tunnel: [w1274 w1282] -> w1270
          tunnel: w1271 -> [w1274 w1280]
          tunnel: w1269 -> [w1275 w1284]
          tunnel: [w1275 w1283] -> w1268
          tunnel: w1265 -> [_ w1278]
          tunnel: w1263 -> [_ w1276]
          frame False {
          }
          frame True {
            n577 = call "Logger_Create.vi"("Logger Queue"=w1278, "Output Directory"="Log File Directory", "HPS17K Refs"=w1276, "Error In"=w1280, "Log File Type"=enum16{"TDMS", "CSV"}."TDMS") -> ("reference out"=w1281:refnum<class "Logger.lvclass">, "Error Out"=w1282:errorcluster)  [unwired: 13 in]
            n578 = Bundle By Name(cluster=w1284, "Logger Ref"=w1281) -> (w1283:T13)
          }
        }
      }
      frame "Script: Launch Grapher" {
        n579 = Unbundle By Name(w1291) -> ("Graph Queue"=w1285:refnum<queue>, "HPS17K Refs"=w1287:refnum<class "HPS-17000.lvclass">[], "Grapher Ref"=w1289:refnum<class "Grapher.lvclass">)
        n580 = Equal?(x=w1289, y=refnum<class "Grapher.lvclass"> refnum) -> (x = y?=w1288:bool)
        n581 = case shown="True" w1288 {
          tunnel: [w1296 w1309] -> w1292
          tunnel: w1293 -> [w1296 w1310]
          tunnel: w1291 -> [w1297 w1312]
          tunnel: [w1297 w1311] -> w1290
          tunnel: w1287 -> [_ w1307]
          tunnel: w1285 -> [_ w1306]
          frame False {
          }
          frame True {
            w1305 = 50  # Update Rate (ms)
            n582 = control-ref of="XY Graph"() -> (w1303:refnum<vi>)
            n583 = control-ref of="Function"() -> (w1298:refnum<vi>)
            n584 = control-ref of="VOLTAGE"() -> (w1300:refnum<vi>)
            n585 = control-ref of="CURRENT"() -> (w1299:refnum<vi>)
            n586 = control-ref of="POWER"() -> (w1301:refnum<vi>)
            n587 = Bundle By Name(cluster=T20 {"XY Graph"=refnum, "Voltage"=refnum, "Current"=refnum, "Power"=refnum, "Function"=refnum} ("Indicator Refs"), "XY Graph"=w1303, "Voltage"=w1300, "Current"=w1299, "Power"=w1301, "Function"=w1298) -> (w1302:T20)
            n588 = call "Grapher_Create.vi"("Indicator Refs"=w1302, "Update Rate (ms)"=w1305, "Graph Queue"=w1306, "HPS17K Refs"=w1307, "Error In"=w1310) -> ("reference out"=w1308:refnum<class "Grapher.lvclass">, "Error Out"=w1309:errorcluster)  [unwired: 13 in]
            n589 = Bundle By Name(cluster=w1312, "Grapher Ref"=w1308) -> (w1311:T13)
          }
        }
      }
      frame "Script: Launch Test Server" {
        n590 = Unbundle By Name(w1316) -> ("Test Server Ref"=w1314:refnum<class "Script.lvclass">)
        n591 = Equal?(x=w1314, y=refnum<class "Script.lvclass"> refnum) -> (x = y?=w1315:bool)
        n592 = case shown="True" w1315 {
          tunnel: w1320 -> [w1324 w1335]
          tunnel: [w1324 w1337] -> w1319
          tunnel: [w1323 w1338] -> w1317
          tunnel: w1314 -> [w1323 _]
          frame False {
          }
          frame True {
            w1332 = "~/testserver.log" ("format string")
            w1333 = 1000  # Update Rate (ms)
            n593 = property on="HPS17K IP Addresses" class="Tree (strict)"() -> ("All Tags"=w1329:string[])  [unwired: 2 in, 2 out]
            n594 = local read "Cycler Selection"() -> (w1327:i16)
            n595 = In Range and Coerce(upper limit=i16 50, x=w1327, lower limit=i16 0) -> (coerced(x)=w1326:i16)  [unwired: 1 out]
            n596 = property on="Run Self Test" class="Bool (strict)"("DisabledEnum"=T14."Enabled" ("Disabled")) -> ()  [unwired: 2 in, 2 out]
            n597 = Index Array(array=w1329, index=w1326) -> (element=w1330:string)
            n598 = control-ref of="Test Server Listbox"() -> (w1336:refnum<vi>)
            n599 = Format Into String(format string="script -c ~/testserver.sh -f %s", w1332) -> (resulting string=w1334:string)  [unwired: 2 in, 1 out]
            n600 = call "Script_Create.vi"("Full Command"=w1334, "Script Name"="pess_testsuite_" ("format string"), "Log File"=w1332, "IP Address"=w1330, "Error In"=w1335, "Update Rate (ms)"=w1333, "Console Listbox"=w1336) -> ("reference out"=w1338:refnum<class "Script.lvclass">, "Error Out"=w1337:errorcluster)  [unwired: 11 in]
          }
        }
        n601 = Bundle By Name(cluster=w1316, "Test Server Ref"=w1317) -> (w1318:T13)
      }
      frame "Script: Volta Monitor" {
        n602 = property on="HPS17K IP Addresses" class="Tree (strict)"() -> ("All Tags"=w1349:string[])  [unwired: 2 in, 2 out]
        n603 = local read "Cycler Selection"() -> (w1347:i16)
        n604 = Format Into String(format string="%s: Launched Volta Monitor", w1341) -> (resulting string=w1343:string)  [unwired: 2 in, 1 out]
        n605 = local write "Status Message"(w1343) -> ()
        n606 = In Range and Coerce(upper limit=i16 50, x=w1347, lower limit=i16 0) -> (coerced(x)=w1346:i16)  [unwired: 1 out]
        n607 = Index Array(array=w1349, index=w1346) -> (element=w1345:string)
        n608 = Format Into String(format string="plink -l admin %s -batch -t \"/usr/local/natinst/bin/volta_monitor\"", w1345) -> (resulting string=w1352:string)  [unwired: 2 in, 1 out]
        n609 = call <vilib>:"System Exec.vi"("run minimized? (F)"=FALSE, "wait until completion? (T)"=FALSE, "error in (no error)"=w1355, "command line"=w1352) -> ("error out"=w1354:errorcluster)  [unwired: 4 in, 3 out]
      }
      frame "Script: FC Sys Inspect" {
        n610 = property on="HPS17K IP Addresses" class="Tree (strict)"() -> ("All Tags"=w1367:string[])  [unwired: 2 in, 2 out]
        n611 = local read "Cycler Selection"() -> (w1365:i16)
        n612 = Format Into String(format string="%s: Launched FC Sys Inspect", w1359) -> (resulting string=w1361:string)  [unwired: 2 in, 1 out]
        n613 = local write "Status Message"(w1361) -> ()
        n614 = In Range and Coerce(upper limit=i16 50, x=w1365, lower limit=i16 0) -> (coerced(x)=w1364:i16)  [unwired: 1 out]
        n615 = Index Array(array=w1367, index=w1364) -> (element=w1363:string)
        n616 = Format Into String(format string="plink -l admin %s -batch -t \"/usr/local/natinst/bin/fc_sys_inspect\"", w1363) -> (resulting string=w1373:string)  [unwired: 2 in, 1 out]
        n617 = call <vilib>:"System Exec.vi"("run minimized? (F)"=FALSE, "wait until completion? (T)"=FALSE, "error in (no error)"=w1369, "command line"=w1373) -> ("error out"=w1368:errorcluster)  [unwired: 4 in, 3 out]
      }
      frame "Script: Write Slew Rates" {
        n618 = Format Into String(format string="%s: Write Slew Rates", w1377) -> (resulting string=w1379:string)  [unwired: 2 in, 1 out]
        n619 = property on="HPS17K IP Addresses" class="Tree (strict)"() -> ("All Tags"=w1385:string[])  [unwired: 2 in, 2 out]
        n620 = local read "Cycler Selection"() -> (w1383:i16)
        n621 = local write "Status Message"(w1379) -> ()
        n622 = In Range and Coerce(upper limit=i16 50, x=w1383, lower limit=i16 0) -> (coerced(x)=w1382:i16)  [unwired: 1 out]
        n623 = Index Array(array=w1385, index=w1382) -> (element=w1381:string)
        n624 = Cluster To Array(cluster="Slew Rates") -> (array=w1386:sgl[])
        n625 = for {
          tunnel: w1391 -> [w1401]
          tunnel: [w1400] -> w1390
          tunnel: "plink -l admin %s -batch -t \"/usr/local/natinst/bin/mb_shm %s -w %f\"" ("format string") -> [w1399]
          tunnel: w1381 -> [w1398]
          tunnel: string[] ["RATE_LIM_SP_V_INC", "RATE_LIM_SP_V_DEC", "RATE_LIM_SP_I_INC", "RATE_LIM_SP_I_DEC", "RATE_LIM_SP_R_INC", "RATE_LIM_SP_R_DEC"] -> [w1396] mode=indexing
          tunnel: w1386 -> [w1395] mode=indexing
          workers-P: _ -> [_]
          n626 = Format Into String(format string=w1399, w1398, w1396, w1395) -> (resulting string=w1397:string)  [unwired: 2 in, 1 out]
          n627 = call <vilib>:"System Exec.vi"("run minimized? (F)"=TRUE, "wait until completion? (T)"=FALSE, "error in (no error)"=w1401, "command line"=w1397) -> ("error out"=w1400:errorcluster)  [unwired: 4 in, 3 out]
        }
      }
      frame "Script: Read Slew Rates" {
        n628 = property on="HPS17K IP Addresses" class="Tree (strict)"() -> ("All Tags"=w1412:string[])  [unwired: 2 in, 2 out]
        n629 = local read "Cycler Selection"() -> (w1410:i16)
        n630 = Format Into String(format string="%s: Read Slew Rates", w1404) -> (resulting string=w1406:string)  [unwired: 2 in, 1 out]
        n631 = In Range and Coerce(upper limit=i16 50, x=w1410, lower limit=i16 0) -> (coerced(x)=w1409:i16)  [unwired: 1 out]
        n632 = local write "Status Message"(w1406) -> ()
        n633 = Index Array(array=w1412, index=w1409) -> (element=w1408:string)
        n634 = for {
          tunnel: w1418 -> [w1434]
          tunnel: [w1428] -> w1417
          tunnel: "plink -l admin %s -batch -t \"/usr/local/natinst/bin/mb_shm %s" ("format string") -> [w1433]
          tunnel: w1408 -> [w1432]
          tunnel: string[] ["RATE_LIM_SP_V_INC", "RATE_LIM_SP_V_DEC", "RATE_LIM_SP_I_INC", "RATE_LIM_SP_I_DEC", "RATE_LIM_SP_R_INC", "RATE_LIM_SP_R_DEC"] -> [w1430] mode=indexing
          workers-P: _ -> [_]
          tunnel: [w1426] -> w1414 mode=indexing
          n635 = Format Into String(format string=w1433, w1432, w1430) -> (resulting string=w1431:string)  [unwired: 2 in, 1 out]
          n636 = call <vilib>:"System Exec.vi"("run minimized? (F)"=TRUE, "wait until completion? (T)"=TRUE, "error in (no error)"=w1434, "command line"=w1431) -> ("error out"=w1428:errorcluster, "standard output"=w1425:string)  [unwired: 4 in, 2 out]
          n637 = Search/Split String(string=w1425, search string/char (-)=":") -> (match + rest of string=w1423:string)  [unwired: 1 in, 2 out]
          n638 = String Subset(string=w1423, offset (0)=1) -> (substring=w1422:string)  [unwired: 1 in]
          n639 = call <vilib>:"Trim Whitespace.vi"("string"=w1422) -> ("trimmed string"=w1427:string)  [unwired: 1 in]
          n640 = Fract/Exp String To Number(string=w1427) -> (number=w1426:dbl)  [unwired: 3 in, 1 out]
        }
        n641 = Array To Cluster(array=w1414) -> (cluster=w1413:T28)
        n642 = local write "Slew Rates"(w1413) -> ()
      }
      frame "Script: Read Setpoint Limits" {
        n643 = property on="HPS17K IP Addresses" class="Tree (strict)"() -> ("All Tags"=w1445:string[])  [unwired: 2 in, 2 out]
        n644 = local read "Cycler Selection"() -> (w1443:i16)
        n645 = Format Into String(format string="%s: Read Setpoint Limits", w1437) -> (resulting string=w1439:string)  [unwired: 2 in, 1 out]
        n646 = local write "Status Message"(w1439) -> ()
        n647 = In Range and Coerce(upper limit=i16 50, x=w1443, lower limit=i16 0) -> (coerced(x)=w1442:i16)  [unwired: 1 out]
        n648 = Index Array(array=w1445, index=w1442) -> (element=w1441:string)
        n649 = for {
          tunnel: w1451 -> [w1467]
          tunnel: [w1461] -> w1450
          tunnel: "plink -l admin %s -batch -t \"/usr/local/natinst/bin/mb_shm %s" ("format string") -> [w1466]
          tunnel: w1441 -> [w1465]
          tunnel: string[] ["lim_i_pos", "lim_i_neg", "lim_v_high", "lim_v_low", "lim_p_pos", "lim_p_neg"] -> [w1463] mode=indexing
          workers-P: _ -> [_]
          tunnel: [w1459] -> w1447 mode=indexing
          n650 = Format Into String(format string=w1466, w1465, w1463) -> (resulting string=w1464:string)  [unwired: 2 in, 1 out]
          n651 = call <vilib>:"System Exec.vi"("run minimized? (F)"=TRUE, "wait until completion? (T)"=TRUE, "error in (no error)"=w1467, "command line"=w1464) -> ("error out"=w1461:errorcluster, "standard output"=w1458:string)  [unwired: 4 in, 2 out]
          n652 = Search/Split String(string=w1458, search string/char (-)=":") -> (match + rest of string=w1456:string)  [unwired: 1 in, 2 out]
          n653 = String Subset(string=w1456, offset (0)=1) -> (substring=w1455:string)  [unwired: 1 in]
          n654 = call <vilib>:"Trim Whitespace.vi"("string"=w1455) -> ("trimmed string"=w1460:string)  [unwired: 1 in]
          n655 = Fract/Exp String To Number(string=w1460) -> (number=w1459:dbl)  [unwired: 3 in, 1 out]
        }
        n656 = Array To Cluster(array=w1447) -> (cluster=w1446:T28)
        n657 = local write "Limits"(w1446) -> ()
      }
      frame "Script: Read Setpoints" {
        n658 = property on="HPS17K IP Addresses" class="Tree (strict)"() -> ("All Tags"=w1478:string[])  [unwired: 2 in, 2 out]
        n659 = local read "Cycler Selection"() -> (w1476:i16)
        n660 = Format Into String(format string="%s: Read Setpoints", w1470) -> (resulting string=w1472:string)  [unwired: 2 in, 1 out]
        n661 = local write "Status Message"(w1472) -> ()
        n662 = In Range and Coerce(upper limit=i16 50, x=w1476, lower limit=i16 0) -> (coerced(x)=w1475:i16)  [unwired: 1 out]
        n663 = Index Array(array=w1478, index=w1475) -> (element=w1474:string)
        n664 = for {
          tunnel: w1484 -> [w1500]
          tunnel: [w1494] -> w1483
          tunnel: "plink -l admin %s -batch -t \"/usr/local/natinst/bin/mb_shm %s" ("format string") -> [w1499]
          tunnel: w1474 -> [w1498]
          tunnel: string[] ["sp_v", "sp_i", "lim_p_neg", "lim_p_pos", "sp_r"] -> [w1496] mode=indexing
          workers-P: _ -> [_]
          tunnel: [w1492] -> w1480 mode=indexing
          n665 = Format Into String(format string=w1499, w1498, w1496) -> (resulting string=w1497:string)  [unwired: 2 in, 1 out]
          n666 = call <vilib>:"System Exec.vi"("run minimized? (F)"=TRUE, "wait until completion? (T)"=TRUE, "error in (no error)"=w1500, "command line"=w1497) -> ("error out"=w1494:errorcluster, "standard output"=w1491:string)  [unwired: 4 in, 2 out]
          n667 = Search/Split String(string=w1491, search string/char (-)=":") -> (match + rest of string=w1489:string)  [unwired: 1 in, 2 out]
          n668 = String Subset(string=w1489, offset (0)=1) -> (substring=w1488:string)  [unwired: 1 in]
          n669 = call <vilib>:"Trim Whitespace.vi"("string"=w1488) -> ("trimmed string"=w1493:string)  [unwired: 1 in]
          n670 = Fract/Exp String To Number(string=w1493) -> (number=w1492:dbl)  [unwired: 3 in, 1 out]
        }
        n671 = Array To Cluster(array=w1480) -> (cluster=w1479:T29)
        n672 = local write "Setpoints"(w1479) -> ()
      }
      frame "Script: Read Thermal Limits" {
        n673 = property on="HPS17K IP Addresses" class="Tree (strict)"() -> ("All Tags"=w1511:string[])  [unwired: 2 in, 2 out]
        n674 = local read "Cycler Selection"() -> (w1509:i16)
        n675 = Format Into String(format string="%s: Read Thermal Limits", w1503) -> (resulting string=w1505:string)  [unwired: 2 in, 1 out]
        n676 = local write "Status Message"(w1505) -> ()
        n677 = In Range and Coerce(upper limit=i16 50, x=w1509, lower limit=i16 0) -> (coerced(x)=w1508:i16)  [unwired: 1 out]
        n678 = Index Array(array=w1511, index=w1508) -> (element=w1507:string)
        n679 = for {
          tunnel: w1516 -> [w1532]
          tunnel: [w1527] -> w1515
          tunnel: "plink -l admin %s -batch -t \"/usr/local/natinst/bin/mb_shm %s" ("format string") -> [w1531]
          tunnel: w1507 -> [w1530]
          tunnel: string[] ["LIM_TEMP_AIR", "LIM_TEMP_TR", "T_AIR_LOW", "T_AIR_HIGH", "T_TR_LOW", "T_TR_HIGH"] -> [w1522] mode=indexing
          workers-P: _ -> [_]
          tunnel: [w1520] -> w1512 mode=indexing
          n680 = Format Into String(format string=w1531, w1530, w1522) -> (resulting string=w1529:string)  [unwired: 2 in, 1 out]
          n681 = call <vilib>:"System Exec.vi"("run minimized? (F)"=TRUE, "wait until completion? (T)"=TRUE, "error in (no error)"=w1532, "command line"=w1529) -> ("error out"=w1527:errorcluster, "standard output"=w1526:string)  [unwired: 4 in, 2 out]
          n682 = Search/Split String(string=w1526, search string/char (-)=":") -> (match + rest of string=w1524:string)  [unwired: 1 in, 2 out]
          n683 = String Subset(string=w1524, offset (0)=1) -> (substring=w1523:string)  [unwired: 1 in]
          n684 = call <vilib>:"Trim Whitespace.vi"("string"=w1523) -> ("trimmed string"=w1521:string)  [unwired: 1 in]
          n685 = Build Array(w1522, w1521) -> (w1520:string[])
        }
        n686 = property on="Thermal Limits" class="MCListbox (strict)"("ItemNames"=w1512) -> ()  [unwired: 2 in, 2 out]
      }
      frame "Script: Read Temperatures" {
        n687 = property on="HPS17K IP Addresses" class="Tree (strict)"() -> ("All Tags"=w1543:string[])  [unwired: 2 in, 2 out]
        n688 = local read "Cycler Selection"() -> (w1541:i16)
        n689 = Format Into String(format string="%s: Read Temperatures", w1535) -> (resulting string=w1537:string)  [unwired: 2 in, 1 out]
        n690 = local write "Status Message"(w1537) -> ()
        n691 = In Range and Coerce(upper limit=i16 50, x=w1541, lower limit=i16 0) -> (coerced(x)=w1540:i16)  [unwired: 1 out]
        n692 = Index Array(array=w1543, index=w1540) -> (element=w1539:string)
        n693 = for {
          tunnel: w1548 -> [w1564]
          tunnel: [w1559] -> w1547
          tunnel: "plink -l admin %s -batch -t \"/usr/local/natinst/bin/mb_shm %s" ("format string") -> [w1563]
          tunnel: w1539 -> [w1562]
          tunnel: string[] ["bo_rear", "bo_front", "cc_rear", "cc_front", "trafo1/0", "trafo1/1", "trafo1/2", "trafo2/0", "trafo2/1", "trafo2/2"] -> [w1554] mode=indexing
          workers-P: _ -> [_]
          tunnel: [w1552] -> w1544 mode=indexing
          n694 = Format Into String(format string=w1563, w1562, w1554) -> (resulting string=w1561:string)  [unwired: 2 in, 1 out]
          n695 = call <vilib>:"System Exec.vi"("run minimized? (F)"=TRUE, "wait until completion? (T)"=TRUE, "error in (no error)"=w1564, "command line"=w1561) -> ("error out"=w1559:errorcluster, "standard output"=w1558:string)  [unwired: 4 in, 2 out]
          n696 = Search/Split String(string=w1558, search string/char (-)=":") -> (match + rest of string=w1556:string)  [unwired: 1 in, 2 out]
          n697 = String Subset(string=w1556, offset (0)=1) -> (substring=w1555:string)  [unwired: 1 in]
          n698 = call <vilib>:"Trim Whitespace.vi"("string"=w1555) -> ("trimmed string"=w1553:string)  [unwired: 1 in]
          n699 = Build Array(w1554, w1553) -> (w1552:string[])
        }
        n700 = property on="Temperatures" class="MCListbox (strict)"("ItemNames"=w1544) -> ()  [unwired: 2 in, 2 out]
      }
      frame "Script: Read Hardware Limits" {
        n701 = local read "Cycler Selection"() -> (w1572:i16)
        n702 = property on="HPS17K IP Addresses" class="Tree (strict)"() -> ("All Tags"=w1574:string[])  [unwired: 2 in, 2 out]
        n703 = In Range and Coerce(upper limit=i16 50, x=w1572, lower limit=i16 0) -> (coerced(x)=w1571:i16)  [unwired: 1 out]
        n704 = Format Into String(format string="%s: Read Hardware Limits", w1567) -> (resulting string=w1569:string)  [unwired: 2 in, 1 out]
        n705 = Index Array(array=w1574, index=w1571) -> (element=w1575:string)
        n706 = local write "Status Message"(w1569) -> ()
        n707 = for {
          tunnel: w1580 -> [w1596]
          tunnel: [w1591] -> w1579
          tunnel: "plink -l admin %s -batch -t \"/usr/local/natinst/bin/mb_shm %s" ("format string") -> [w1595]
          tunnel: w1575 -> [w1594]
          tunnel: string[] ["LIM_HW_I_PARALLEL_POS", "LIM_HW_I_PARALLEL_NEG", "LIM_HW_I_SERIES_POS", "LIM_HW_I_SERIES_NEG", "LIM_HW_V_PARALLEL_HIGH", "LIM_HW_V_PARALLEL_LOW", "LIM_HW_V_SERIES_HIGH", "LIM_HW_V_SERIES_LOW", "LIM_HW_P_POS", "LIM_HW_P_NEG", "LIM_HW_R_HIGH", "LIM_HW_R_LOW"] -> [w1586] mode=indexing
          workers-P: _ -> [_]
          tunnel: [w1584] -> w1576 mode=indexing
          n708 = Format Into String(format string=w1595, w1594, w1586) -> (resulting string=w1593:string)  [unwired: 2 in, 1 out]
          n709 = call <vilib>:"System Exec.vi"("run minimized? (F)"=TRUE, "wait until completion? (T)"=TRUE, "error in (no error)"=w1596, "command line"=w1593) -> ("error out"=w1591:errorcluster, "standard output"=w1590:string)  [unwired: 4 in, 2 out]
          n710 = Search/Split String(string=w1590, search string/char (-)=":") -> (match + rest of string=w1588:string)  [unwired: 1 in, 2 out]
          n711 = String Subset(string=w1588, offset (0)=1) -> (substring=w1587:string)  [unwired: 1 in]
          n712 = call <vilib>:"Trim Whitespace.vi"("string"=w1587) -> ("trimmed string"=w1585:string)  [unwired: 1 in]
          n713 = Build Array(w1586, w1585) -> (w1584:string[])
        }
        n714 = property on="Hardware Limits" class="MCListbox (strict)"("ItemNames"=w1576) -> ()  [unwired: 2 in, 2 out]
      }
      frame "Script: Stop Test Server" {
        n715 = Unbundle By Name(w1603) -> ("Test Server Ref"=w1601:refnum<class "Script.lvclass">)
        n716 = Equal?(x=w1601, y=refnum<class "Script.lvclass"> refnum) -> (x = y?=w1602:bool)
        n717 = case shown="False" w1602 {
          tunnel: w1606 -> [w1610 w1615]
          tunnel: [w1609 w1615] -> w1605
          tunnel: w1601 -> [w1611 w1614]
          tunnel: [refnum<class "Script.lvclass"> refnum ("Test Server Ref") w1614] -> w1600
          frame False {
            n718 = call-dynamic "Destroy.vi"("reference in"=w1611, "Error In"=w1610) -> ("Error Out"=w1609:errorcluster)  [unwired: 16 in, 1 out]
            n719 = property on="Run Self Test" class="Bool (strict)"("DisabledEnum"=T14."Disabled and Grayed Out" ("Disabled")) -> ()  [unwired: 2 in, 2 out]
          }
          frame True {
          }
        }
        n720 = Bundle By Name(cluster=w1603, "Test Server Ref"=w1600) -> (w1604:T13)
      }
      frame "Script: Start Self Test" {
        n721 = Unbundle By Name(w1623) -> ("Self Test Ref"=w1618:refnum<class "Script.lvclass">, "Self Test Completed"=w1620:refnum<user-event>)
        n722 = Equal?(x=refnum<class "Script.lvclass"> refnum ("y"), y=w1618) -> (x = y?=w1622:bool)
        n723 = case shown="True" w1622 {
          tunnel: w1627 -> [w1631 w1645]
          tunnel: [w1631 w1651] -> w1626
          tunnel: [w1630 w1652] -> w1624
          tunnel: w1618 -> [w1630 _]
          tunnel: w1620 -> [w1629 _]
          tunnel: [w1629 w1637] -> w1617
          tunnel: "Voltage Reformation" -> [_ w1635]
          frame False {
          }
          frame True {
            w1646 = FALSE  # Script Complete
            w1636 = "~/selftest.log" ("format string")
            n724 = Create User Event(user event datatype=w1646, error in=w1645) -> (user event=w1637:refnum<user-event>, error out=w1644:errorcluster)
            n725 = Select(t="~/selftest-reform.sh" ("format string"), s=w1635, f="~/selftest.sh" ("format string")) -> (s? t:f=w1633:string)
            n726 = local read "Cycler Selection"() -> (w1641:i16)
            n727 = property on="HPS17K IP Addresses" class="Tree (strict)"() -> ("All Tags"=w1643:string[])  [unwired: 2 in, 2 out]
            n728 = Format Into String(format string="script -c %s -f %s", w1633, w1636) -> (resulting string=w1648:string)  [unwired: 2 in, 1 out]
            n729 = control-ref of="Self Test Log"() -> (w1650:refnum<vi>)
            n730 = In Range and Coerce(upper limit=i16 50, x=w1641, lower limit=i16 0) -> (coerced(x)=w1640:i16)  [unwired: 1 out]
            n731 = Index Array(array=w1643, index=w1640) -> (element=w1639:string)
            n732 = call "Script_Create.vi"("Full Command"=w1648, "Script Name"="pess_selftest" ("format string"), "Log File"=w1636, "IP Address"=w1639, "Error In"=w1644, "Update Rate (ms)"=1000, "Console Listbox"=w1650, "Script Complete Event"=w1637) -> ("reference out"=w1652:refnum<class "Script.lvclass">, "Error Out"=w1651:errorcluster)  [unwired: 10 in]
          }
        }
        n733 = Bundle By Name(cluster=w1623, "Self Test Completed"=w1617, "Self Test Ref"=w1624) -> (w1625:T13)
      }
      frame "Script: Stop Self Test" {
        n734 = Unbundle By Name(w1659) -> ("Self Test Ref"=w1657:refnum<class "Script.lvclass">)
        n735 = Equal?(x=w1657, y=refnum<class "Script.lvclass"> refnum) -> (x = y?=w1658:bool)
        n736 = case shown="False" w1658 {
          tunnel: w1662 -> [w1665 w1669]
          tunnel: [w1666 w1669] -> w1661
          tunnel: w1657 -> [w1664 w1668]
          tunnel: [refnum<class "Script.lvclass"> refnum ("Self Test Ref") w1668] -> w1655
          frame False {
            n737 = call-dynamic "Destroy.vi"("reference in"=w1664, "Error In"=w1665) -> ("Error Out"=w1666:errorcluster)  [unwired: 16 in, 1 out]
          }
          frame True {
          }
        }
        n738 = Bundle By Name(cluster=w1659, "Self Test Ref"=w1655) -> (w1660:T13)
      }
      frame "Script: Stop Streamer" {
        n739 = Unbundle By Name(w1674) -> ("Streamer Ref"=w1672:refnum<class "Streamer.lvclass">)
        n740 = Equal?(x=w1672, y=refnum<class "Streamer.lvclass"> refnum) -> (x = y?=w1673:bool)
        n741 = case shown="False" w1673 {
          tunnel: w1677 -> [w1681 w1685]
          tunnel: [w1680 w1685] -> w1676
          tunnel: w1672 -> [w1682 w1684]
          tunnel: [refnum<class "Streamer.lvclass"> refnum ("Stream Ref") w1684] -> w1671
          frame False {
            n742 = call-dynamic "Destroy.vi"("reference in"=w1682, "Error In"=w1681) -> ("Error Out"=w1680:errorcluster)  [unwired: 16 in, 1 out]
          }
          frame True {
          }
        }
        n743 = Bundle By Name(cluster=w1674, "Streamer Ref"=w1671) -> (w1675:T13)
      }
      frame "Script: Stop Logger" {
        n744 = Unbundle By Name(w1691) -> ("Logger Ref"=w1689:refnum<class "Logger.lvclass">)
        n745 = Equal?(x=w1689, y=refnum<class "Logger.lvclass"> refnum) -> (x = y?=w1690:bool)
        n746 = case shown="False" w1690 {
          tunnel: w1694 -> [w1705 w1714]
          tunnel: [w1699 w1714] -> w1693
          tunnel: w1689 -> [w1702 w1713]
          tunnel: [refnum<class "Logger.lvclass"> refnum ("Logger Ref") w1713] -> w1688
          tunnel: w1686 -> [w1697 _]
          frame False {
            w1701 = -1  # timeout in ms (-1)
            n747 = call "Close Log.vi"("reference in"=w1702, "timeout in ms (-1)"=w1701, "Error In"=w1705) -> ("reference out"=w1703:refnum<class "Logger.lvclass">, "log file path"=w1698:path, "Error Out"=w1704:errorcluster)  [unwired: 14 in]
            n748 = call-dynamic "Destroy.vi"("reference in"=w1703, "Error In"=w1704) -> ("Error Out"=w1700:errorcluster)  [unwired: 16 in, 1 out]
            n749 = flat-sequence {
              tunnel: w1700 -> [w1712]
              tunnel: [w1711] -> w1699
              tunnel: w1698 -> [w1708]
              tunnel: w1697 -> [w1707]
              frame #0 {
                n750 = Format Into String(format string="%s: Log File Saved to %s", w1707, w1708) -> (resulting string=w1709:string)  [unwired: 2 in, 1 out]
                n751 = property on="Status Message" class="Str"(error in=w1712, "Value"=w1709) -> (error out=w1711:errorcluster)  [unwired: 1 in, 1 out]
              }
            }
          }
          frame True {
          }
        }
        n752 = Bundle By Name(cluster=w1691, "Logger Ref"=w1688) -> (w1692:T13)
      }
      frame "Script: Stop Grapher" {
        n753 = Unbundle By Name(w1719) -> ("Grapher Ref"=w1717:refnum<class "Grapher.lvclass">)
        n754 = Equal?(x=w1717, y=refnum<class "Grapher.lvclass"> refnum) -> (x = y?=w1718:bool)
        n755 = case shown="False" w1718 {
          tunnel: w1722 -> [w1728 w1730]
          tunnel: [w1727 w1730] -> w1721
          tunnel: w1717 -> [w1726 w1729]
          tunnel: [refnum<class "Grapher.lvclass"> refnum ("y") w1729] -> w1716
          frame False {
            n756 = call-dynamic "Destroy.vi"("reference in"=w1726, "Error In"=w1728) -> ("Error Out"=w1727:errorcluster)  [unwired: 16 in, 1 out]
          }
          frame True {
          }
        }
        n757 = Bundle By Name(cluster=w1719, "Grapher Ref"=w1716) -> (w1720:T13)
      }
      frame "---------- Events ----------" {
        # "Do not put any code in this frame.\n(It is a separator no-op. You can make a copy of this frame to create a new UI frame)"
      }
      frame "Events: Register" {
        n758 = Unbundle By Name(w1738) -> ("HPS17K Events"=w1737:T12, "Self Test Completed"=w1735:refnum<user-event>)
        n759 = register-events(error in=w1736, w1737, w1735) -> (reference out=w1740:refnum<event-registration>, error out=w1739:errorcluster)  [unwired: 1 in]
      }
      frame "Events: Unregister" {
        n760 = Unregister For Events(event registration refnum=w1744, error in=w1743) -> (error out=w1742:errorcluster)
      }
      frame "---------- UI ----------" {
        # "Do not put any code in this frame.\n(It is a separator no-op. You can make a copy of this frame to create a new UI frame)"
      }
      frame "UI: Initialize" {
        w1762 = i16 -1 items=["ALL"=-1, "10.204.213.142"=0] ("Cycler Selection")
        w1765 = FALSE ("HPS Connect")
        w1771 = 0.0 ("POWER")
        w1772 = "" ("Error Message")
        w1767 = string[] [] ("Item Names")
        w1754 = T14."Disabled and Grayed Out" ("Disabled")
        # "Initialize the User Interface, here.\n(this is called automatically, by the Macro: Initialize)"
        n761 = property on="Run Self Test" class="Bool (strict)"("DisabledEnum"=w1754) -> ()  [unwired: 2 in, 2 out]
        n762 = property on="Apply Setpoints" class="Bool"("DisabledEnum"=w1754) -> ()  [unwired: 2 in, 2 out]
        n763 = property on="Energize" class="Bool (strict)"("DisabledEnum"=w1754) -> ()  [unwired: 2 in, 2 out]
        n764 = property on="Output" class="Bool (strict)"("DisabledEnum"=w1754) -> ()  [unwired: 2 in, 2 out]
        n765 = property on="Get Device Properties" class="Bool"("DisabledEnum"=w1754) -> ()  [unwired: 2 in, 2 out]
        n766 = property on="Get XC Report" class="Bool"("DisabledEnum"=w1754) -> ()  [unwired: 2 in, 2 out]
        n767 = property on="FC Sys Inspect" class="Bool"("DisabledEnum"=w1754) -> ()  [unwired: 2 in, 2 out]
        n768 = property on="Volta Monitor" class="Bool"("DisabledEnum"=w1754) -> ()  [unwired: 2 in, 2 out]
        n769 = property on="HPS Reserve" class="Bool (strict)"("DisabledEnum"=w1754) -> ()  [unwired: 2 in, 2 out]
        n770 = property on="Apply Mode & Range" class="Bool"("DisabledEnum"=w1754) -> ()  [unwired: 2 in, 2 out]
        n771 = property on="Apply Limits" class="Bool"("DisabledEnum"=w1754) -> ()  [unwired: 2 in, 2 out]
        n772 = property on="HPS Clear" class="Bool"("DisabledEnum"=w1754) -> ()  [unwired: 2 in, 2 out]
        n773 = property on="Launch Test Server" class="Bool (strict)"("DisabledEnum"=w1754) -> ()  [unwired: 2 in, 2 out]
        n774 = property on="High Speed" class="Bool (strict)"("DisabledEnum"=w1754) -> ()  [unwired: 2 in, 2 out]
        n775 = property on="Start Profile" class="Bool (strict)"("DisabledEnum"=w1754) -> ()  [unwired: 2 in, 2 out]
        n776 = property on="Apply Slew Rates" class="Bool"("DisabledEnum"=w1754) -> ()  [unwired: 2 in, 2 out]
        n777 = property on="HPS Connect" class="Bool (strict)"("DisabledEnum"=w1754) -> ()  [unwired: 2 in, 2 out]
        n778 = local read "Log File Directory"() -> (w1760:path)
        n779 = Empty String/Path?(string/path=w1760) -> (empty?=w1759:bool)
        n780 = property on="Cycler Selection" class="Ring (strict)"("StringsAndValues[]"=T21 [{"String"="ALL", "Value"=-1}] ("Strings And Values []"), "Value"=w1762) -> ()  [unwired: 2 in, 2 out]
        n781 = Select(t=T14."Disabled and Grayed Out" ("Disabled"), s=w1759, f=T14."Enabled" ("Disabled")) -> (s? t:f=w1757:T14)
        n782 = property class="VI"("Front Panel.Title"="HPS17K Panel" ("Front Panel Window:Title")) -> ()  [unwired: 2 in, 2 out]
        n783 = call <userlib>:"Fit VI window to Largest Dec__ogtk.vi"("error in (no error)"=w1774) -> ("error out"=w1773:errorcluster)  [unwired: 5 in, 1 out]
        n784 = property on="Start Logging" class="Bool (strict)"("DisabledEnum"=w1757) -> ()  [unwired: 2 in, 2 out]
        n785 = invoke on="HPS17K IP Addresses" class="Tree (strict)" method="Edit Tree Items.Delete"() -> ()  [unwired: 5 in, 5 out]
        n786 = invoke on="Device Search" class="Tree (strict)" method="Edit Tree Items.Delete"() -> ()  [unwired: 5 in, 5 out]
        n787 = property on="Self Test Log" class="LstBox (strict)"("Item Names"=w1767) -> ()  [unwired: 2 in, 2 out]
        n788 = property on="Event Log" class="MCListbox (strict)"("ItemNames"=string[][] [] ("Item Names")) -> ()  [unwired: 2 in, 2 out]
        n789 = property on="Test Server Log" class="LstBox (strict)"("Item Names"=w1767) -> ()  [unwired: 2 in, 2 out]
        n790 = property on="Test Server Log" class="LstBox (strict)"("Top Row"=0) -> ()  [unwired: 2 in, 2 out]
        n791 = property on="Self Test Log" class="LstBox (strict)"("Top Row"=0) -> ()  [unwired: 2 in, 2 out]
        n792 = property on="Fault Message" class="Str"("Value"=w1772) -> ()  [unwired: 2 in, 2 out]
        n793 = property on="Status Message" class="Str"("Value"=w1772) -> ()  [unwired: 2 in, 2 out]
        n794 = local write "device properties"(T9 {"name"="", "model"="", "vendor"="", "serial_number"=""} ("device properties")) -> ()
        n795 = local write "CURRENT"(w1771) -> ()
        n796 = local write "VOLTAGE"(w1771) -> ()
        n797 = local write "POWER"(w1771) -> ()
        n798 = property on="EMO Indicator" class="Ring (strict)"("Value"=u16 0 ("EMO Indicator")) -> ()  [unwired: 2 in, 2 out]
        n799 = local write "HPS Connect"(w1765) -> ()
        n800 = local write "HPS Reserve"(w1765) -> ()
        n801 = local write "Energize"(w1765) -> ()
        n802 = local write "Output"(w1765) -> ()
        n803 = local write "Run Self Test"(w1765) -> ()
        n804 = local write "Launch Test Server"(w1765) -> ()
        n805 = local write "Main Tab Control"(T2."CONFIG" ("Main Tab Control")) -> ()
        n806 = local write "Setpoint Stream"(w1765) -> ()
        n807 = local write "Measurement Stream"(w1765) -> ()
        n808 = local write "XY Graph"(T3 [] ("appended array")) -> ()
        n809 = local write "Start Profile"(w1765) -> ()
        n810 = local write "CSV Profile"(waveform(sgl)[] [] ("CSV Profile")) -> ()
        n811 = local write item#-1(waveform(dbl)[] [] ("EIS Profile")) -> ()
      }
      frame "UI: Uninitialize" {
        # "Cleanup the User Interface, here.\n(this is called automatically, by the Macro: Exit)"
      }
      frame "UI: Self Test Start" {
        w1783 = T14."Disabled and Grayed Out" ("Disabled")
        n812 = local write "Run Self Test"(TRUE ("Run Self Test")) -> ()
        n813 = property on="Apply Mode & Range" class="Bool"("DisabledEnum"=w1783) -> ()  [unwired: 2 in, 2 out]
        n814 = property on="Apply Limits" class="Bool"("DisabledEnum"=w1783) -> ()  [unwired: 2 in, 2 out]
        n815 = property on="Apply Setpoints" class="Bool"("DisabledEnum"=w1783) -> ()  [unwired: 2 in, 2 out]
        n816 = property on="Apply Slew Rates" class="Bool"("DisabledEnum"=w1783) -> ()  [unwired: 2 in, 2 out]
        n817 = property on="Energize" class="Bool (strict)"("DisabledEnum"=w1783) -> ()  [unwired: 2 in, 2 out]
        n818 = property on="Output" class="Bool (strict)"("DisabledEnum"=w1783) -> ()  [unwired: 2 in, 2 out]
      }
      frame "UI: Self Test Stop" {
        w1790 = T14."Enabled" ("Disabled")
        n819 = local write "Run Self Test"(FALSE ("Run Self Test")) -> ()
        n820 = property on="Apply Mode & Range" class="Bool"("DisabledEnum"=w1790) -> ()  [unwired: 2 in, 2 out]
        n821 = property on="Apply Limits" class="Bool"("DisabledEnum"=w1790) -> ()  [unwired: 2 in, 2 out]
        n822 = property on="Apply Setpoints" class="Bool"("DisabledEnum"=w1790) -> ()  [unwired: 2 in, 2 out]
        n823 = property on="Apply Slew Rates" class="Bool"("DisabledEnum"=w1790) -> ()  [unwired: 2 in, 2 out]
        n824 = property on="Energize" class="Bool (strict)"("DisabledEnum"=w1790) -> ()  [unwired: 2 in, 2 out]
        n825 = property on="Output" class="Bool (strict)"("DisabledEnum"=w1790) -> ()  [unwired: 2 in, 2 out]
      }
      frame "UI: Add HPS17K" {
        n826 = call "Add HPS17K"() -> ("IP Address"=w1799:string, "Add"=w1796:bool)  [unwired: 17 in, 1 out]
        n827 = property on="HPS17K IP Addresses" class="Tree (strict)"() -> ("All Tags"=w1794:string[])  [unwired: 2 in, 2 out]
        n828 = Search 1D Array(1D array=w1794, element=w1799) -> (index of element=w1798:i32)  [unwired: 1 in]
        n829 = Less Than 0?(x=w1798) -> (x < 0?=w1797:bool)
        n830 = And(x=w1796, y=w1797) -> (x .and. y?=w1795:bool)
        n831 = case shown="True" w1795 {
          tunnel: w1799 -> [_ w1804]
          frame False {
          }
          frame True {
            n832 = String To IP(1:w1804) -> (0:w1805:u32)
            n833 = case shown="Default" w1805 {
              tunnel: w1804 -> [_ w1811]
              frame 0, 181174352 {
                # "0 = invalid\n\n181174352 = empty (localhost?)"
              }
              frame Default {
                n834 = property on="Cycler Selection" class="Ring (strict)"() -> ("StringsAndValues[]"=w1809:T21)  [unwired: 2 in, 2 out]
                n835 = Array Size(array=w1809) -> (size(s)=w1808:i32)
                n836 = invoke on="HPS17K IP Addresses" class="Tree (strict)" method="Edit Tree Items.Add Item"("Left Cell"=w1811, "Child Tag"=w1811) -> ()  [unwired: 7 in, 9 out]
                n837 = Decrement(x=w1808) -> (x-1=w1807:i32)
                n838 = Bundle By Name(cluster=cluster{"String":string, "Value":i16} {"String"="", "Value"=0} ("new element/subarray"), "String"=w1811, "Value"=w1807) -> (w1810:cluster{"String":string, "Value":i16})
                n839 = property on="HPS Connect" class="Bool (strict)"("DisabledEnum"=T14."Enabled" ("Disabled")) -> ()  [unwired: 2 in, 2 out]
                n840 = Insert Into Array(array=w1809, new element=w1810) -> (w1813:T21)  [unwired: 1 in]
                n841 = property on="Cycler Selection" class="Ring (strict)"("StringsAndValues[]"=w1813) -> ()  [unwired: 2 in, 2 out]
              }
            }
          }
        }
      }
      frame "UI: Remove HPS17K" {
        w1814 = i16 -1 items=["ALL"=-1] ("Cycler Selection")
        n842 = local read "HPS17K IP Addresses"() -> (w1822:string[])
        n843 = property on="Cycler Selection" class="Ring (strict)"() -> ("StringsAndValues[]"=w1823:T21)  [unwired: 2 in, 2 out]
        n844 = for {
          tunnel: w1822 -> [w1833] mode=indexing
          n845 = invoke on="HPS17K IP Addresses" class="Tree (strict)" method="Edit Tree Items.Delete"("tag"=w1833) -> ()  [unwired: 4 in, 5 out]
        }
        n846 = for {
          tunnel: w1823 -> [w1829] mode=indexing
          tunnel: [w1829] -> w1821 mode=indexing if=w1830
          tunnel: w1822 -> [w1832]
          n847 = Unbundle By Name(w1829) -> ("String"=w1828:string)
          n848 = Search 1D Array(1D array=w1832, element=w1828) -> (index of element=w1831:i32)  [unwired: 1 in]
          n849 = Less Than 0?(x=w1831) -> (x < 0?=w1830:bool)
        }
        n850 = property on="Cycler Selection" class="Ring (strict)"("StringsAndValues[]"=w1821, "Value"=w1814) -> ()  [unwired: 2 in, 2 out]
        n851 = Array Size(array=w1821) -> (size(s)=w1820:i32)
        n852 = Greater?(x=w1820, y=1) -> (0:w1819:bool)
        n853 = Select(t=T14."Enabled" ("Disabled"), s=w1819, f=T14."Disabled and Grayed Out" ("Disabled")) -> (s? t:f=w1818:T14)
        n854 = property on="HPS Connect" class="Bool (strict)"("DisabledEnum"=w1818) -> ()  [unwired: 2 in, 2 out]
      }
      frame "UI: Reservation Complete" {
        n855 = Format Into String(format string="%s: Reservation Successful", w1834) -> (resulting string=w1836:string)  [unwired: 2 in, 1 out]
        n856 = local write "Status Message"(w1836) -> ()
      }
      frame "UI: Reservation Failed" {
        n857 = Format Into String(format string="%s: Reservation Failed", w1841) -> (resulting string=w1843:string)  [unwired: 2 in, 1 out]
        n858 = local write "Status Message"(w1843) -> ()
      }
      frame "UI: Connection Complete" {
        n859 = Format Into String(format string="%s: Connection Successful", w1848) -> (resulting string=w1850:string)  [unwired: 2 in, 1 out]
        n860 = local write "Status Message"(w1850) -> ()
      }
      frame "UI: Connection Failed" {
        n861 = Format Into String(format string="%s: Connection Failed", w1855) -> (resulting string=w1857:string)  [unwired: 2 in, 1 out]
        n862 = local write "Status Message"(w1857) -> ()
      }
      frame "UI: Cursor Set" {
        # "Argument"
        # "Set and Unset Cursor Busy.\n(Usage: \"UI: Cursor Set >> Busy|Idle\")"
        n863 = case shown="\"Idle\", Default" w1863 {
          tunnel: w1865 -> [w1869 w1871]
          tunnel: [w1868 w1870] -> w1864
          frame "Idle", Default {
            n864 = call <vilib>:"Unset Busy.vi"("error in (no error)"=w1869) -> ("error out"=w1868:errorcluster)  [unwired: 10 in]
          }
          frame "Busy" {
            n865 = call <vilib>:"Set Busy.vi"("error in (no error)"=w1871) -> ("error out"=w1870:errorcluster)  [unwired: 9 in, 1 out]
          }
        }
      }
      frame "UI: Front Panel State" {
        # "Argument"
        # "Set Front Panel Open or Closed\n(Usage: \"UI: Front Panel State >> Open|Close\")"
        n866 = Unbundle By Name(w1875) -> ("Core.Current VI Reference"=w1874:refnum<vi>)
        n867 = case shown="\"Minimize\", \"Minimized\"" w1873 {
          tunnel: w1877 -> [w1884 w1899 w1910 w1923 w1936]
          tunnel: [w1886 w1900 w1912 w1925 w1938] -> w1876
          tunnel: w1874 -> [w1885 w1897 w1911 w1924 w1937]
          frame "Open", "Standard", Default {
            w1879 = T16."Standard" ("State")
            n868 = property class="VI"(reference=w1885, error in=w1884) -> (reference out=w1882:refnum<vi>, error out=w1883:errorcluster, "FP.State"=w1881:T16)
            n869 = Not Equal?(x=w1881, y=w1879) -> (x != y?=w1880:bool)
            n870 = case shown="True" w1880 {
              tunnel: [w1890 w1892] -> w1886
              tunnel: w1883 -> [w1889 w1892]
              tunnel: w1882 -> [w1888 _]
              tunnel: w1879 -> [w1887 _]
              frame True {
                n871 = invoke class="VI" method="FP.Open"(reference=w1888, error in=w1889, "Activate"=TRUE, "State"=w1887) -> (error out=w1890:errorcluster)  [unwired: 1 in, 4 out]
              }
              frame False {
              }
            }
          }
          frame "Close", "Closed" {
            n872 = property class="VI"(reference=w1897, error in=w1899) -> (reference out=w1896:refnum<vi>, error out=w1898:errorcluster, "FP.State"=w1894:T16)
            n873 = Not Equal?(x=w1894, y=T16."Closed" ("Front Panel Window:State")) -> (x != y?=w1893:bool)
            n874 = case shown="True" w1893 {
              tunnel: [w1901 w1904] -> w1900
              tunnel: w1898 -> [w1901 w1903]
              tunnel: w1896 -> [_ w1902]
              frame False {
              }
              frame True {
                n875 = invoke class="VI" method="FP.Close"(reference=w1902, error in=w1903) -> (error out=w1904:errorcluster)  [unwired: 1 in, 2 out]
              }
            }
          }
          frame "Hidden", "Hide" {
            w1905 = T16."Hidden" ("State")
            n876 = property class="VI"(reference=w1911, error in=w1910) -> (reference out=w1908:refnum<vi>, error out=w1909:errorcluster, "FP.State"=w1907:T16)
            n877 = Not Equal?(x=w1907, y=w1905) -> (x != y?=w1906:bool)
            n878 = case shown="True" w1906 {
              tunnel: [w1916 w1917] -> w1912
              tunnel: w1909 -> [w1915 w1917]
              tunnel: w1908 -> [w1914 _]
              tunnel: w1905 -> [w1913 _]
              frame True {
                n879 = invoke class="VI" method="FP.Open"(reference=w1914, error in=w1915, "State"=w1913) -> (error out=w1916:errorcluster)  [unwired: 2 in, 4 out]
              }
              frame False {
              }
            }
          }
          frame "Minimize", "Minimized" {
            w1918 = T16."Minimized" ("State")
            n880 = property class="VI"(reference=w1924, error in=w1923) -> (reference out=w1921:refnum<vi>, error out=w1922:errorcluster, "FP.State"=w1920:T16)
            n881 = Not Equal?(x=w1920, y=w1918) -> (x != y?=w1919:bool)
            n882 = case shown="True" w1919 {
              tunnel: [w1929 w1930] -> w1925
              tunnel: w1922 -> [w1928 w1930]
              tunnel: w1921 -> [w1927 _]
              tunnel: w1918 -> [w1926 _]
              frame True {
                n883 = invoke class="VI" method="FP.Open"(reference=w1927, error in=w1928, "State"=w1926) -> (error out=w1929:errorcluster)  [unwired: 2 in, 4 out]
              }
              frame False {
              }
            }
          }
          frame "Maximize", "Maximized" {
            w1931 = T16."Maximized" ("State")
            n884 = property class="VI"(reference=w1937, error in=w1936) -> (reference out=w1934:refnum<vi>, error out=w1935:errorcluster, "FP.State"=w1933:T16)
            n885 = Not Equal?(x=w1933, y=w1931) -> (x != y?=w1932:bool)
            n886 = case shown="True" w1932 {
              tunnel: [w1942 w1943] -> w1938
              tunnel: w1935 -> [w1941 w1943]
              tunnel: w1934 -> [w1940 _]
              tunnel: w1931 -> [w1939 _]
              frame True {
                n887 = invoke class="VI" method="FP.Open"(reference=w1940, error in=w1941, "State"=w1939) -> (error out=w1942:errorcluster)  [unwired: 2 in, 4 out]
              }
              frame False {
              }
            }
          }
        }
      }
      frame "---------- Macro ----------" {
        # "Do not put any code in this frame.\n(It is a separator no-op. You can make a copy of this frame to create a new Macro frame)"
      }
      frame "Macro: Initialize" {
        # "Initialization Macro\n(This is called once, when the VI starts)"
        n888 = call <vilib>:"Add State(s) to Queue__jki_lib_state_machine.vi"("State(s) in Front (\"\")"="Data: Initialize\nInitialize Core Data\nUI: Initialize\nUI: Front Panel State >> Open", "State(s) in (\"\")"=w1953) -> ("States Out"=w1952:string)  [unwired: 13 in]
      }
      frame "Macro: Unreserve" {
        w1954 = FALSE ("Energize")
        # "Unreserve Macro\n(This is called when we unreserve the HPS17K)"
        n889 = local write "Energize"(w1954) -> ()
        n890 = local write "Output"(w1954) -> ()
        n891 = call <vilib>:"Add State(s) to Queue__jki_lib_state_machine.vi"("State(s) in Front (\"\")"="UI: Cursor Set >> Busy\nHPS: Output\nHPS: Energize\nHPS: Stop Measurement Stream\nHPS: Stop Setpoint Stream\nHPS: Unreserve\nScript: Stop Streamer\nUI: Cursor Set >> Idle", "State(s) in (\"\")"=w1960) -> ("States Out"=w1959:string)  [unwired: 13 in]
      }
      frame "Macro: Reserve" {
        # "Reserve Macro\n(This is called when we reserve the HPS17K)"
        n892 = call <vilib>:"Add State(s) to Queue__jki_lib_state_machine.vi"("State(s) in Front (\"\")"="UI: Cursor Set >> Busy\nHPS: Reserve\nHPS: Start Measurement Stream\nScript: Launch Streamer\nData: Update Periodic\nScript: Read Slew Rates\nScript: Read Setpoints\nScript: Read Setpoint Limits\nScript: Read Hardware Limits\nUI: Reservation Complete\nUI: Cursor Set >> Idle", "State(s) in (\"\")"=w1966) -> ("States Out"=w1965:string)  [unwired: 13 in]
      }
      frame "Macro: Connect" {
        # "Connect Macro\n(This is called when we connect to the HPS17K)"
        n893 = call <vilib>:"Add State(s) to Queue__jki_lib_state_machine.vi"("State(s) in Front (\"\")"="UI: Cursor Set >> Busy\nHPS: Connect\nScript: Launch Grapher\nEvents: Register\nUI: Connection Complete\nUI: Cursor Set >> Idle", "State(s) in (\"\")"=w1972) -> ("States Out"=w1971:string)  [unwired: 13 in]
      }
      frame "Macro: Disconnect" {
        # "Disconnect Macro\n(This is called when we disconnect from the HPS17K)"
        n894 = Unbundle By Name(w1980) -> ("Reserved"=w1979:bool, "Connected"=w1975:bool)
        n895 = Select(t="UI: Cursor Set >> Busy\nMacro: Unreserve\nScript: Stop Grapher\nHPS: Disconnect\nEvents: Unregister\nUI: Cursor Set >> Idle", s=w1979, f="UI: Cursor Set >> Busy\nScript: Stop Grapher\nHPS: Disconnect\nEvents: Unregister\nUI: Cursor Set >> Idle") -> (s? t:f=w1976:string)
        n896 = Select(t=w1976, s=w1975, f="") -> (s? t:f=w1973:string)
        n897 = call <vilib>:"Add State(s) to Queue__jki_lib_state_machine.vi"("State(s) in Front (\"\")"=w1973, "State(s) in (\"\")"=w1984) -> ("States Out"=w1983:string)  [unwired: 13 in]
      }
      frame "Macro: Start Test Server" {
        # "Start Test Server Macro\n(This is called when we start the test server on the HPS17K)"
        n898 = call <vilib>:"Add State(s) to Queue__jki_lib_state_machine.vi"("State(s) in Front (\"\")"="UI: Cursor Set >> Busy\nScript: Launch Test Server\nUI: Cursor Set >> Idle", "State(s) in (\"\")"=w1990) -> ("States Out"=w1989:string)  [unwired: 13 in]
      }
      frame "Macro: Start Self Test" {
        # "Start Self Test Macro\n(This is called when we start the self test on the HPS17K)"
        n899 = call <vilib>:"Add State(s) to Queue__jki_lib_state_machine.vi"("State(s) in Front (\"\")"="UI: Cursor Set >> Busy\nUI: Self Test Start\nScript: Start Self Test\nEvents: Register \nUI: Cursor Set >> Idle", "State(s) in (\"\")"=w1996) -> ("States Out"=w1995:string)  [unwired: 13 in]
      }
      frame "Macro: Stop Self Test" {
        # "Stop Self Test Macro\n(This is called when we start the self test on the HPS17K)"
        n900 = call <vilib>:"Add State(s) to Queue__jki_lib_state_machine.vi"("State(s) in Front (\"\")"="UI: Cursor Set >> Busy\nScript: Stop Self Test\nUI: Self Test Stop \nUI: Cursor Set >> Idle", "State(s) in (\"\")"=w2002) -> ("States Out"=w2001:string)  [unwired: 13 in]
      }
      frame "Macro: Self Test Complete" {
        # "Self Test Complete Macro\n(This is called when we the self test script has completed)"
        n901 = call <vilib>:"Add State(s) to Queue__jki_lib_state_machine.vi"("State(s) in Front (\"\")"="UI: Cursor Set >> Busy\nUI: Self Test Stop \nUI: Cursor Set >> Idle", "State(s) in (\"\")"=w2008) -> ("States Out"=w2007:string)  [unwired: 13 in]
      }
      frame "Macro: Stop Test Server" {
        # "Stop Test Server Macro\n(This is called when we stop the test server on the HPS17K)"
        n902 = call <vilib>:"Add State(s) to Queue__jki_lib_state_machine.vi"("State(s) in Front (\"\")"="UI: Cursor Set >> Busy\nScript: Stop Self Test\nScript: Stop Test Server\nUI: Cursor Set >> Idle", "State(s) in (\"\")"=w2014) -> ("States Out"=w2013:string)  [unwired: 13 in]
      }
      frame "Macro: Start Setpoint Stream" {
        # "Start Setpoint Stream Macro\n(This is called when we start the setpoint stream)"
        n903 = call <vilib>:"Add State(s) to Queue__jki_lib_state_machine.vi"("State(s) in Front (\"\")"="UI: Cursor Set >> Busy\nHPS: Start Setpoint Stream\nHPS: Update Setpoint Stream\nUI: Cursor Set >> Idle", "State(s) in (\"\")"=w2020) -> ("States Out"=w2019:string)  [unwired: 13 in]
      }
      frame "Macro: Stop Setpoint Stream" {
        # "Stop Setpoint Stream Macro\n(This is called when we stop the setpoint stream)"
        n904 = call <vilib>:"Add State(s) to Queue__jki_lib_state_machine.vi"("State(s) in Front (\"\")"="UI: Cursor Set >> Busy\nHPS: Stop Setpoint Stream\nUI: Cursor Set >> Idle", "State(s) in (\"\")"=w2026) -> ("States Out"=w2025:string)  [unwired: 13 in]
      }
      frame "Macro: Update Slew Rate" {
        # "Update Slew Rate Macro\n(This is called when we stop apply new slew rates to the HPS17K)"
        n905 = call <vilib>:"Add State(s) to Queue__jki_lib_state_machine.vi"("State(s) in Front (\"\")"="UI: Cursor Set >> Busy\nScript: Write Slew Rates\nScript: Read Slew Rates\nUI: Cursor Set >> Idle", "State(s) in (\"\")"=w2032) -> ("States Out"=w2031:string)  [unwired: 13 in]
      }
      frame "Macro: Run EIS Profile" {
        # "Run EIS Profile Macro\n(This is called after we start an EIS profile and are at steady state)"
        n906 = call <vilib>:"Add State(s) to Queue__jki_lib_state_machine.vi"("State(s) in Front (\"\")"="UI: Cursor Set >> Busy\nHPS: Start Setpoint Stream\nHPS: Update Setpoint Stream\nUI: Cursor Set >> Idle", "State(s) in (\"\")"=w2038) -> ("States Out"=w2037:string)  [unwired: 13 in]
      }
      frame "Macro: Start EIS Profile" {
        w2039 = TRUE ("Energize")
        w2048 = T6 2 items=["Constant Voltage"=1, "Constant Current"=2, "Internal Recirculation"=193] ("Mode")
        w2051 = T10 1 items=["Voltage (PEIS)"=1, "Current (GEIS)"=2] ("y")
        w2050 = T6 1 items=["Constant Voltage"=1, "Constant Current"=2, "Internal Recirculation"=193] ("Mode")
        # "Start EIS Profile Macro\n(This is called when we start an EIS profile on the HPS-17K)"
        n907 = local read "EIS DC Potential"() -> (w2044:dbl)
        n908 = local read "EIS DC Current"() -> (w2042:dbl)
        n909 = local read "EIS Mode"() -> (w2052:T10)
        n910 = Equal?(x=w2052, y=w2051) -> (x = y?=w2049:bool)
        n911 = local read "Mode & Range"() -> (w2053:cluster{"Mode":T6, "Range":T7})
        n912 = local read "Setpoints"() -> (w2045:T5)
        n913 = To Single Precision Float(number=w2044) -> (single precision float=w2043:sgl)
        n914 = To Single Precision Float(number=w2042) -> (single precision float=w2041:sgl)
        n915 = Select(t=w2050, s=w2049, f=w2048) -> (s? t:f=w2047:T6)
        n916 = Bundle By Name(cluster=w2045, "Voltage"=w2043, "Current"=w2041) -> (w2040:T5)
        n917 = Bundle By Name(cluster=w2053, "Mode"=w2047) -> (w2046:cluster{"Mode":T6, "Range":T7})
        n918 = local write "Mode & Range"(w2046) -> ()
        n919 = local write "Setpoints"(w2040) -> ()
        n920 = local write "Energize"(w2039) -> ()
        n921 = local write "Output"(w2039) -> ()
        n922 = call <vilib>:"Add State(s) to Queue__jki_lib_state_machine.vi"("State(s) in Front (\"\")"="UI: Cursor Set >> Busy\nHPS: Set Mode and Range\nHPS: Apply Setpoints\nHPS: Energize\nHPS: Output\nEIS: Wait for Steady State\nEvents: Register\nUI: Cursor Set >> Idle", "State(s) in (\"\")"=w2059) -> ("States Out"=w2058:string)  [unwired: 13 in]
      }
      frame "Macro: Exit" {
        # "Exit Macro\n(This is called once, when the VI exits)"
        n923 = Unbundle By Name(w2067) -> ("Core.Close Panel on Exit?"=w2063:bool)
        n924 = call <vilib>:"Conditional State String__jki_lib_state_machine.vi"("Do State(s)?"=w2063, "State"="UI: Front Panel State >> Close") -> ("State Out"=w2062:string)  [unwired: 7 in]
        n925 = call <vilib>:"Add State(s) to Queue__jki_lib_state_machine.vi"("State(s) in (\"\")"=w2062, "State(s) at Back (\"\")"="Script: Stop Self Test\nScript: Stop Test Server\nScript: Stop Streamer\nScript: Stop Logger\nUI: Uninitialize\nData: Cleanup\nMacro: Disconnect\nExit") -> ("States Out"=w2065:string)  [unwired: 13 in]
        n926 = call <vilib>:"Add State(s) to Queue__jki_lib_state_machine.vi"("State(s) in Front (\"\")"=w2065, "State(s) in (\"\")"=w2069) -> ("States Out"=w2068:string)  [unwired: 13 in]
      }
    }
  }
  n927 = disable-structure shown="Disabled" {
    frame Disabled {
      n928 = invoke on="EIS Subpanel" class="SubPnl" method="Insert VI"() -> ()  [unwired: 4 in, 4 out]
    }
    frame Enabled {
    }
  }
